vi "高压板校准程序1.2.vi"(8 "波特率":T3(ring)=enum."500Kbps", 9 "CAN路数":u16(ring) items=["0", "1"], 10 "设备索引":u16(ring) items=["0", "1", "2", "3", "4", "5", "6", "7", "8", "9", "10", "11", "12", "13", "14", "15", ""], 11 "CAN卡类型":u32(ring)=21 items=["PCI5121"=1, "PCI9810"=2, "USBCAN1"=3, "USBCAN2"=4, "PCI9820"=5, "PCI5110"=7, "CANLite(mini)"=8, "ISA9620"=9, "ISA5420"=10, "PC104CAN"=11, "DNP9810"=13, "PCI9840B"=14, "PC104C2"=15, "PCI9820I"=16, "pec9920"=18, "USBCAN_E_U"=20, "USBCAN_2E_U"=21]) -> (6 "E-U_baud":u32(ring)=393223 items=["0x060003--1000Kbps"=393219, "0x060004--800Kbps"=393220, "0x060007--500Kbps"=393223, "0x1C0008--250Kbps"=1835016, "0x1C0011--125Kbps"=1835025, "0x160023--100Kbps"=1441827, "0x1C002C--50Kbps"=1835052, "0x1600B3--20Kbps"=1441971, "0x1C00E0--10Kbps"=1835232, "0x1C01C1--5Kbps"=1835457])   [LabVIEW 2013]
uses:
  <vilib>/Instr/_visa.llb/VISA Configure Serial Port (Instr).vi
  <vilib>/Utility/config.llb/Write Key (String).vi
  <vilib>/Utility/file.llb/Read From Spreadsheet File (string).vi
  <vilib>/Utility/file.llb/Write To Spreadsheet File (string).vi
  <vilib>/Utility/config.llb/NI_LVConfig.lvlib
  data/kerneldlls/usbcan.dll
panel:
  in  "输出簇":T1
  out "Life":dbl
  out "分流器":enum32{"选项卡 1"}(tab)
  out "外总压":enum32{"选项卡 1"}(tab)
  out "内总压":enum32{"选项卡 1"}(tab)
  out "电流校正 2":enum32{"选项卡 1"}(tab)
  out "电流校正":enum32{"选项卡 1"}(tab)
  in  "Judge(%)":dbl=1.0
  in  "Judge(%)":dbl=0.5
  in  "记录":bool
  out "结果":i32(listbox)=-1
  in  "一键校正":bool
  in  "刷新":bool
  in  "分流器大小":T2(ring)=enum."300A"
  out "监控状态":bool
  out "电流":dbl format="%#.6f"
  out "外总压":dbl format="%#.6f"
  out "内总压":dbl format="%#.6f"
  in  "平均电压":dbl
  in  "电压增益":dbl
  in  "平均电流":dbl
  in  "电流增益":dbl
  in  "放电能量阀值":dbl=375.0
  in  "充电能量阀值":dbl=375.0
  in  "分流器型号":bool
  out "Current Gain结果 4":bool
  in  "充电能量阀值":bool
  out "Current Offset结果 4":bool
  in  "Set Current Gain 3":bool
  out "Current Gain结果 3":bool
  in  "Set Current Offset 3":bool
  out "Current Offset结果 3":bool
  out "Shunt Volt Gain":string
  out "Shunt Volt Offset":string
  in  "Set Current Gain 2":bool
  out "Current Gain结果 2":bool
  in  "Volt Offset":bool
  out "Current Offset结果 2":bool
  in  "导入配置结果":bool
  in  "读版本结果":bool
  in  "写版本结果":bool
  out "版本号-读":string
  in  "版本号":string
  in  "写配置文件版本":bool
  in  "读配置文件版本":bool
  in  "生成配置":bool
  in  "导入配置":bool
  out "config_data":string="000124FE00264205"
  out "充放电阈值":dbl=75006.0
  in  "连接状态 10":bool
  in  "设置参数":bool
  in  "安时分辨率/AH":u16(ring)=1 items=["0.001", "0.2"]
  in  "是否有外部高压":u16(ring)=1 items=["有", "无"]
  in  "分流器大小/A":u16(ring)=3 items=["50", "100", "200", "300", "400", "500", "600", "700", "800", "900", "1000"]
  in  "传感器类型":u16(ring)=1 items=["霍尔传感器", "分流器"]
  in  "电压分辨率/V":u16(ring)=1 items=["0.01", "0.1"]
  in  "电流分辨率/A":u16(ring)=1 items=["0.01", "0.1"]
  in  "Set":dbl
  in  "Volt2":dbl=300.0
  in  "Volt1":dbl=150.0
  in  "Clear":bool
  out "Clear结果":bool
  out "电流增益":string
  out "电流零点":string
  in  "Read1_in":bool
  out "Read1_in结果":bool
  in  "REAL1":dbl=150.0
  out "AD1":dbl
  in  "REAL2":dbl=300.0
  out "AD2":dbl
  in  "Offset":i32 format="%x"
  in  "Gain":dbl
  in  "REAL1":dbl=150.0
  in  "AD1":dbl
  in  "REAL2":dbl=300.0
  in  "AD2":dbl
  in  "Offset":i32 format="%x"
  in  "Gain":dbl
  in  "Read2_in":bool
  out "Read2_in结果":bool
  in  "Set_in":bool
  out "Set_in结果":bool
  in  "Read1_Out":bool
  out "Read1_Out结果":bool
  in  "Read2_Out":bool
  out "Read2_Out结果":bool
  in  "Set_out":bool
  out "Set_out结果":bool
  in  "Read1":bool
  out "Read1结果":bool
  in  "REAL1":dbl=40.0
  out "AD1":u16
  in  "REAL2":dbl=80.0
  out "AD2":u16
  in  "Gain":dbl
  in  "Read2":bool
  out "Read2结果":bool
  in  "Set":bool
  out "Set结果":bool
  in  "Set Current Gain":bool
  out "Current Gain结果":bool
  in  "Set Current Offset":bool
  out "Current Offset结果":bool
  in  "Clear_out":bool
  out "Clear_out结果":bool
  in  "Clear_in":bool
  out "Clear_in结果":bool
  in  "输出自定义值1":bool
  in  "输出自定义值2":bool
  out "Actual":dbl format="%#.6f"
  out "Set":dbl format="%#.6f"
  out "Actual":dbl
  in  "连接电压源":bool
  out "连接状态 10":bool
  in  "VISA resource name 4":refnum<visa-resource-name>="COM1" caption="设备端口号"
  in  "工作方式":u8(ring) items=["Normal", "Listen Only"]
  in  "滤波方式":u8(ring) items=["Dual Filter", "Single Filter"]
  out "CAN连接状态":bool
  in  "启动CAN连接":bool
  in  "VISA resource name 2":refnum<visa-resource-name>="GPIB0::5::INSTR" caption="设备端口号"
  out "连接状态 10":bool
  in  "连接GPIB":bool
  in  "Curr1":dbl=40.0
  in  "输出自定义值1 2":bool
  in  "输出自定义值2 2":bool
  in  "Curr2":dbl=80.0
  in  "退出":bool
  out "设置中？ 2":bool
  out "CAN状态 3":bool
  in  "设备索引 3":u16(ring) items=["0", "1", "2", "3", "4", "5", "6", "7", "8", "9", "10", "11", "12", "13", "14", "15", ""]
  in  "CAN路数 3":u16(ring) items=["0", "1"]
  in  "设备类型 3":u16(ring)=4 items=["PCI5121"=1, "PCI9810"=2, "USBCAN1"=3, "USBCAN2"=4, "PCI9820"=5, "CAN232"=6, "PCI5110"=7, "CANLite(mini)"=8, "ISA9620"=9, "ISA5420"=10, "PC104CAN"=11, "CANETE"=12, "DNP9810"=13]
  out "CAN 3":bool
  in  "停止 2":bool=TRUE
  out "监控 4":bool
  out "x-y":u32
  in  "退出程序 2":bool
  in  "error in (no error)":errorcluster caption="错误输入（无错误）"
  in  "控制读取  2":bool
  out "VISA资源名称输出":refnum<visa-resource-name>="0"
  in  "退出程序 3":bool
  in  "输出200A":bool
  out "实际值 2":dbl
  out "设定值 2":dbl
  in  "输出100A":bool
  in  "停止 7":bool=TRUE
  in  "分辨率偏移值 4":T4={"主板总电压分辨率"=0.01, "主板总电压偏移量"=0.0, "主板总电流分辨率"=0.01, "主板总电流偏移量"=-300.0, "主板安时分辨率"=0.2, "主板安时偏移量"=0.0, "主板SOC分辨率"=0.4, "主板SOC偏移量"=0.0, "从板总电压分辨率"=0.01, "从板总电压偏移量"=0.0, "从板总电流分辨率"=0.01, "从板总电流偏移量"=0.0, "从板安时分辨率"=0.2, "从板安时偏移量"=0.0, "从板SOC分辨率"=0.4, "从板SOC偏移量"=0.0, "功率分辨率"=0.01, "功率偏移量"=-300.0, "单体电压分辨率 "=0.0001, "单体电压偏移量"=0.0, "温度分辨率"=1.0, "温度偏移量"=-40.0, "高压板总电压分辨率"=0.01, "高压板总电压偏移量"=0.0, "高压板总电流分辨率"=0.01, "高压板总电流偏移量"=-300.0, "高压板安时分辨率"=0.2, "高压板安时偏移量"=0.0, "高压板SOC分辨率"=0.4, "高压板SOC偏移量"=0.0, "高压板功率分辨率"=0.01, "高压板功率偏移量"=-300.0}
  in  "分辨率偏移值 3":T4={"主板总电压分辨率"=0.01, "主板总电压偏移量"=0.0, "主板总电流分辨率"=0.01, "主板总电流偏移量"=-300.0, "主板安时分辨率"=0.2, "主板安时偏移量"=0.0, "主板SOC分辨率"=0.4, "主板SOC偏移量"=0.0, "从板总电压分辨率"=0.01, "从板总电压偏移量"=0.0, "从板总电流分辨率"=0.01, "从板总电流偏移量"=0.0, "从板安时分辨率"=0.2, "从板安时偏移量"=0.0, "从板SOC分辨率"=0.4, "从板SOC偏移量"=0.0, "功率分辨率"=0.01, "功率偏移量"=-300.0, "单体电压分辨率 "=0.0001, "单体电压偏移量"=0.0, "温度分辨率"=1.0, "温度偏移量"=-40.0, "高压板总电压分辨率"=0.01, "高压板总电压偏移量"=0.0, "高压板总电流分辨率"=0.01, "高压板总电流偏移量"=-300.0, "高压板安时分辨率"=0.2, "高压板安时偏移量"=0.0, "高压板SOC分辨率"=0.4, "高压板SOC偏移量"=0.0, "高压板功率分辨率"=0.01, "高压板功率偏移量"=-300.0}
  in  "监控":bool
  out "VCI_CAN_OBJ_R 2":T5={"ID"=0, "TimeStamp"=0, "TimeFlag"=0, "SendType"=1, "RemoteFlag"=0, "ExternFlag"=0, "DataLen"=8, 0, 0, 0, 0, 0, 0, 0, 0, 0, 0, 0}
  in  "分辨率偏移值":T6
  out "允许读取":bool
  out "设置中？":bool
  out "CAN状态 2":bool=TRUE
  in  "设备索引 2":u16(ring) items=["0", "1", "2", "3", "4", "5", "6", "7", "8", "9", "10", "11", "12", "13", "14", "15", ""]
  in  "CAN路数 2":u16(ring) items=["0", "1"]
  in  "设备类型 2":u16(ring)=4 items=["PCI5121"=1, "PCI9810"=2, "USBCAN1"=3, "USBCAN2"=4, "PCI9820"=5, "CAN232"=6, "PCI5110"=7, "CANLite(mini)"=8, "ISA9620"=9, "ISA5420"=10, "PC104CAN"=11, "CANETE"=12, "DNP9810"=13]
  out "CAN 2":bool
  in  "监控 2":bool
  in  "停止 6":bool=TRUE
  out "接收":T5={"ID"=67239966, "TimeStamp"=241409471, "TimeFlag"=1, "SendType"=250, "RemoteFlag"=0, "ExternFlag"=1, "DataLen"=8, 0, 0, 117, 48, 117, 48, 0, 0, 0, 0, 124} {"ID" format="%x"}
  in  "高压板信息":T7={"内部高压/V"=0.0, "Life"=10.0, "外部高压/V"=0.0, "power/KW"=0.0, "current/A"=0.0, "error code"=1, "SOC/%"=0.0, "总充电安时/AH"=0.0, "总放电安时/AH"=0.0, "平均电压"=0.0} {"平均电压" format="%.3f"; "总放电安时/AH" format="%#.3f"; "总充电安时/AH" format="%#.3f"; "SOC/%" format="%.3g"; "error code" format="%x"; "current/A" format="%.3g"; "power/KW" format="%#.3f"; "外部高压/V" format="%.3g"; "内部高压/V" format="%.3g"}
  in  "控制读取  5":bool
  out "VISA资源名称输出 10":refnum<visa-resource-name>
  in  "输出300V":bool
  out "电流/A 4":dbl
  in  "输出150V":bool
  in  "停止 3":bool=TRUE
  out "error out 3":errorcluster caption="error out"
  in  "错误输入（无错误）":errorcluster
  in  "控制读取  2":bool
  out "VISA资源名称输出 9":refnum<visa-resource-name>
  in  "退出程序":bool
  in  "输出80A":bool
  in  "输出40A":bool
  in  "控制读取  4":bool
  out "VISA资源名称输出 8":refnum<visa-resource-name>
  in  "连接状态 7":bool
  out "error out 2":errorcluster caption="error out"
  in  "控制读取  2":bool
  in  "连接状态 6":bool
  in  "控制读取  3":bool
  out "VISA资源名称输出 6":refnum<visa-resource-name>
  out "error out":errorcluster
  in  "控制读取  2":bool
  out "VISA资源名称输出 5":refnum<visa-resource-name>
  in  "电流值":dbl
  in  "自动控制仪器":bool=TRUE
  out "VISA资源名称输出 4":refnum<visa-resource-name>
  out "VISA资源名称输出 3":refnum<visa-resource-name>
  out "实际值 3":dbl format="%#.6f"
  out "设定值":dbl format="%#.6f"
  in  "控制读取  2":bool
  out "电流/A":dbl
  in  "控制读取":bool
  in  "Boar_Type":bool
  out "temp1":bool
  in  "总步骤":dbl=21.0
  in  "NG重测次数":dbl=3.0
  out "一键测试":bool
  out "测试结果":bool=TRUE
  in  "行号":dbl
  out "CAN状态":bool=TRUE
  out "CAN":bool
  in  "监控":bool=TRUE
  out "VCI_CAN_OBJ_R":T5={"ID"=0, "TimeStamp"=0, "TimeFlag"=0, "SendType"=1, "RemoteFlag"=0, "ExternFlag"=0, "DataLen"=8, 0, 0, 0, 0, 0, 0, 0, 0, 0, 0, 0}
  in  "停止":bool=TRUE
  # "重要参数设置"
  # "A"
  # "V"
  # "监控上位机"
  # "内总压"
  # "电流增益"
  # "AD2=AD1*2"
  # "外总压"
  # "BCU实时信息："
  # "BMS_Monitor"
  # "分辩率"
  # "偏移量"
  # "分辩率"
  # "偏移量"
  # "分辩率"
  # "偏移量"
  # "分辩率"
  # "偏移量"
  # "分辩率"
  # "偏移量"
  # "分辩率"
  # "偏移量"
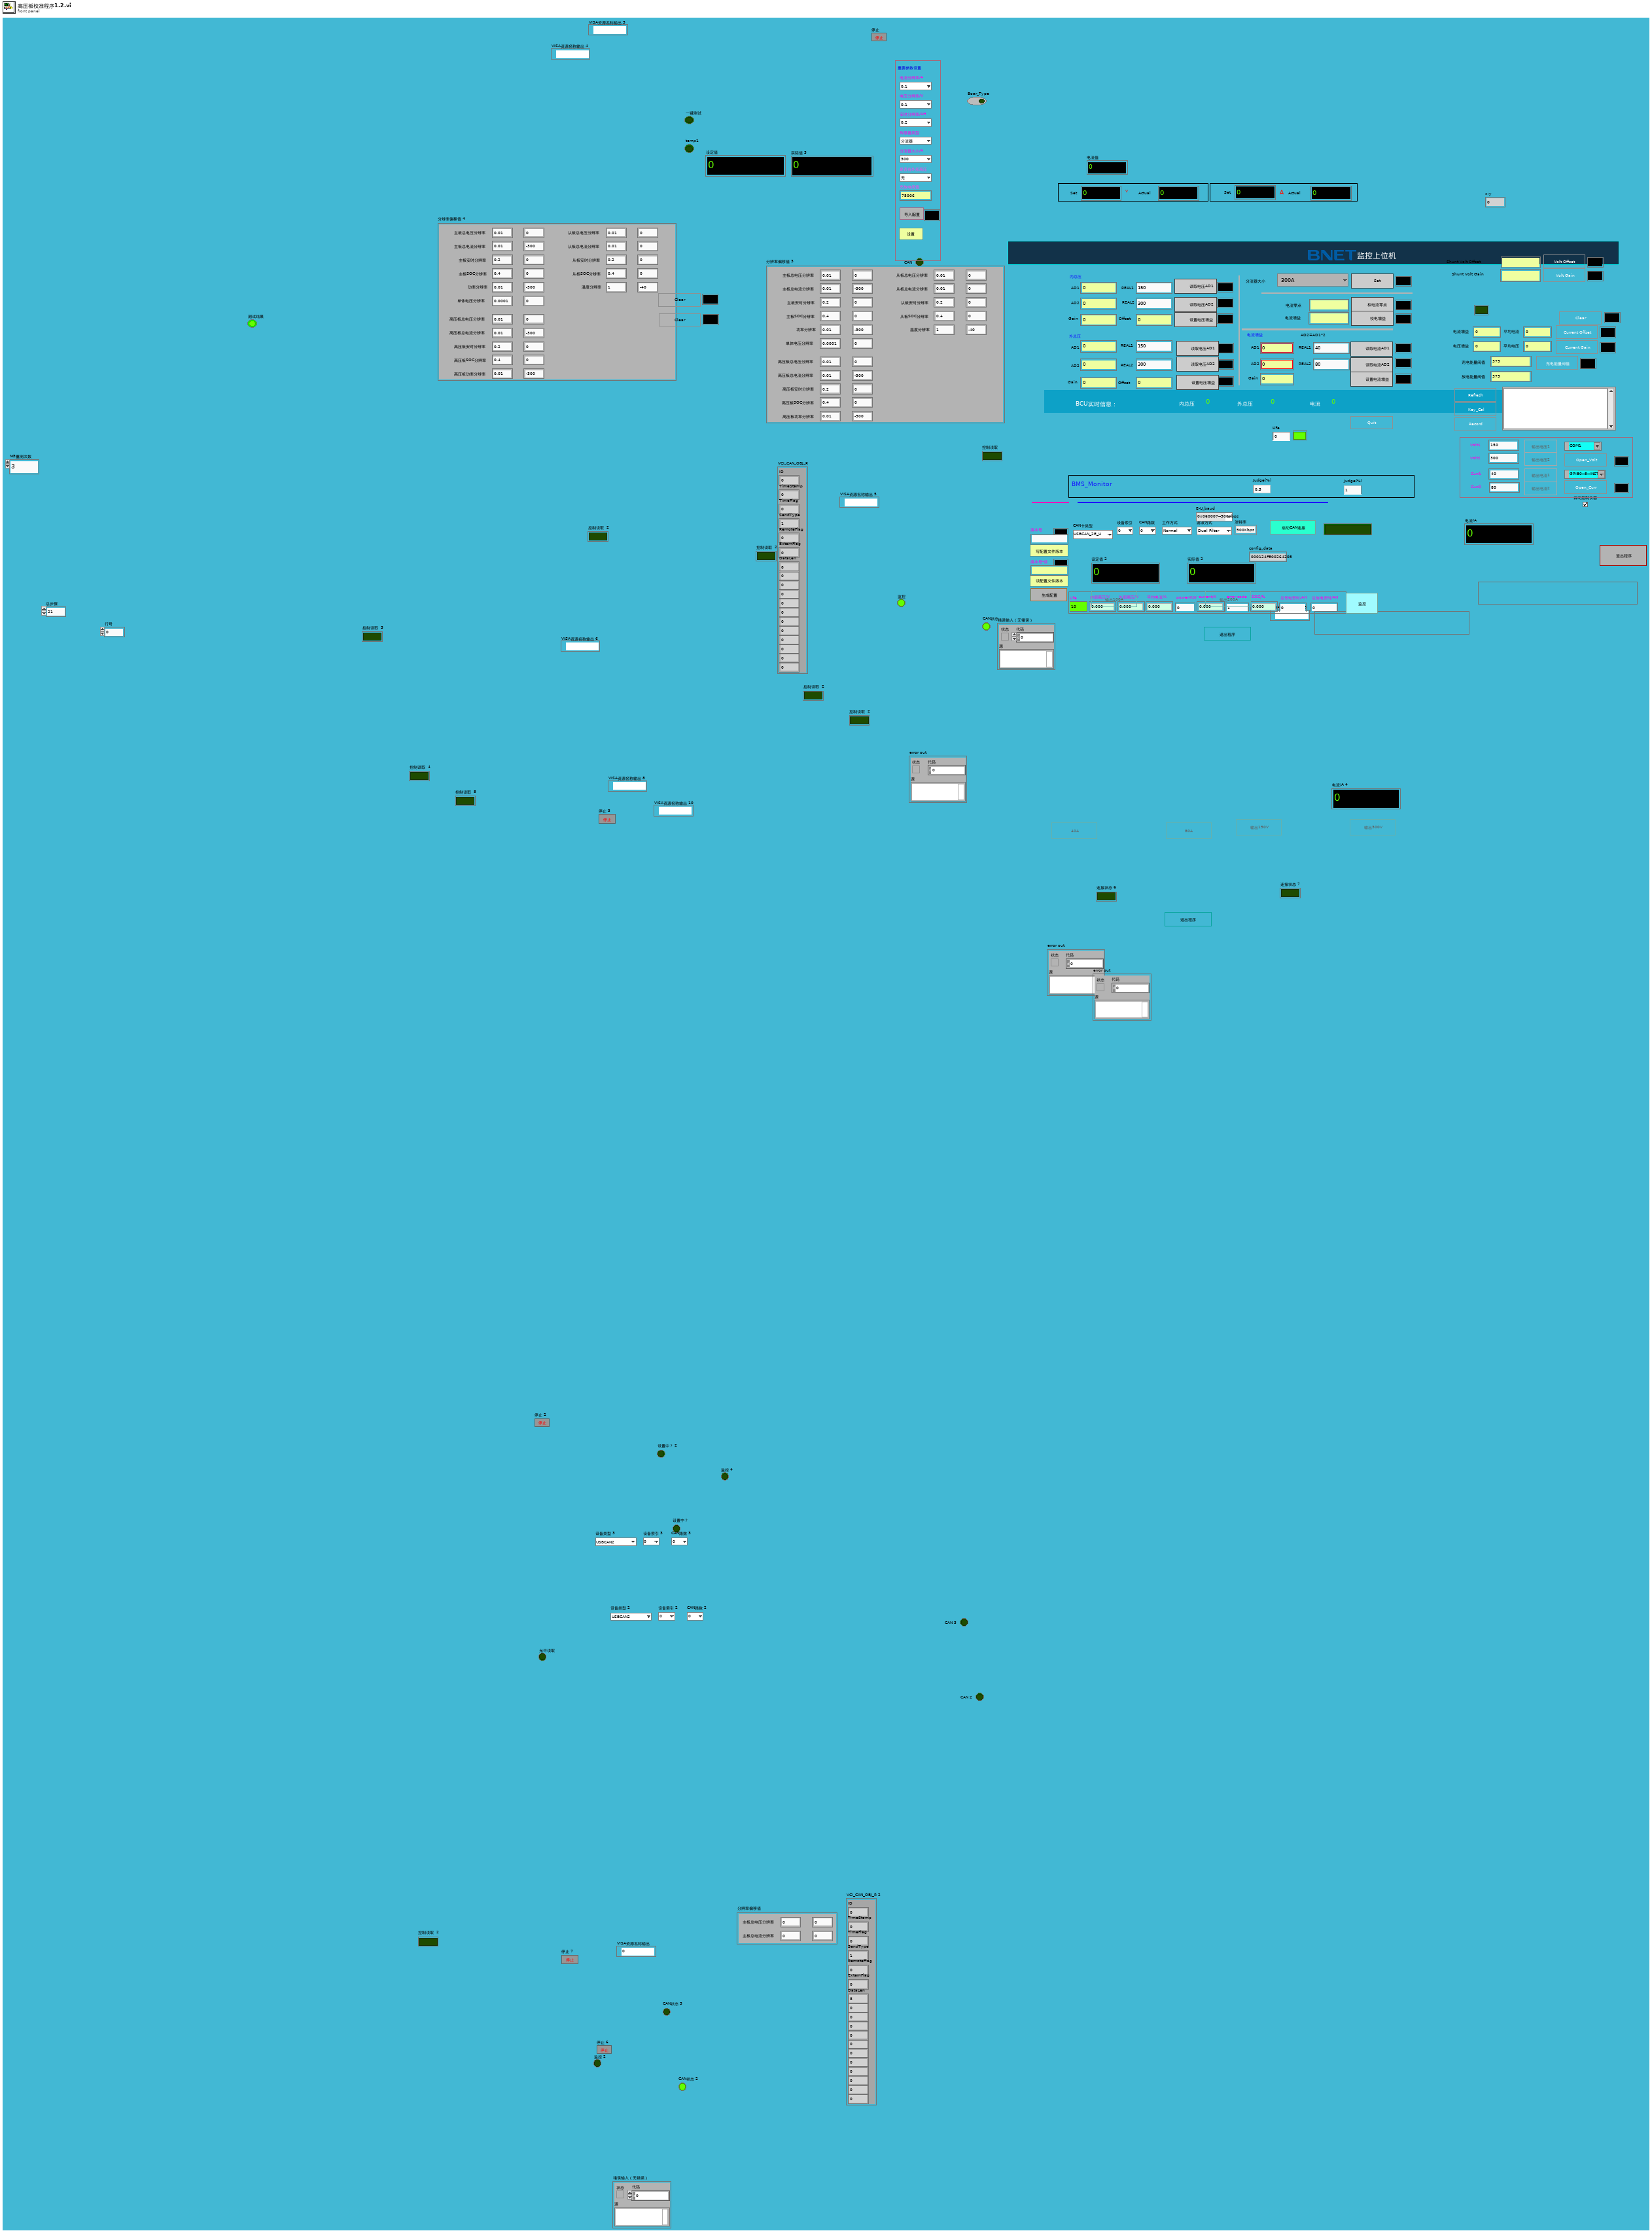
[diagram p1: front panel]
types:
  T1 = cluster{"return type":u32, "pReceive":cluster{"ID":u32, "TimeStamp":u32, "TimeFlag":u8, "SendType":u8, "RemoteFlag":u8, "ExternFlag":u8, "DataLen":u8, u8, u8, u8, u8, u8, u8, u8, u8, u8, u8, u8}[]}
  T2 = enum16{"选择分流器型号", "100A", "200A", "300A", "400A", "500A", "600A", "700A", "800A", "900A", "1000A"}
  T3 = enum16{"5Kbps", "10Kbps", "20Kbps", "40Kbps", "50Kbps", "80Kbps", "100Kbps", "125Kbps", "200Kbps", "250Kbps", "400Kbps", "500Kbps", "666Kbps", "800Kbps", "1000Kbps"}
  T4 = cluster{"主板总电压分辨率":dbl, "主板总电压偏移量":dbl, "主板总电流分辨率":dbl, "主板总电流偏移量":dbl, "主板安时分辨率":dbl, "主板安时偏移量":dbl, "主板SOC分辨率":dbl, "主板SOC偏移量":dbl, "从板总电压分辨率":dbl, "从板总电压偏移量":dbl, "从板总电流分辨率":dbl, "从板总电流偏移量":dbl, "从板安时分辨率":dbl, "从板安时偏移量":dbl, "从板SOC分辨率":dbl, "从板SOC偏移量":dbl, "功率分辨率":dbl, "功率偏移量":dbl, "单体电压分辨率 ":dbl, "单体电压偏移量":dbl, "温度分辨率":dbl, "温度偏移量":dbl, "高压板总电压分辨率":dbl, "高压板总电压偏移量":dbl, "高压板总电流分辨率":dbl, "高压板总电流偏移量":dbl, "高压板安时分辨率":dbl, "高压板安时偏移量":dbl, "高压板SOC分辨率":dbl, "高压板SOC偏移量":dbl, "高压板功率分辨率":dbl, "高压板功率偏移量":dbl}
  T5 = cluster{"ID":u32, "TimeStamp":u32, "TimeFlag":u8, "SendType":u8, "RemoteFlag":u8, "ExternFlag":u8, "DataLen":u8, u8, u8, u8, u8, u8, u8, u8, u8, u8, u8, u8}
  T6 = cluster{"主板总电压分辨率":dbl, "主板总电压偏移量":dbl, "主板总电流分辨率":dbl, "主板总电流偏移量":dbl, "主板安时分辨率":dbl, "主板安时偏移量":dbl, "主板SOC分辨率":dbl, "主板SOC偏移量":dbl, "从板总电压分辨率":dbl, "从板总电压偏移量":dbl, "从板总电流分辨率":dbl, "从板总电流偏移量":dbl, "从板安时分辨率":dbl, "从板安时偏移量":dbl, "从板SOC分辨率":dbl, "从板SOC偏移量":dbl, "功率分辨率":dbl, "功率偏移量":dbl, "单体电压分辨率 ":dbl, "单体电压偏移量":dbl, "温度分辨率":dbl, "温度偏移量":dbl}
  T7 = cluster{"内部高压/V":dbl, "Life":dbl, "外部高压/V":dbl, "power/KW":dbl, "current/A":dbl, "error code":u32, "SOC/%":dbl, "总充电安时/AH":dbl, "总放电安时/AH":dbl, "平均电压":dbl}
  T8 = enum16{"Set Current Offset", "Set Current Gain 4", "Set Current Gain", "Set Volt offset", "Set Volt Gain", "Set Current Offset 3", "Set Current Gain 3", "Set Current Offset 4", "Read", "Set", "Clear", "Read_in", "Set_in", "Clear_in", "Read_out", "Set_out", "Clear_out", "参数设置", "写配置文件版本", "读配置文件版本"}
  T9 = enum16{"Set Current Offset", "Set Current Gain", "Read", "Set", "Clear", "Read_in", "Set_in", "Clear_in", "Read_out", "Set_out", "Clear_out", "参数设置", "写配置文件版本", "读配置文件版本"}
  T10 = enum16{"Set Current Offset", "Set Current Gain", "Read", "Set", "Clear", "Read_in", "Set_in", "Clear_in", "Read_out", "Set_out", "Clear_out"}
  T11 = cluster{"ID":u32, "TimeStamp":u32, "TimeFlag":u8, "SendType":u8, "RemoteFlag":u8, "ExternFlag":u8, "DataLen":u8, u8, u8, u8, u8, u8, u8, u8, u8, u8, u8, u8}[]
  T12 = enum32{"Invalid", "Standard", "Closed", "Hidden", "Minimized", "Maximized"}
  T13 = typedef "NI_LVConfig.lvlib/Config Data RefNum.ctl" = refnum<k1>
  T14 = cluster{"return type":u32, "pReceive":cluster{"ID":u32, "TimeStamp":u32, "TimeFlag":u8, "SendType":u8, "RemoteFlag":u8, "ExternFlag":u8, "DataLen":u8, "1":u8, "2":u8, "3":u8, "4":u8, "5":u8, "6":u8, "7":u8, "8":u8, "9":u8, "10":u8, "11":u8}[]}
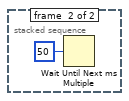
[diagram p4: hidden frame]
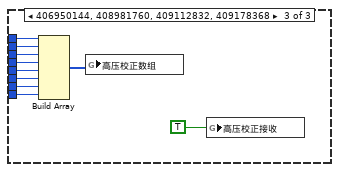
[diagram p6: hidden frame]
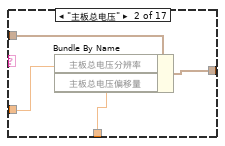
[diagram p9: hidden frame]
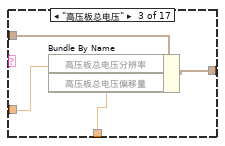
[diagram p10: hidden frame]
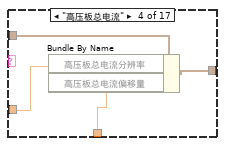
[diagram p11: hidden frame]
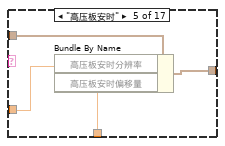
[diagram p12: hidden frame]
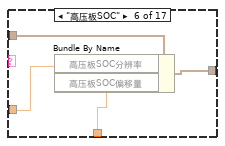
[diagram p13: hidden frame]
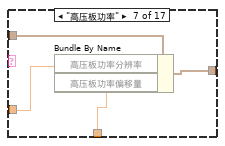
[diagram p14: hidden frame]
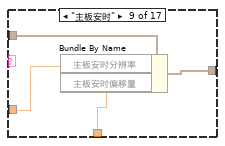
[diagram p15: hidden frame]
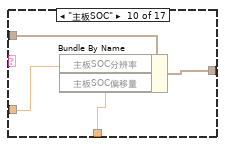
[diagram p16: hidden frame]
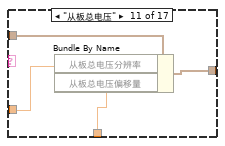
[diagram p17: hidden frame]
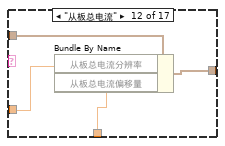
[diagram p18: hidden frame]
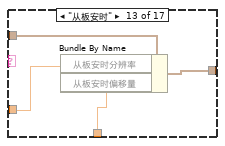
[diagram p19: hidden frame]
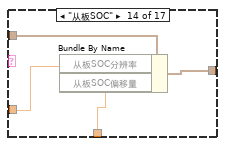
[diagram p20: hidden frame]
diagram:
  w18 = u32 0
  w35 = FALSE ("停止")
  w39 = u16 1 items=["霍尔传感器", "分流器"] ("传感器类型")
  w37 = cluster{u32, u32}[] [{0, 0}] ("颜色[4]")
  w36 = "" ("布尔文本.文本")
  w50 = u8 2 ("禁用")
  w46 = 0.0 ("电流/A")
  (unwired) "SET:GRO 1,10,1,1,0,0,0" ("写入缓冲区")
  w61 = u8 2 ("禁用")
  w45 = u8 2 ("禁用")
  (unwired) "SET:GRO 1,10,1,1,0,0,0" ("写入缓冲区")
  w68 = u8 0 ("禁用")
  w24 = cluster{u32, u32}[] [{0, 0}] ("颜色[4]")
  w23 = "" ("布尔文本.文本")
  (unwired) u8 2 ("禁用")
  (unwired) 20
  (unwired) u8 2 ("禁用")
  w69 = "Cmd" ("名称（未命名）")
  n1 = disable-structure shown="禁用" {
    frame Disabled {
      n2 = call "getpath.vi"() -> ("stripped path"=w77:path)  [unwired: 11 out]
      n3 = local read "分辨率偏移值 3"() -> (w74:T4)
      n4 = Build Path(base path=w77, name or relative path="Settings\\300以下分辨率偏移值.xls" ("名称或相对路径")) -> (appended path=w81:path)
      n5 = call-poly <vilib>:"Read From Spreadsheet File.vi"("file path (dialog if empty)"=w81) -> ("all rows"=w78:string[][])  [unwired: 3 in, 7 out]
      n6 = Delete From Array(array=w78, length=1 ("长度"), index (row)=0 ("索引")) -> (array with subset deleted=w75:string[][])  [unwired: 1 in, 1 out]
      n7 = for {
        tunnel: w75 -> [w90] mode=indexing
        shift-right: [w82] -> w73
        shift-left: w74 -> [w87]
        n8 = Index Array(array=w90, index #1=0 ("索引")) -> (element #1=w88:string, element #2=w86:string, element #3=w84:string)  [unwired: 2 in]
        n9 = Fract/Exp String To Number(string=w86) -> (number=w85:dbl)  [unwired: 4 out]
        n10 = Fract/Exp String To Number(string=w84) -> (number=w83:dbl)  [unwired: 4 out]
        n11 = case shown="\"主板总电流\"" w88 {
          tunnel: w87 -> [w91 w95 w99 w103 w107 w111 w115 w119 w123 w127 w131 w135 w139 w143 w147 w151 w155]
          tunnel: [w91 w94 w98 w102 w106 w110 w114 w118 w122 w126 w130 w134 w138 w142 w146 w150 w154] -> w82
          tunnel: w85 -> [_ w93 w97 w101 w105 w109 w113 w117 w121 w125 w129 w133 w137 w141 w145 w149 w153]
          tunnel: w83 -> [_ w92 w96 w100 w104 w108 w112 w116 w120 w124 w128 w132 w136 w140 w144 w148 w152]
          frame "假", Default {
          }
          frame "主板总电压" {
            n12 = Bundle By Name(cluster=w95, "主板总电压分辨率"=w93, "主板总电压偏移量"=w92) -> (w94:T4)
          }
          frame "高压板总电压" {
            n13 = Bundle By Name(cluster=w99, "高压板总电压分辨率"=w97, "高压板总电压偏移量"=w96) -> (w98:T4)
          }
          frame "高压板总电流" {
            n14 = Bundle By Name(cluster=w103, "高压板总电流分辨率"=w101, "高压板总电流偏移量"=w100) -> (w102:T4)
          }
          frame "高压板安时" {
            n15 = Bundle By Name(cluster=w107, "高压板安时分辨率"=w105, "高压板安时偏移量"=w104) -> (w106:T4)
          }
          frame "高压板SOC" {
            n16 = Bundle By Name(cluster=w111, "高压板SOC分辨率"=w109, "高压板SOC偏移量"=w108) -> (w110:T4)
          }
          frame "高压板功率" {
            n17 = Bundle By Name(cluster=w115, "高压板功率分辨率"=w113, "高压板功率偏移量"=w112) -> (w114:T4)
          }
          frame "主板总电流" {
            n18 = Bundle By Name(cluster=w119, "主板总电流分辨率"=w117, "主板总电流偏移量"=w116) -> (w118:T4)
          }
          frame "主板安时" {
            n19 = Bundle By Name(cluster=w123, "主板安时分辨率"=w121, "主板安时偏移量"=w120) -> (w122:T4)
          }
          frame "主板SOC" {
            n20 = Bundle By Name(cluster=w127, "主板SOC分辨率"=w125, "主板SOC偏移量"=w124) -> (w126:T4)
          }
          frame "从板总电压" {
            n21 = Bundle By Name(cluster=w131, "从板总电压分辨率"=w129, "从板总电压偏移量"=w128) -> (w130:T4)
          }
          frame "从板总电流" {
            n22 = Bundle By Name(cluster=w135, "从板总电流分辨率"=w133, "从板总电流偏移量"=w132) -> (w134:T4)
          }
          frame "从板安时" {
            n23 = Bundle By Name(cluster=w139, "从板安时分辨率"=w137, "从板安时偏移量"=w136) -> (w138:T4)
          }
          frame "从板SOC" {
            n24 = Bundle By Name(cluster=w143, "从板SOC分辨率"=w141, "从板SOC偏移量"=w140) -> (w142:T4)
          }
          frame "温度" {
            n25 = Bundle By Name(cluster=w147, "温度分辨率"=w145, "温度偏移量"=w144) -> (w146:T4)
          }
          frame "功率" {
            n26 = Bundle By Name(cluster=w151, "功率分辨率"=w149, "功率偏移量"=w148) -> (w150:T4)
          }
          frame "单体电压" {
            n27 = Bundle By Name(cluster=w155, "单体电压分辨率"=w153, "单体电压偏移量"=w152) -> (w154:T4)
          }
        }
      }
      n28 = local write "分辨率偏移值 3"(w73) -> ()
    }
    frame Enabled {
    }
  }
  n29 = stacked-sequence {
    tunnel: [w157 _] -> w19
    frame #0 {
      n30 = global read "EV05全局变量1.vi" "设备索引号"() -> (w159:u16)
      n31 = global read "EV05全局变量1.vi" "CAN卡类型"() -> (w160:u32)
      n32 = global read "EV05全局变量1.vi" "CAN端口"() -> (w158:u16)
      n33 = Build Array(1) -> (w161:i32[])
      n34 = call "transmit-8.6.vi"("can卡类型"=w160, "设备索引号"=w159, "CAN端口"=w158, "ID"=418398080, "SendType"=u8 0, "Data"=w161) -> ("错误输出"=w157:errorcluster)  [unwired: 3 in, 10 out]
    }
    frame #1 {
      n35 = Wait Until Next ms Multiple(millisecond multiple=u32 50 ("毫秒倍数")) -> ()  [unwired: 1 out]
    }
  }
  n36 = disable-structure shown="禁用" {
    frame Disabled {
      w171 = "MOSHI" ("section")
      n37 = call "getpath.vi"() -> ("stripped path"=w175:path)  [unwired: 11 out]
      n38 = Build Path(base path=w175, name or relative path="Settings\\EV03.ini" ("名称或相对路径")) -> (appended path=w173:path)
      n39 = call "Read&Write ini.vi"("功能"=enum16{"读取配置", "写入配置"}."读取配置", "configuration file path"=w173, "section"=w171, "key"=w171) -> ("key 4"=w170:string)  [unwired: 1 in, 10 out]
      n40 = Equal?(x=w170, y="1") -> (x = y?=w168:bool)
      n41 = Select(t=u8 0 ("禁用"), s=w168, f=u8 1 ("禁用")) -> (s? t:f=w165:u8)
      n42 = property on="电流分辨率/A" class="Ring (严格)"("Disabled"=w165) -> ()  [unwired: 2 in, 2 out]
      n43 = property on="电压分辨率/V" class="Ring (严格)"("Disabled"=w165) -> ()  [unwired: 2 in, 2 out]
      n44 = property on="是否有外部高压" class="Ring (严格)"("Disabled"=w165) -> ()  [unwired: 2 in, 2 out]
      n45 = property on="充放电阈值" class="DigNum (严格)"("Disabled"=w165) -> ()  [unwired: 2 in, 2 out]
      n46 = property on="传感器类型" class="Ring (严格)"("Disabled"=w165) -> ()  [unwired: 2 in, 2 out]
      n47 = property on="分流器大小/A" class="Ring (严格)"("Disabled"=w165) -> ()  [unwired: 2 in, 2 out]
      n48 = property on="安时分辨率/AH" class="Ring (严格)"("Disabled"=w165) -> ()  [unwired: 2 in, 2 out]
      n49 = property on="版本号" class="Str"("Disabled"=w165) -> ()  [unwired: 2 in, 2 out]
    }
    frame Enabled {
    }
  }
  n50 = local write "连接状态 10"(FALSE ("连接状态")) -> ()
  n51 = property on="输出150V" class="Bool"("Disabled"=w61) -> ()  [unwired: 2 in, 2 out]
  n52 = property on="输出300V" class="Bool"("Disabled"=w61) -> ()  [unwired: 2 in, 2 out]
  n53 = property on="输出自定义值2" class="Bool"("Disabled"=w61) -> ()  [unwired: 2 in, 2 out]
  n54 = property on="输出自定义值1" class="Bool"("Disabled"=w61) -> ()  [unwired: 2 in, 2 out]
  n55 = local write "VISA resource name 2"("GPIB0::5::INSTR" ("写入缓冲区")) -> ()
  n56 = local write "VISA资源名称输出 9"("" ("写入缓冲区")) -> ()
  n57 = local write "连接状态 10"(FALSE ("连接状态")) -> ()
  n58 = global read "EV05全局变量1.vi" "分流器型号"() -> (w1:T2)
  n59 = local write "连接状态 10"(FALSE ("设置_结果")) -> ()
  n60 = property on="Set_out" class="Bool (严格)"("Disabled"=w68) -> ()  [unwired: 2 in, 2 out]
  n61 = property on="Clear_in" class="Bool (严格)"("Disabled"=w68) -> ()  [unwired: 2 in, 2 out]
  n62 = property on="Set_in" class="Bool (严格)"("Disabled"=w68) -> ()  [unwired: 2 in, 2 out]
  n63 = local write "连接状态 10"(FALSE ("连接状态")) -> ()
  n64 = property on="Read2_Out" class="Bool (严格)"("Disabled"=w68) -> ()  [unwired: 2 in, 2 out]
  n65 = property on="Clear" class="Bool (严格)"("Disabled"=w68) -> ()  [unwired: 2 in, 2 out]
  n66 = local write "退出"(FALSE ("退出")) -> ()
  n67 = property on="输出40A" class="Bool"("Disabled"=w45) -> ()  [unwired: 2 in, 2 out]
  n68 = property on="输出80A" class="Bool"("Disabled"=w45) -> ()  [unwired: 2 in, 2 out]
  n69 = local write "NG重测次数"(3.0 ("NG重测次数")) -> ()
  n70 = property on="Read1_Out" class="Bool (严格)"("Disabled"=w68) -> ()  [unwired: 2 in, 2 out]
  n71 = property on="输出100A" class="Bool"("Disabled"=w50) -> ()  [unwired: 2 in, 2 out]
  n72 = property on="输出200A" class="Bool"("Disabled"=w50) -> ()  [unwired: 2 in, 2 out]
  n73 = property on="输出自定义值2 2" class="Bool"("Disabled"=w50) -> ()  [unwired: 2 in, 2 out]
  n74 = property on="输出自定义值1 2" class="Bool"("Disabled"=w50) -> ()  [unwired: 2 in, 2 out]
  n75 = property on="Set Current Gain" class="Bool (严格)"("Disabled"=w68) -> ()  [unwired: 2 in, 2 out]
  n76 = property on="Set Current Offset" class="Bool (严格)"("Disabled"=w68) -> ()  [unwired: 2 in, 2 out]
  n77 = property on="Read1_in" class="Bool (严格)"("Disabled"=w68) -> ()  [unwired: 2 in, 2 out]
  n78 = property on="Clear_out" class="Bool (严格)"("Disabled"=w68) -> ()  [unwired: 2 in, 2 out]
  n79 = local write "分流器大小"(w1) -> ()
  n80 = local write "Actual"(w46) -> ()
  n81 = global read "EV05全局变量1.vi" "设备索引号"() -> (w32:u16)
  n82 = global read "EV05全局变量1.vi" "CAN卡类型"() -> (w33:u32)
  n83 = local write "连接状态 10"(FALSE ("连接状态")) -> ()
  n84 = global read "EV05全局变量1.vi" "CAN端口"() -> (w34:u16)
  n85 = property on="Read2_in" class="Bool (严格)"("Disabled"=w68) -> ()  [unwired: 2 in, 2 out]
  n86 = property on="Set" class="Bool (严格)"("Disabled"=w68) -> ()  [unwired: 2 in, 2 out]
  n87 = property on="Read2" class="Bool (严格)"("Disabled"=w68) -> ()  [unwired: 2 in, 2 out]
  n88 = local write "Set"(w46) -> ()
  n89 = property on="Read1" class="Bool (严格)"("Disabled"=w68) -> ()  [unwired: 2 in, 2 out]
  n90 = local write "Curr1"(40.0 ("电流1（A）")) -> ()
  n91 = local write "Curr2"(80.0 ("电流2（A）")) -> ()
  n92 = local write "Volt1"(150.0 ("电压1 4")) -> ()
  n93 = local write "Volt2"(300.0 ("电压2 5")) -> ()
  n94 = local write "CAN卡类型"(w33) -> ()
  n95 = local write "CAN路数"(w34) -> ()
  n96 = local write "设备索引"(w32) -> ()
  n97 = Obtain Queue(name (unnamed)="CAN" ("名称（未命名）"), element data type="输出簇", error in (no error)="error in (no error)") -> (queue out=w7:refnum<queue>, error out=w41:errorcluster)  [unwired: 2 in, 1 out]
  n98 = local write "VISA资源名称输出"("0" ("写入缓冲区")) -> ()
  n99 = property on="读版本结果" class="Bool (严格)"("Colors [4]"=w37, "BoolText.Text"=w36) -> ()  [unwired: 2 in, 2 out]
  n100 = property on="写版本结果" class="Bool (严格)"("Colors [4]"=w37, "BoolText.Text"=w36) -> ()  [unwired: 2 in, 2 out]
  n101 = property on="导入配置结果" class="Bool (严格)"("Colors [4]"=w37, "BoolText.Text"=w36) -> ()  [unwired: 2 in, 2 out]
  n102 = property on="连接状态 10" class="Bool (严格)"("Colors [4]"=w37, "BoolText.Text"=w36) -> ()  [unwired: 2 in, 2 out]
  n103 = local write "版本号"("" ("版本号")) -> ()
  n104 = invoke on="监控" class="Bool" method="Reinit To Default"() -> ()  [unwired: 3 in, 3 out]
  n105 = local write "监控 2"(FALSE ("监控 2")) -> ()
  n106 = local write "传感器类型"(w39) -> ()
  n107 = Obtain Queue(name (unnamed)=w69, element data type=w69) -> (queue out=w44:refnum<queue>, error out=w43:errorcluster)  [unwired: 3 in, 1 out]
  n108 = while {
    tunnel: [w211] -> _
    tunnel: w19 -> [_]
    stop <- "停止 3" stop-if-true
    n109 = local read "连接状态 10"() -> (w214:bool)
    n110 = local read "控制读取  5"() -> (w215:bool)
    n111 = local read "Judge(%)"() -> (w210:dbl)
    n112 = local read "内总压"() -> (w205:dbl)
    n113 = local read "外总压"() -> (w203:dbl)
    n114 = local read "Actual"() -> (w198:dbl)
    n115 = And(x=w214, y=w215) -> (x .and. y?=w213:bool)
    n116 = case shown="真" w213 {
      tunnel: [_ w218] -> w212
      frame False {
      }
      frame True {
        n117 = local read "VISA资源名称输出 10"() -> (w235:refnum<visa-resource-name>)
        n118 = Concatenate Strings("MEA:ALL?" ("写入缓冲区"), "\n") -> (w232:string)
        n119 = VISA Write(VISA resource name=w235, write buffer=w232) -> (VISA resource name out=w234:refnum<visa-resource-name>, error out=w230:errorcluster)  [unwired: 1 in, 1 out]
        n120 = flat-sequence {
          tunnel: w234 -> [w238]
          tunnel: [w238] -> w229
          tunnel: [w236] -> w228
          tunnel: w230 -> [w236]
          tunnel: [w243] -> w227
          tunnel: [w242] -> w226
          tunnel: w229 -> [w241]
          tunnel: w228 -> [w240]
          tunnel: [w239] -> w225
          frame #0 {
            n121 = Wait (ms)(milliseconds to wait=u32 50 ("等待时间（毫秒）")) -> ()  [unwired: 1 out]
          }
          frame #1 {
            n122 = property class="Instr"(reference=w241, error in=w240) -> (reference out=w243:refnum<visa-resource-name>, error out=w239:errorcluster, "Serial Settings:Number of Bytes at Serial Port"=w242:u32)
          }
        }
        n123 = VISA Read(VISA resource name=w227, byte count=w226, error in (no error)=w225) -> (read buffer=w224:string, error out=w218:errorcluster)  [unwired: 2 out]
        n124 = Match Pattern(string=w224, regular expression="," ("正则表达式")) -> (before substring=w221:string, after substring=w222:string)  [unwired: 3 out]
        n125 = Fract/Exp String To Number(string=w221) -> (number=w220:dbl)  [unwired: 4 out]
        n126 = Fract/Exp String To Number(string=w222) -> (number=w219:dbl)  [unwired: 4 out]
        n127 = local write "电流/A 4"(w219) -> ()
        n128 = local write "Actual"(w220) -> ()
      }
    }
    n129 = Divide(x=w210, y=100.0) -> (x/y=w206:dbl)
    n130 = Add(x=1.0, y=w206) -> (x+y=w202:dbl)
    n131 = Subtract(x=1.0, y=w206) -> (x-y=w204:dbl)
    n132 = Multiply(x=w202, y=w198) -> (x*y=w192:dbl)
    n133 = Multiply(x=w204, y=w198) -> (x*y=w191:dbl)
    n134 = In Range and Coerce(upper limit=w192, x=w205, lower limit=w191) -> (In Range?=w201:bool)  [unwired: 1 out]
    n135 = In Range and Coerce(upper limit=w192, x=w203, lower limit=w191) -> (In Range?=w194:bool)  [unwired: 1 out]
    n136 = Select(t=u32 0, s=w201, f=u32 16711680) -> (s? t:f=w197:u32)
    n137 = Select(t=u32 0, s=w194, f=u32 16711680) -> (s? t:f=w193:u32)
    n138 = property on="内总压" class="DigNum (严格)"("NumText.BGColor"=w197) -> ()  [unwired: 2 in, 2 out]
    n139 = property on="外总压" class="DigNum (严格)"("NumText.BGColor"=w193) -> ()  [unwired: 2 in, 2 out]
    n140 = local read "Judge(%)"() -> (w185:dbl)
    n141 = local read "Actual"() -> (w186:dbl)
    n142 = Divide(x=w185, y=100.0) -> (x/y=w176:dbl)
    n143 = local read "电流"() -> (w180:dbl)
    n144 = Subtract(x=1.0, y=w176) -> (x-y=w188:dbl)
    n145 = Add(x=1.0, y=w176) -> (x+y=w190:dbl)
    n146 = Multiply(x=w188, y=w186) -> (x*y=w178:dbl)
    n147 = Multiply(x=w190, y=w186) -> (x*y=w179:dbl)
    n148 = In Range and Coerce(upper limit=w179, x=w180, lower limit=w178) -> (In Range?=w183:bool)  [unwired: 1 out]
    n149 = Wait (ms)(milliseconds to wait=u32 50 ("等待时间（毫秒）")) -> ()  [unwired: 1 out]
    n150 = Select(t=u32 0, s=w183, f=u32 16711680) -> (s? t:f=w177:u32)
    n151 = property on="电流" class="DigNum (严格)"("NumText.BGColor"=w177) -> ()  [unwired: 2 in, 2 out]
    n152 = call <vilib>:"Clear Errors.vi"("error in (no error)"=w212) -> ("error out"=w211:errorcluster)  [unwired: 6 out]
  }
  n153 = while {
    tunnel: w44 -> [w246]
    tunnel: w43 -> [w245]
    tunnel: w19 -> [_]
    stop <- w244 stop-if-true
    n154 = Dequeue Element(queue=w246, error in (no error)=w245) -> (queue out=w247:refnum<queue>, element=w248:string, error out=w244:errorcluster)  [unwired: 2 out]
    n155 = case shown="无错误" w244 {
      tunnel: w248 -> [w251 _]
      tunnel: w247 -> [w250 _]
      tunnel: w244 -> [w249 _]
      frame No Error {
        n156 = while {
          tunnel: w251 -> [w277]
          tunnel: w249 -> [_]
          tunnel: w250 -> [_]
          i -> [w275]
          stop <- w273 stop-if-true
          n157 = case shown="\"Set Current Gain 4\"" w277 {
            selector: w277 -> [w917 w921 w925 w929 w933 w939 w943 w947 w951 w955 w959 w963 w969 w975 w978 w982 w988 w994 w998 w1002 w1006 w1010 w1020 w1030]
            tunnel: ["" ("转换结果") "00" ("产品编号") "00" ("产品编号") "00" ("产品编号") "00" ("产品编号") w935 "00" ("产品编号") "00" ("产品编号") "00" ("产品编号") "00" ("产品编号") "00" ("产品编号") "00" ("产品编号") w965 w971 "2710" ("产品编号") w980 w985 w990 "000100000000" ("产品编号") "000100000000" ("产品编号") "00" ("产品编号") "00" ("产品编号") w1012 w1024] -> w271
            tunnel: [w917 w921 w925 w929 w933 w939 w943 w947 w951 w955 w959 w963 w969 w975 w978 w982 w988 w994 w998 w1002 w1006 w1010 w1020 w1030] -> w278
            tunnel: [enum16{"ASCII字符", "16进制字符"}."ASCII字符" ("传入类型") enum16{"ASCII字符", "16进制字符"}."16进制字符" ("传入类型") enum16{"ASCII字符", "16进制字符"}."16进制字符" ("传入类型") enum16{"ASCII字符", "16进制字符"}."16进制字符" ("传入类型") enum16{"ASCII字符", "16进制字符"}."16进制字符" ("传入类型") enum16{"ASCII字符", "16进制字符"}."16进制字符" ("传入类型") enum16{"ASCII字符", "16进制字符"}."16进制字符" ("传入类型") enum16{"ASCII字符", "16进制字符"}."16进制字符" ("传入类型") enum16{"ASCII字符", "16进制字符"}."16进制字符" ("传入类型") enum16{"ASCII字符", "16进制字符"}."16进制字符" ("传入类型") enum16{"ASCII字符", "16进制字符"}."16进制字符" ("传入类型") enum16{"ASCII字符", "16进制字符"}."16进制字符" ("传入类型") enum16{"ASCII字符", "16进制字符"}."16进制字符" ("传入类型") enum16{"ASCII字符", "16进制字符"}."16进制字符" ("传入类型") enum16{"ASCII字符", "16进制字符"}."16进制字符" ("传入类型") enum16{"ASCII字符", "16进制字符"}."16进制字符" ("传入类型") enum16{"ASCII字符", "16进制字符"}."ASCII字符" ("传入类型") enum16{"ASCII字符", "16进制字符"}."ASCII字符" ("传入类型") enum16{"ASCII字符", "16进制字符"}."16进制字符" ("传入类型") enum16{"ASCII字符", "16进制字符"}."16进制字符" ("传入类型") enum16{"ASCII字符", "16进制字符"}."16进制字符" ("传入类型") enum16{"ASCII字符", "16进制字符"}."16进制字符" ("传入类型") enum16{"ASCII字符", "16进制字符"}."16进制字符" ("传入类型") enum16{"ASCII字符", "16进制字符"}."16进制字符" ("传入类型")] -> w262
            tunnel: [_ T8."Read" ("校准命令") T8."Read_out" ("校准命令") T8."Read_out" ("校准命令") T8."Read" ("校准命令") T8."Set" ("校准命令") T8."Set Current Offset" ("校准命令") T8."Set Current Gain" ("校准命令") T8."Set Volt offset" ("校准命令") T8."Set Volt Gain" ("校准命令") T8."Set Current Offset 3" ("校准命令") T8."Set Current Gain 3" ("校准命令") T8."Set Current Offset 4" ("校准命令") T8."Set Current Gain 4" ("校准命令") _ T8."参数设置" ("校准命令") T8."写配置文件版本" ("校准命令") T9."读配置文件版本" ("校准命令") T10."Clear_in" ("校准命令") T10."Clear_out" ("校准命令") T8."Read_in" ("校准命令") T8."Read_in" ("校准命令") T8."Set_in" ("校准命令") T8."Set_out" ("校准命令")] -> w260
            frame "NULL", Default {
            }
            frame "Read1" {
            }
            frame "Read1_out" {
            }
            frame "Read2_out" {
            }
            frame "Read2" {
            }
            frame "Set" {
              n158 = local read "Gain"() -> (w937:dbl)
              n159 = Number To Hexadecimal String(1:i16 4 ("宽度(-)"), 2:w937) -> (0:w935:string)
            }
            frame "Set Current Offset" {
            }
            frame "Set Current Gain" {
            }
            frame "Set Volt offset" {
            }
            frame "Set Volt Gain" {
            }
            frame "Set Current Offset 3" {
            }
            frame "Set Current Gain 3" {
            }
            frame "Set Current Offset 4" {
              n160 = local read "充电能量阀值"() -> (w964:dbl)
              n161 = Number To Hexadecimal String(1:i16 8 ("宽度(-)"), 2:w964) -> (0:w965:string)
            }
            frame "Set Current Gain 4" {
              n162 = local read "分流器大小"() -> (w970:T2)
              n163 = Number To Hexadecimal String(1:i16 2 ("宽度(-)"), 2:w970) -> (0:w971:string)
            }
            frame "Clear" {
              (unwired) T8."Clear" ("校准命令")
            }
            frame "设置参数" {
              n164 = local read "config_data"() -> (w980:string)
            }
            frame "写配置文件版本" {
              n165 = local read "版本号"() -> (w984:string)
              n166 = String Subset(string=w984, length (rest)=8 ("长度（剩余）")) -> (substring=w985:string)  [unwired: 1 out]
            }
            frame "读配置文件版本" {
              n167 = local read "版本号"() -> (w989:string)
              n168 = String Subset(string=w989, length (rest)=8 ("长度（剩余）")) -> (substring=w990:string)  [unwired: 1 out]
            }
            frame "Clear_in" {
            }
            frame "Clear_out" {
            }
            frame "Read1_in" {
            }
            frame "Read2_in" {
            }
            frame "Set_in" {
              n169 = local read "Offset"() -> (w1017:i32)
              n170 = local read "Gain"() -> (w1018:dbl)
              n171 = Number To Hexadecimal String(1:i16 4 ("宽度(-)"), 2:w1018) -> (0:w1014:string)
              n172 = Number To Hexadecimal String(1:i16 8 ("宽度(-)"), 2:w1017) -> (0:w1013:string)
              n173 = Concatenate Strings(w1014, w1013) -> (w1012:string)
            }
            frame "Set_out" {
              n174 = local read "Offset"() -> (w1023:i32)
              n175 = local read "Gain"() -> (w1022:dbl)
              n176 = Number To Hexadecimal String(1:i16 4 ("宽度(-)"), 2:w1022) -> (0:w1026:string)
              n177 = Number To Hexadecimal String(1:i16 8 ("宽度(-)"), 2:w1023) -> (0:w1025:string)
              n178 = Concatenate Strings(w1026, w1025) -> (w1024:string)
            }
          }
          n179 = local read "CAN卡类型"() -> (w267:u32)
          n180 = disable-structure shown="禁用" {
            disable-tunnel: [w279 0.0 ("NG重测次数")] -> w276
            frame Disabled {
              n181 = local read "NG重测次数"() -> (w279:dbl)
            }
            frame Enabled {
            }
          }
          n182 = local read "滤波方式"() -> (w266:u8)
          n183 = local read "设备索引"() -> (w268:u16)
          n184 = local read "CAN路数"() -> (w269:u16)
          n185 = local read "工作方式"() -> (w265:u8)
          n186 = local read "波特率"() -> (w270:T3)
          n187 = call "高压板校正命令.vi"("CAN卡类型"=w267, "设备索引"=w268, "波特率"=w270, "CAN路数"=w269, "Data Input"=w271, "滤波方式"=w266, "传入类型"=w262, "工作方式"=w265, "校准命令"=w260) -> ("结果"=w264:bool, "添加的数组"=w259:u8[], "错误输出"=w253:errorcluster)  [unwired: 3 in, 5 out]
          n188 = Equal?(x=w276, y=w275) -> (x = y?=w274:bool)
          n189 = call <vilib>:"Clear Errors.vi"("error in (no error)"=w253) -> ()  [unwired: 7 out]
          n190 = Index Array(array=w259) -> (element #1=w254:u8, element #2=w258:u8, element #3=w257:u8, element #4=w256:u8, element #5=w255:u8)  [unwired: 5 in]
          n191 = case shown="\"Read1_in\"" w278 {
            tunnel: "" ("转换结果") -> [_ _ _ _ _ _ _ _ _ _ _ _ _ _ _ _ _ _ _ _ _ _ _ _]
            tunnel: ["跳过..." ("布尔文本.文本") w294 w327 w353 w379 w405 w432 w455 w477 w512 _ w574 w609 w644 w680 w713 w744 w767 w785 w803 w820 w841 w862 w876] -> _
            tunnel: [TRUE w283 w316 w342 w368 w394 w422 w445 w466 w502 w526 w562 w597 w632 w667 w700 w734 w757 w778 w796 w813 w831 w852 w872] -> w263
            tunnel: FALSE -> [_ w290 w323 w349 w375 w401 w428 w451 w473 w508 w535 w570 w605 w640 w676 w709 w740 w763 w781 w799 w816 w837 w858 w874]
            tunnel: w274 -> [_ w291 w324 w350 w376 w402 w429 w452 w474 w509 w536 w571 w606 w641 w677 w710 w741 w764 w782 w800 w817 w838 w859 w875]
            tunnel: w264 -> [_ w283 w316 w342 w368 w394 w422 w445 w466 w502 w526 w562 w597 w632 w667 w700 w734 w757 w778 w796 w813 w832 w853 w873]
            tunnel: w258 -> [_ w286 w319 w345 w371 w397 w425 w448 w469 w505 w531 w566 w601 w636 w671 w704 w737 w760 _ _ _ w830 w851 _]
            tunnel: w257 -> [_ w285 w318 w344 w370 w396 _ _ w468 _ w530 w565 w600 w635 w670 w703 _ _ _ _ _ _ _ _]
            tunnel: w256 -> [_ _ _ _ _ _ _ _ _ _ w529 w564 w599 w634 w669 w702 _ _ _ _ _ _ _ _]
            tunnel: w255 -> [_ _ _ _ _ _ _ _ _ _ w528 w563 w598 w633 w668 w701 _ _ _ _ _ _ _ _]
            tunnel: w254 -> [_ _ _ _ _ _ _ _ _ _ _ _ _ _ _ _ _ _ _ _ _ _ _ _]
            frame "NULL", Default {
              n192 = call <vilib>:"Unset Busy.vi"() -> ()  [unwired: 2 in, 10 out]
            }
            frame "Read1" {
              n193 = case shown="真" w283 {
                tunnel: [_ w300] -> w287
                tunnel: w286 -> [_ w299]
                tunnel: w285 -> [_ w298]
                frame False {
                }
                frame True {
                  n194 = Join Numbers(hi=w299, lo=w298) -> ((hi.lo)=w300:u16)
                }
              }
              n195 = disable-structure shown="禁用" {
                disable-tunnel: w287 -> [w301 _]
                frame Disabled {
                  w304 = 500.0 ("x")
                  n196 = local read "REAL1"() -> (w307:dbl)
                  n197 = Multiply(x=w307, y=100.0) -> (x*y=w305:dbl)
                  n198 = Add(x=w304, y=w305) -> (x+y=w303:dbl)
                  n199 = Subtract(x=w305, y=w304) -> (x-y=w302:dbl)
                  n200 = In Range and Coerce(upper limit=w303, x=w301, lower limit=w302) -> ()  [unwired: 2 out]
                }
                frame Enabled {
                }
              }
              n201 = global write "EV05全局变量1.vi" "CAN接收"(TRUE ("CAN接收")) -> ()
              n202 = case shown="假" w283 {
                tunnel: cluster{u32, u32}[] [{6618880, 6618880}] ("颜色[4]") -> [w312 _]
                tunnel: cluster{u32, u32}[] [{15663131, 6618880}] ("颜色[4]") -> [_ w315]
                tunnel: [w312 w315] -> w295
                tunnel: ["OK" ("布尔文本.文本") "NG" ("布尔文本.文本")] -> w294
                frame True {
                  n203 = call <vilib>:"Unset Busy.vi"() -> ()  [unwired: 2 in, 10 out]
                }
                frame False {
                  n204 = call <vilib>:"Unset Busy.vi"() -> ()  [unwired: 2 in, 10 out]
                }
              }
              n205 = Not(x=w290) -> (.not. x?=w293:bool)
              n206 = And(x=w283, y=w293) -> (x .and. y?=w292:bool)
              n207 = And(x=w293, y=w291) -> (x .and. y?=w289:bool)
              n208 = Or(x=w292, y=w289) -> (x .or. y?=w288:bool)
              n209 = case shown="真" w288 {
                tunnel: w295 -> [_ w311]
                tunnel: w294 -> [_ w310]
                tunnel: w287 -> [_ w309]
                frame False {
                }
                frame True {
                  n210 = local write "AD1"(w309) -> ()
                  n211 = property on="Read1结果" class="Bool (严格)"("Colors [4]"=w311, "BoolText.Text"=w310) -> (error out=w308:errorcluster)  [unwired: 2 in, 1 out]
                  n212 = call <vilib>:"Clear Errors.vi"("error in (no error)"=w308) -> ()  [unwired: 7 out]
                }
              }
            }
            frame "Read1_out" {
              n213 = case shown="真" w316 {
                tunnel: [_ w333] -> w320
                tunnel: w319 -> [_ w332]
                tunnel: w318 -> [_ w331]
                frame False {
                }
                frame True {
                  n214 = Join Numbers(hi=w332, lo=w331) -> ((hi.lo)=w333:u16)
                }
              }
              n215 = global write "EV05全局变量1.vi" "CAN接收"(TRUE ("CAN接收")) -> ()
              n216 = case shown="假" w316 {
                tunnel: cluster{u32, u32}[] [{6618880, 6618880}] ("颜色[4]") -> [w338 _]
                tunnel: cluster{u32, u32}[] [{15663131, 6618880}] ("颜色[4]") -> [_ w341]
                tunnel: [w338 w341] -> w328
                tunnel: ["OK" ("布尔文本.文本") "NG" ("布尔文本.文本")] -> w327
                frame True {
                  n217 = call <vilib>:"Unset Busy.vi"() -> ()  [unwired: 2 in, 10 out]
                }
                frame False {
                  n218 = call <vilib>:"Unset Busy.vi"() -> ()  [unwired: 2 in, 10 out]
                }
              }
              n219 = Not(x=w323) -> (.not. x?=w326:bool)
              n220 = And(x=w316, y=w326) -> (x .and. y?=w325:bool)
              n221 = And(x=w326, y=w324) -> (x .and. y?=w322:bool)
              n222 = Or(x=w325, y=w322) -> (x .or. y?=w321:bool)
              n223 = case shown="真" w321 {
                tunnel: w328 -> [_ w337]
                tunnel: w327 -> [_ w336]
                tunnel: w320 -> [_ w335]
                frame False {
                }
                frame True {
                  n224 = local write "AD1"(w335) -> ()
                  n225 = property on="Read1_Out结果" class="Bool (严格)"("Colors [4]"=w337, "BoolText.Text"=w336) -> (error out=w334:errorcluster)  [unwired: 2 in, 1 out]
                  n226 = call <vilib>:"Clear Errors.vi"("error in (no error)"=w334) -> ()  [unwired: 7 out]
                }
              }
            }
            frame "Read2_out" {
              n227 = case shown="真" w342 {
                tunnel: [_ w359] -> w346
                tunnel: w345 -> [_ w358]
                tunnel: w344 -> [_ w357]
                frame False {
                }
                frame True {
                  n228 = Join Numbers(hi=w358, lo=w357) -> ((hi.lo)=w359:u16)
                }
              }
              n229 = global write "EV05全局变量1.vi" "CAN接收"(TRUE ("CAN接收")) -> ()
              n230 = case shown="假" w342 {
                tunnel: cluster{u32, u32}[] [{6618880, 6618880}] ("颜色[4]") -> [w364 _]
                tunnel: cluster{u32, u32}[] [{15663131, 6618880}] ("颜色[4]") -> [_ w367]
                tunnel: [w364 w367] -> w354
                tunnel: ["OK" ("布尔文本.文本") "NG" ("布尔文本.文本")] -> w353
                frame True {
                  n231 = call <vilib>:"Unset Busy.vi"() -> ()  [unwired: 2 in, 10 out]
                }
                frame False {
                  n232 = call <vilib>:"Unset Busy.vi"() -> ()  [unwired: 2 in, 10 out]
                }
              }
              n233 = Not(x=w349) -> (.not. x?=w352:bool)
              n234 = And(x=w342, y=w352) -> (x .and. y?=w351:bool)
              n235 = And(x=w352, y=w350) -> (x .and. y?=w348:bool)
              n236 = Or(x=w351, y=w348) -> (x .or. y?=w347:bool)
              n237 = case shown="真" w347 {
                tunnel: w354 -> [_ w363]
                tunnel: w353 -> [_ w362]
                tunnel: w346 -> [_ w361]
                frame False {
                }
                frame True {
                  n238 = local write "AD2"(w361) -> ()
                  n239 = property on="Read2_Out结果" class="Bool (严格)"("Colors [4]"=w363, "BoolText.Text"=w362) -> (error out=w360:errorcluster)  [unwired: 2 in, 1 out]
                  n240 = call <vilib>:"Clear Errors.vi"("error in (no error)"=w360) -> ()  [unwired: 7 out]
                }
              }
            }
            frame "Read1_in" {
              n241 = case shown="真" w368 {
                tunnel: [_ w385] -> w372
                tunnel: w371 -> [_ w384]
                tunnel: w370 -> [_ w383]
                frame False {
                }
                frame True {
                  n242 = Join Numbers(hi=w384, lo=w383) -> ((hi.lo)=w385:u16)
                }
              }
              n243 = global write "EV05全局变量1.vi" "CAN接收"(TRUE ("CAN接收")) -> ()
              n244 = case shown="假" w368 {
                tunnel: cluster{u32, u32}[] [{6618880, 6618880}] ("颜色[4]") -> [w390 _]
                tunnel: cluster{u32, u32}[] [{15663131, 6618880}] ("颜色[4]") -> [_ w393]
                tunnel: [w390 w393] -> w380
                tunnel: ["OK" ("布尔文本.文本") "NG" ("布尔文本.文本")] -> w379
                frame True {
                  n245 = call <vilib>:"Unset Busy.vi"() -> ()  [unwired: 2 in, 10 out]
                }
                frame False {
                  n246 = call <vilib>:"Unset Busy.vi"() -> ()  [unwired: 2 in, 10 out]
                }
              }
              n247 = Not(x=w375) -> (.not. x?=w378:bool)
              n248 = And(x=w368, y=w378) -> (x .and. y?=w377:bool)
              n249 = And(x=w378, y=w376) -> (x .and. y?=w374:bool)
              n250 = Or(x=w377, y=w374) -> (x .or. y?=w373:bool)
              n251 = case shown="真" w373 {
                tunnel: w380 -> [_ w389]
                tunnel: w379 -> [_ w388]
                tunnel: w372 -> [_ w387]
                frame False {
                }
                frame True {
                  n252 = property on="Read1_in结果" class="Bool (严格)"("Colors [4]"=w389, "BoolText.Text"=w388) -> (error out=w386:errorcluster)  [unwired: 2 in, 1 out]
                  n253 = local write "AD1"(w387) -> ()
                  n254 = call <vilib>:"Clear Errors.vi"("error in (no error)"=w386) -> ()  [unwired: 7 out]
                }
              }
            }
            frame "Read2_in" {
              n255 = case shown="真" w394 {
                tunnel: [_ w411] -> w398
                tunnel: w397 -> [_ w410]
                tunnel: w396 -> [_ w409]
                frame False {
                }
                frame True {
                  n256 = Join Numbers(hi=w410, lo=w409) -> ((hi.lo)=w411:u16)
                }
              }
              n257 = global write "EV05全局变量1.vi" "CAN接收"(TRUE ("CAN接收")) -> ()
              n258 = case shown="假" w394 {
                tunnel: cluster{u32, u32}[] [{6618880, 6618880}] ("颜色[4]") -> [w416 _]
                tunnel: cluster{u32, u32}[] [{15663131, 6618880}] ("颜色[4]") -> [_ w419]
                tunnel: [w416 w419] -> w406
                tunnel: ["OK" ("布尔文本.文本") "NG" ("布尔文本.文本")] -> w405
                frame True {
                  n259 = call <vilib>:"Unset Busy.vi"() -> ()  [unwired: 2 in, 10 out]
                }
                frame False {
                  n260 = call <vilib>:"Unset Busy.vi"() -> ()  [unwired: 2 in, 10 out]
                }
              }
              n261 = Not(x=w401) -> (.not. x?=w404:bool)
              n262 = And(x=w394, y=w404) -> (x .and. y?=w403:bool)
              n263 = And(x=w404, y=w402) -> (x .and. y?=w400:bool)
              n264 = Or(x=w403, y=w400) -> (x .or. y?=w399:bool)
              n265 = case shown="真" w399 {
                tunnel: w406 -> [_ w415]
                tunnel: w405 -> [_ w414]
                tunnel: w398 -> [_ w413]
                frame False {
                }
                frame True {
                  n266 = local write "AD2"(w413) -> ()
                  n267 = property on="Read2_in结果" class="Bool (严格)"("Colors [4]"=w415, "BoolText.Text"=w414) -> (error out=w412:errorcluster)  [unwired: 2 in, 1 out]
                  n268 = call <vilib>:"Clear Errors.vi"("error in (no error)"=w412) -> ()  [unwired: 7 out]
                }
              }
            }
            frame "Set_in" {
              n269 = Equal?(x=w425, y=u8 1 ("x")) -> (x = y?=w423:bool)
              n270 = global write "EV05全局变量1.vi" "CAN接收"(TRUE ("CAN接收")) -> ()
              n271 = And(x=w423, y=w422) -> (x .and. y?=w421:bool)
              n272 = case shown="假" w421 {
                tunnel: cluster{u32, u32}[] [{6618880, 6618880}] ("颜色[4]") -> [w439 _]
                tunnel: cluster{u32, u32}[] [{15663131, 6618880}] ("颜色[4]") -> [_ w442]
                tunnel: [w439 w442] -> w433
                tunnel: ["OK" ("布尔文本.文本") "NG" ("布尔文本.文本")] -> w432
                frame True {
                  n273 = call <vilib>:"Unset Busy.vi"() -> ()  [unwired: 2 in, 10 out]
                }
                frame False {
                  n274 = call <vilib>:"Unset Busy.vi"() -> ()  [unwired: 2 in, 10 out]
                }
              }
              n275 = Not(x=w428) -> (.not. x?=w431:bool)
              n276 = And(x=w422, y=w431) -> (x .and. y?=w430:bool)
              n277 = And(x=w431, y=w429) -> (x .and. y?=w427:bool)
              n278 = Or(x=w430, y=w427) -> (x .or. y?=w426:bool)
              n279 = case shown="真" w426 {
                tunnel: w433 -> [_ w438]
                tunnel: w432 -> [_ w437]
                frame False {
                }
                frame True {
                  n280 = property on="Set_in结果" class="Bool (严格)"("Colors [4]"=w438, "BoolText.Text"=w437) -> (error out=w436:errorcluster)  [unwired: 2 in, 1 out]
                  n281 = call <vilib>:"Clear Errors.vi"("error in (no error)"=w436) -> ()  [unwired: 7 out]
                }
              }
            }
            frame "Set_out" {
              n282 = Equal?(x=w448, y=u8 1) -> (x = y?=w446:bool)
              n283 = global write "EV05全局变量1.vi" "CAN接收"(TRUE ("CAN接收")) -> ()
              n284 = And(x=w446, y=w445) -> (x .and. y?=w444:bool)
              n285 = case shown="假" w444 {
                tunnel: cluster{u32, u32}[] [{6618880, 6618880}] ("颜色[4]") -> [w462 _]
                tunnel: cluster{u32, u32}[] [{15663131, 6618880}] ("颜色[4]") -> [_ w465]
                tunnel: [w462 w465] -> w456
                tunnel: ["OK" ("布尔文本.文本") "NG" ("布尔文本.文本")] -> w455
                frame True {
                  n286 = call <vilib>:"Unset Busy.vi"() -> ()  [unwired: 2 in, 10 out]
                }
                frame False {
                  n287 = call <vilib>:"Unset Busy.vi"() -> ()  [unwired: 2 in, 10 out]
                }
              }
              n288 = Not(x=w451) -> (.not. x?=w454:bool)
              n289 = And(x=w445, y=w454) -> (x .and. y?=w453:bool)
              n290 = And(x=w454, y=w452) -> (x .and. y?=w450:bool)
              n291 = Or(x=w453, y=w450) -> (x .or. y?=w449:bool)
              n292 = case shown="真" w449 {
                tunnel: w456 -> [_ w461]
                tunnel: w455 -> [_ w460]
                frame False {
                }
                frame True {
                  n293 = property on="Set_out结果" class="Bool (严格)"("Colors [4]"=w461, "BoolText.Text"=w460) -> (error out=w459:errorcluster)  [unwired: 2 in, 1 out]
                  n294 = call <vilib>:"Clear Errors.vi"("error in (no error)"=w459) -> ()  [unwired: 7 out]
                }
              }
            }
            frame "Read2" {
              n295 = case shown="真" w466 {
                tunnel: [_ w483] -> w470
                tunnel: w469 -> [_ w482]
                tunnel: w468 -> [_ w481]
                frame False {
                }
                frame True {
                  n296 = Join Numbers(hi=w482, lo=w481) -> ((hi.lo)=w483:u16)
                }
              }
              n297 = disable-structure shown="禁用" {
                disable-tunnel: w470 -> [w485 _]
                frame Disabled {
                  w488 = 500.0 ("x")
                  n298 = local read "REAL2"() -> (w484:dbl)
                  n299 = Multiply(x=w484, y=100.0) -> (x*y=w489:dbl)
                  n300 = Add(x=w488, y=w489) -> (x+y=w487:dbl)
                  n301 = Subtract(x=w489, y=w488) -> (x-y=w486:dbl)
                  n302 = In Range and Coerce(upper limit=w487, x=w485, lower limit=w486) -> ()  [unwired: 2 out]
                }
                frame Enabled {
                }
              }
              n303 = global write "EV05全局变量1.vi" "CAN接收"(TRUE ("CAN接收")) -> ()
              n304 = case shown="假" w466 {
                tunnel: cluster{u32, u32}[] [{6618880, 6618880}] ("颜色[4]") -> [w495 _]
                tunnel: cluster{u32, u32}[] [{15663131, 6618880}] ("颜色[4]") -> [_ w498]
                tunnel: [w495 w498] -> w478
                tunnel: ["OK" ("布尔文本.文本") "NG" ("布尔文本.文本")] -> w477
                frame True {
                  n305 = call <vilib>:"Unset Busy.vi"() -> ()  [unwired: 2 in, 10 out]
                }
                frame False {
                  n306 = call <vilib>:"Unset Busy.vi"() -> ()  [unwired: 2 in, 10 out]
                }
              }
              n307 = Not(x=w473) -> (.not. x?=w476:bool)
              n308 = And(x=w466, y=w476) -> (x .and. y?=w475:bool)
              n309 = And(x=w476, y=w474) -> (x .and. y?=w472:bool)
              n310 = Or(x=w475, y=w472) -> (x .or. y?=w471:bool)
              n311 = case shown="真" w471 {
                tunnel: w478 -> [_ w494]
                tunnel: w477 -> [_ w493]
                tunnel: w470 -> [_ w492]
                frame False {
                }
                frame True {
                  n312 = local write "AD2"(w492) -> ()
                  n313 = property on="Read2结果" class="Bool (严格)"("Colors [4]"=w494, "BoolText.Text"=w493) -> (error out=w491:errorcluster)  [unwired: 2 in, 1 out]
                  n314 = call <vilib>:"Clear Errors.vi"("error in (no error)"=w491) -> ()  [unwired: 7 out]
                }
              }
            }
            frame "Set" {
              n315 = Equal?(x=w505, y=u8 1) -> (x = y?=w503:bool)
              n316 = disable-structure shown="禁用" {
                frame Disabled {
                  n317 = local read "Gain"() -> (w517:dbl)
                  n318 = In Range and Coerce(upper limit=100.0 ("上限"), x=w517, lower limit=94.0 ("上限")) -> (In Range?=w515:bool)  [unwired: 1 out]
                  n319 = And(x=w515, y=w515) -> ()  [unwired: 1 out]
                }
                frame Enabled {
                }
              }
              n320 = global write "EV05全局变量1.vi" "CAN接收"(TRUE ("CAN接收")) -> ()
              n321 = And(x=w503, y=w502) -> (x .and. y?=w501:bool)
              n322 = case shown="假" w501 {
                tunnel: cluster{u32, u32}[] [{6618880, 6618880}] ("颜色[4]") -> [w522 _]
                tunnel: cluster{u32, u32}[] [{15663131, 6618880}] ("颜色[4]") -> [_ w525]
                tunnel: [w522 w525] -> w513
                tunnel: ["OK" ("布尔文本.文本") "NG" ("布尔文本.文本")] -> w512
                frame True {
                  n323 = call <vilib>:"Unset Busy.vi"() -> ()  [unwired: 2 in, 10 out]
                }
                frame False {
                  n324 = call <vilib>:"Unset Busy.vi"() -> ()  [unwired: 2 in, 10 out]
                }
              }
              n325 = Not(x=w508) -> (.not. x?=w511:bool)
              n326 = And(x=w502, y=w511) -> (x .and. y?=w510:bool)
              n327 = And(x=w511, y=w509) -> (x .and. y?=w507:bool)
              n328 = Or(x=w510, y=w507) -> (x .or. y?=w506:bool)
              n329 = case shown="真" w506 {
                tunnel: w513 -> [_ w521]
                tunnel: w512 -> [_ w520]
                frame False {
                }
                frame True {
                  n330 = property on="Set结果" class="Bool (严格)"("Colors [4]"=w521, "BoolText.Text"=w520) -> (error out=w519:errorcluster)  [unwired: 2 in, 1 out]
                  n331 = call <vilib>:"Clear Errors.vi"("error in (no error)"=w519) -> ()  [unwired: 7 out]
                }
              }
            }
            frame "Set Current Offset" {
              n332 = case shown="假" w526 {
                tunnel: [_ w549] -> w532
                tunnel: w531 -> [_ w546]
                tunnel: w530 -> [_ w545]
                tunnel: w529 -> [_ w544]
                tunnel: w528 -> [_ w543]
                frame False {
                }
                frame True {
                  w548 = i16 2 ("宽度(-)")
                  n333 = Number To Hexadecimal String(1:w548, 2:w545) -> (0:w551:string)
                  n334 = Number To Hexadecimal String(1:w548, 2:w544) -> (0:w550:string)
                  n335 = Number To Hexadecimal String(1:w548, 2:w546) -> (0:w552:string)
                  n336 = Number To Hexadecimal String(1:w548, 2:w543) -> (0:w547:string)
                  n337 = Concatenate Strings(w552, w551, w550, w547) -> (w549:string)
                }
              }
              n338 = global write "EV05全局变量1.vi" "CAN接收"(TRUE ("CAN接收")) -> ()
              n339 = case shown="真" w526 {
                tunnel: cluster{u32, u32}[] [{6618880, 6618880}] ("颜色[4]") -> [w557 _]
                tunnel: cluster{u32, u32}[] [{15663131, 6618880}] ("颜色[4]") -> [_ w560]
                tunnel: [w557 w560] -> w540
                tunnel: ["OK" ("布尔文本.文本") "NG" ("布尔文本.文本")] -> w539
                frame True {
                  n340 = call <vilib>:"Unset Busy.vi"() -> ()  [unwired: 2 in, 10 out]
                }
                frame False {
                  n341 = call <vilib>:"Unset Busy.vi"() -> ()  [unwired: 2 in, 10 out]
                }
              }
              n342 = Not(x=w535) -> (.not. x?=w538:bool)
              n343 = And(x=w526, y=w538) -> (x .and. y?=w537:bool)
              n344 = And(x=w538, y=w536) -> (x .and. y?=w534:bool)
              n345 = Or(x=w537, y=w534) -> (x .or. y?=w533:bool)
              n346 = case shown="真" w533 {
                tunnel: w540 -> [_ w556]
                tunnel: w539 -> [_ w555]
                tunnel: w532 -> [_ w554]
                frame False {
                }
                frame True {
                  n347 = property on="Current Offset结果" class="Bool (严格)"("Colors [4]"=w556, "BoolText.Text"=w555) -> (error out=w553:errorcluster)  [unwired: 2 in, 1 out]
                  n348 = local write "电流零点"(w554) -> ()
                  n349 = call <vilib>:"Clear Errors.vi"("error in (no error)"=w553) -> ()  [unwired: 7 out]
                }
              }
            }
            frame "Set Current Gain" {
              n350 = case shown="真" w562 {
                tunnel: [_ w584] -> w567
                tunnel: w566 -> [_ w581]
                tunnel: w565 -> [_ w580]
                tunnel: w564 -> [_ w579]
                tunnel: w563 -> [_ w578]
                frame False {
                }
                frame True {
                  w583 = i16 2 ("宽度(-)")
                  n351 = Number To Hexadecimal String(1:w583, 2:w580) -> (0:w586:string)
                  n352 = Number To Hexadecimal String(1:w583, 2:w581) -> (0:w587:string)
                  n353 = Number To Hexadecimal String(1:w583, 2:w578) -> (0:w582:string)
                  n354 = Number To Hexadecimal String(1:w583, 2:w579) -> (0:w585:string)
                  n355 = Concatenate Strings(w587, w586, w585, w582) -> (w584:string)
                }
              }
              n356 = global write "EV05全局变量1.vi" "CAN接收"(TRUE ("CAN接收")) -> ()
              n357 = case shown="真" w562 {
                tunnel: cluster{u32, u32}[] [{6618880, 6618880}] ("颜色[4]") -> [w592 _]
                tunnel: cluster{u32, u32}[] [{15663131, 6618880}] ("颜色[4]") -> [_ w595]
                tunnel: [w592 w595] -> w575
                tunnel: ["OK" ("布尔文本.文本") "NG" ("布尔文本.文本")] -> w574
                frame True {
                  n358 = call <vilib>:"Unset Busy.vi"() -> ()  [unwired: 2 in, 10 out]
                }
                frame False {
                  n359 = call <vilib>:"Unset Busy.vi"() -> ()  [unwired: 2 in, 10 out]
                }
              }
              n360 = Not(x=w570) -> (.not. x?=w573:bool)
              n361 = And(x=w562, y=w573) -> (x .and. y?=w572:bool)
              n362 = And(x=w573, y=w571) -> (x .and. y?=w569:bool)
              n363 = Or(x=w572, y=w569) -> (x .or. y?=w568:bool)
              n364 = case shown="真" w568 {
                tunnel: w575 -> [_ w591]
                tunnel: w574 -> [_ w590]
                tunnel: w567 -> [_ w589]
                frame False {
                }
                frame True {
                  n365 = local write "电流增益"(w589) -> ()
                  n366 = property on="Current Gain结果" class="Bool (严格)"("Colors [4]"=w591, "BoolText.Text"=w590) -> (error out=w588:errorcluster)  [unwired: 2 in, 1 out]
                  n367 = call <vilib>:"Clear Errors.vi"("error in (no error)"=w588) -> ()  [unwired: 7 out]
                }
              }
            }
            frame "Set Volt offset" {
              n368 = case shown="真" w597 {
                tunnel: [_ w619] -> w602
                tunnel: w601 -> [_ w616]
                tunnel: w600 -> [_ w615]
                tunnel: w599 -> [_ w614]
                tunnel: w598 -> [_ w613]
                frame False {
                }
                frame True {
                  w618 = i16 2 ("宽度(-)")
                  n369 = Number To Hexadecimal String(1:w618, 2:w615) -> (0:w621:string)
                  n370 = Number To Hexadecimal String(1:w618, 2:w616) -> (0:w622:string)
                  n371 = Number To Hexadecimal String(1:w618, 2:w614) -> (0:w620:string)
                  n372 = Number To Hexadecimal String(1:w618, 2:w613) -> (0:w617:string)
                  n373 = Concatenate Strings(w622, w621, w620, w617) -> (w619:string)
                }
              }
              n374 = global write "EV05全局变量1.vi" "CAN接收"(TRUE ("CAN接收")) -> ()
              n375 = case shown="假" w597 {
                tunnel: cluster{u32, u32}[] [{6618880, 6618880}] ("颜色[4]") -> [w627 _]
                tunnel: cluster{u32, u32}[] [{15663131, 6618880}] ("颜色[4]") -> [_ w630]
                tunnel: [w627 w630] -> w610
                tunnel: ["OK" ("布尔文本.文本") "NG" ("布尔文本.文本")] -> w609
                frame True {
                  n376 = call <vilib>:"Unset Busy.vi"() -> ()  [unwired: 2 in, 10 out]
                }
                frame False {
                  n377 = call <vilib>:"Unset Busy.vi"() -> ()  [unwired: 2 in, 10 out]
                }
              }
              n378 = Not(x=w605) -> (.not. x?=w608:bool)
              n379 = And(x=w597, y=w608) -> (x .and. y?=w607:bool)
              n380 = And(x=w608, y=w606) -> (x .and. y?=w604:bool)
              n381 = Or(x=w607, y=w604) -> (x .or. y?=w603:bool)
              n382 = case shown="真" w603 {
                tunnel: w610 -> [_ w626]
                tunnel: w609 -> [_ w625]
                tunnel: w602 -> [_ w624]
                frame False {
                }
                frame True {
                  n383 = local write "Shunt Volt Offset"(w624) -> ()
                  n384 = property on="Current Offset结果 2" class="Bool (严格)"("Colors [4]"=w626, "BoolText.Text"=w625) -> (error out=w623:errorcluster)  [unwired: 2 in, 1 out]
                  n385 = call <vilib>:"Clear Errors.vi"("error in (no error)"=w623) -> ()  [unwired: 7 out]
                }
              }
            }
            frame "Set Volt Gain" {
              n386 = case shown="真" w632 {
                tunnel: [_ w654] -> w637
                tunnel: w636 -> [_ w651]
                tunnel: w635 -> [_ w650]
                tunnel: w634 -> [_ w649]
                tunnel: w633 -> [_ w648]
                frame False {
                }
                frame True {
                  w653 = i16 2 ("宽度(-)")
                  n387 = Number To Hexadecimal String(1:w653, 2:w649) -> (0:w655:string)
                  n388 = Number To Hexadecimal String(1:w653, 2:w648) -> (0:w652:string)
                  n389 = Number To Hexadecimal String(1:w653, 2:w650) -> (0:w656:string)
                  n390 = Number To Hexadecimal String(1:w653, 2:w651) -> (0:w657:string)
                  n391 = Concatenate Strings(w657, w656, w655, w652) -> (w654:string)
                }
              }
              n392 = global write "EV05全局变量1.vi" "CAN接收"(TRUE ("CAN接收")) -> ()
              n393 = case shown="假" w632 {
                tunnel: cluster{u32, u32}[] [{6618880, 6618880}] ("颜色[4]") -> [w662 _]
                tunnel: cluster{u32, u32}[] [{15663131, 6618880}] ("颜色[4]") -> [_ w665]
                tunnel: [w662 w665] -> w645
                tunnel: ["OK" ("布尔文本.文本") "NG" ("布尔文本.文本")] -> w644
                frame True {
                  n394 = call <vilib>:"Unset Busy.vi"() -> ()  [unwired: 2 in, 10 out]
                }
                frame False {
                  n395 = call <vilib>:"Unset Busy.vi"() -> ()  [unwired: 2 in, 10 out]
                }
              }
              n396 = Not(x=w640) -> (.not. x?=w643:bool)
              n397 = And(x=w632, y=w643) -> (x .and. y?=w642:bool)
              n398 = And(x=w643, y=w641) -> (x .and. y?=w639:bool)
              n399 = Or(x=w642, y=w639) -> (x .or. y?=w638:bool)
              n400 = case shown="真" w638 {
                tunnel: w645 -> [_ w661]
                tunnel: w644 -> [_ w660]
                tunnel: w637 -> [_ w659]
                frame False {
                }
                frame True {
                  n401 = local write "Shunt Volt Gain"(w659) -> ()
                  n402 = property on="Current Gain结果 2" class="Bool (严格)"("Colors [4]"=w661, "BoolText.Text"=w660) -> (error out=w658:errorcluster)  [unwired: 2 in, 1 out]
                  n403 = call <vilib>:"Clear Errors.vi"("error in (no error)"=w658) -> ()  [unwired: 7 out]
                }
              }
            }
            frame "Set Current Offset 3" {
              n404 = case shown="真" w667 {
                tunnel: [_ w689] -> w673
                tunnel: [_ w688] -> w672
                tunnel: w671 -> [_ w687]
                tunnel: w670 -> [_ w686]
                tunnel: w669 -> [_ w685]
                tunnel: w668 -> [_ w684]
                frame False {
                }
                frame True {
                  n405 = Join Numbers(hi=w687, lo=w686) -> ((hi.lo)=w689:u16)
                  n406 = Join Numbers(hi=w685, lo=w684) -> ((hi.lo)=w688:u16)
                }
              }
              n407 = global write "EV05全局变量1.vi" "CAN接收"(TRUE ("CAN接收")) -> ()
              n408 = case shown="假" w667 {
                tunnel: cluster{u32, u32}[] [{6618880, 6618880}] ("颜色[4]") -> [w695 _]
                tunnel: cluster{u32, u32}[] [{15663131, 6618880}] ("颜色[4]") -> [_ w698]
                tunnel: [w695 w698] -> w681
                tunnel: ["OK" ("布尔文本.文本") "NG" ("布尔文本.文本")] -> w680
                frame True {
                  n409 = call <vilib>:"Unset Busy.vi"() -> ()  [unwired: 2 in, 10 out]
                }
                frame False {
                  n410 = call <vilib>:"Unset Busy.vi"() -> ()  [unwired: 2 in, 10 out]
                }
              }
              n411 = Not(x=w676) -> (.not. x?=w679:bool)
              n412 = And(x=w667, y=w679) -> (x .and. y?=w678:bool)
              n413 = And(x=w679, y=w677) -> (x .and. y?=w675:bool)
              n414 = Or(x=w678, y=w675) -> (x .or. y?=w674:bool)
              n415 = case shown="真" w674 {
                tunnel: w681 -> [_ w694]
                tunnel: w680 -> [_ w693]
                tunnel: w673 -> [_ w692]
                tunnel: w672 -> [_ w691]
                frame False {
                }
                frame True {
                  n416 = property on="Current Offset结果 3" class="Bool (严格)"("Colors [4]"=w694, "BoolText.Text"=w693) -> (error out=w690:errorcluster)  [unwired: 2 in, 1 out]
                  n417 = local write "平均电流"(w691) -> ()
                  n418 = local write "电流增益"(w692) -> ()
                  n419 = call <vilib>:"Clear Errors.vi"("error in (no error)"=w690) -> ()  [unwired: 7 out]
                }
              }
            }
            frame "Set Current Gain 3" {
              n420 = case shown="真" w700 {
                tunnel: [_ w722] -> w706
                tunnel: [_ w721] -> w705
                tunnel: w704 -> [_ w720]
                tunnel: w703 -> [_ w719]
                tunnel: w702 -> [_ w718]
                tunnel: w701 -> [_ w717]
                frame False {
                }
                frame True {
                  n421 = Join Numbers(hi=w720, lo=w719) -> ((hi.lo)=w722:u16)
                  n422 = Join Numbers(hi=w718, lo=w717) -> ((hi.lo)=w721:u16)
                }
              }
              n423 = global write "EV05全局变量1.vi" "CAN接收"(TRUE ("CAN接收")) -> ()
              n424 = case shown="假" w700 {
                tunnel: cluster{u32, u32}[] [{6618880, 6618880}] ("颜色[4]") -> [w728 _]
                tunnel: cluster{u32, u32}[] [{15663131, 6618880}] ("颜色[4]") -> [_ w731]
                tunnel: [w728 w731] -> w714
                tunnel: ["OK" ("布尔文本.文本") "NG" ("布尔文本.文本")] -> w713
                frame True {
                  n425 = call <vilib>:"Unset Busy.vi"() -> ()  [unwired: 2 in, 10 out]
                }
                frame False {
                  n426 = call <vilib>:"Unset Busy.vi"() -> ()  [unwired: 2 in, 10 out]
                }
              }
              n427 = Not(x=w709) -> (.not. x?=w712:bool)
              n428 = And(x=w700, y=w712) -> (x .and. y?=w711:bool)
              n429 = And(x=w712, y=w710) -> (x .and. y?=w708:bool)
              n430 = Or(x=w711, y=w708) -> (x .or. y?=w707:bool)
              n431 = case shown="真" w707 {
                tunnel: w714 -> [_ w727]
                tunnel: w713 -> [_ w726]
                tunnel: w706 -> [_ w725]
                tunnel: w705 -> [_ w724]
                frame False {
                }
                frame True {
                  n432 = property on="Current Gain结果 3" class="Bool (严格)"("Colors [4]"=w727, "BoolText.Text"=w726) -> (error out=w723:errorcluster)  [unwired: 2 in, 1 out]
                  n433 = local write "电压增益"(w725) -> ()
                  n434 = local write "平均电压"(w724) -> ()
                  n435 = call <vilib>:"Clear Errors.vi"("error in (no error)"=w723) -> ()  [unwired: 7 out]
                }
              }
            }
            frame "Set Current Offset 4" {
              n436 = Equal?(x=w737, y=u8 1) -> (x = y?=w735:bool)
              n437 = global write "EV05全局变量1.vi" "CAN接收"(TRUE ("CAN接收")) -> ()
              n438 = And(x=w735, y=w734) -> (x .and. y?=w733:bool)
              n439 = case shown="假" w733 {
                tunnel: cluster{u32, u32}[] [{6618880, 6618880}] ("颜色[4]") -> [w751 _]
                tunnel: cluster{u32, u32}[] [{15663131, 6618880}] ("颜色[4]") -> [_ w754]
                tunnel: [w751 w754] -> w745
                tunnel: ["OK" ("布尔文本.文本") "NG" ("布尔文本.文本")] -> w744
                frame True {
                  n440 = call <vilib>:"Unset Busy.vi"() -> ()  [unwired: 2 in, 10 out]
                }
                frame False {
                  n441 = call <vilib>:"Unset Busy.vi"() -> ()  [unwired: 2 in, 10 out]
                }
              }
              n442 = Not(x=w740) -> (.not. x?=w743:bool)
              n443 = And(x=w734, y=w743) -> (x .and. y?=w742:bool)
              n444 = And(x=w743, y=w741) -> (x .and. y?=w739:bool)
              n445 = Or(x=w742, y=w739) -> (x .or. y?=w738:bool)
              n446 = case shown="真" w738 {
                tunnel: w745 -> [_ w750]
                tunnel: w744 -> [_ w749]
                frame False {
                }
                frame True {
                  n447 = property on="Current Offset结果 4" class="Bool (严格)"("Colors [4]"=w750, "BoolText.Text"=w749) -> (error out=w748:errorcluster)  [unwired: 2 in, 1 out]
                  n448 = call <vilib>:"Clear Errors.vi"("error in (no error)"=w748) -> ()  [unwired: 7 out]
                }
              }
            }
            frame "Set Current Gain 4" {
              n449 = Equal?(x=w760, y=u8 1) -> (x = y?=w758:bool)
              n450 = And(x=w758, y=w757) -> (x .and. y?=w756:bool)
              n451 = global write "EV05全局变量1.vi" "CAN接收"(TRUE ("CAN接收")) -> ()
              n452 = case shown="假" w756 {
                tunnel: cluster{u32, u32}[] [{6618880, 6618880}] ("颜色[4]") -> [w774 _]
                tunnel: cluster{u32, u32}[] [{15663131, 6618880}] ("颜色[4]") -> [_ w777]
                tunnel: [w774 w777] -> w768
                tunnel: ["OK" ("布尔文本.文本") "NG" ("布尔文本.文本")] -> w767
                frame True {
                  n453 = call <vilib>:"Unset Busy.vi"() -> ()  [unwired: 2 in, 10 out]
                }
                frame False {
                  n454 = call <vilib>:"Unset Busy.vi"() -> ()  [unwired: 2 in, 10 out]
                }
              }
              n455 = Not(x=w763) -> (.not. x?=w766:bool)
              n456 = And(x=w757, y=w766) -> (x .and. y?=w765:bool)
              n457 = And(x=w766, y=w764) -> (x .and. y?=w762:bool)
              n458 = Or(x=w765, y=w762) -> (x .or. y?=w761:bool)
              n459 = case shown="真" w761 {
                tunnel: w768 -> [_ w773]
                tunnel: w767 -> [_ w772]
                frame False {
                }
                frame True {
                  n460 = property on="Current Gain结果 4" class="Bool (严格)"("Colors [4]"=w773, "BoolText.Text"=w772) -> (error out=w771:errorcluster)  [unwired: 2 in, 1 out]
                  n461 = call <vilib>:"Clear Errors.vi"("error in (no error)"=w771) -> ()  [unwired: 7 out]
                }
              }
            }
            frame "Clear_in" {
              n462 = case shown="真" w778 {
                tunnel: cluster{u32, u32}[] [{6618880, 6618880}] ("颜色[4]") -> [w792 _]
                tunnel: cluster{u32, u32}[] [{15663131, 6618880}] ("颜色[4]") -> [_ w795]
                tunnel: [w792 w795] -> w786
                tunnel: ["OK" ("布尔文本.文本") "NG" ("布尔文本.文本")] -> w785
                frame True {
                }
                frame False {
                }
              }
              n463 = Not(x=w781) -> (.not. x?=w784:bool)
              n464 = And(x=w778, y=w784) -> (x .and. y?=w783:bool)
              n465 = And(x=w784, y=w782) -> (x .and. y?=w780:bool)
              n466 = Or(x=w783, y=w780) -> (x .or. y?=w779:bool)
              n467 = case shown="真" w779 {
                tunnel: w786 -> [_ w791]
                tunnel: w785 -> [_ w790]
                frame False {
                }
                frame True {
                  n468 = property on="Clear_in结果" class="Bool (严格)"("Colors [4]"=w791, "BoolText.Text"=w790) -> (error out=w789:errorcluster)  [unwired: 2 in, 1 out]
                  n469 = call <vilib>:"Clear Errors.vi"("error in (no error)"=w789) -> ()  [unwired: 7 out]
                }
              }
            }
            frame "Clear_out" {
              n470 = case shown="真" w796 {
                tunnel: cluster{u32, u32}[] [{6618880, 6618880}] ("颜色[4]") -> [w809 _]
                tunnel: cluster{u32, u32}[] [{15663131, 6618880}] ("颜色[4]") -> [_ w812]
                tunnel: [w809 w812] -> w804
                tunnel: ["OK" ("布尔文本.文本") "NG" ("布尔文本.文本")] -> w803
                frame True {
                }
                frame False {
                }
              }
              n471 = Not(x=w799) -> (.not. x?=w802:bool)
              n472 = And(x=w796, y=w802) -> (x .and. y?=w801:bool)
              n473 = And(x=w802, y=w800) -> (x .and. y?=w798:bool)
              n474 = Or(x=w801, y=w798) -> (x .or. y?=w797:bool)
              n475 = case shown="真" w797 {
                tunnel: w804 -> [_ w808]
                tunnel: w803 -> [_ w807]
                frame False {
                }
                frame True {
                  n476 = property on="Clear_out结果" class="Bool (严格)"("Colors [4]"=w808, "BoolText.Text"=w807) -> ()  [unwired: 2 in, 2 out]
                }
              }
            }
            frame "Clear" {
              n477 = case shown="真" w813 {
                tunnel: cluster{u32, u32}[] [{6618880, 6618880}] ("颜色[4]") -> [w826 _]
                tunnel: cluster{u32, u32}[] [{15663131, 6618880}] ("颜色[4]") -> [_ w829]
                tunnel: [w826 w829] -> w821
                tunnel: ["OK" ("布尔文本.文本") "NG" ("布尔文本.文本")] -> w820
                frame True {
                }
                frame False {
                }
              }
              n478 = Not(x=w816) -> (.not. x?=w819:bool)
              n479 = And(x=w813, y=w819) -> (x .and. y?=w818:bool)
              n480 = And(x=w819, y=w817) -> (x .and. y?=w815:bool)
              n481 = Or(x=w818, y=w815) -> (x .or. y?=w814:bool)
              n482 = case shown="真" w814 {
                tunnel: w821 -> [_ w825]
                tunnel: w820 -> [_ w824]
                frame False {
                }
                frame True {
                  n483 = property on="Clear结果" class="Bool (严格)"("Colors [4]"=w825, "BoolText.Text"=w824) -> ()  [unwired: 2 in, 2 out]
                }
              }
            }
            frame "设置参数" {
              n484 = Equal?(x=w830, y=u8 1) -> (x = y?=w833:bool)
              n485 = And(x=w833, y=w832) -> (x .and. y?=w831:bool)
              n486 = case shown="真" w831 {
                tunnel: cluster{u32, u32}[] [{6618880, 6618880}] ("颜色[4]") -> [w847 _]
                tunnel: cluster{u32, u32}[] [{15663131, 6618880}] ("颜色[4]") -> [_ w850]
                tunnel: [w847 w850] -> w842
                tunnel: ["OK" ("布尔文本.文本") "NG" ("布尔文本.文本")] -> w841
                frame True {
                }
                frame False {
                }
              }
              n487 = Not(x=w837) -> (.not. x?=w840:bool)
              n488 = And(x=w831, y=w840) -> (x .and. y?=w839:bool)
              n489 = And(x=w840, y=w838) -> (x .and. y?=w836:bool)
              n490 = Or(x=w839, y=w836) -> (x .or. y?=w835:bool)
              n491 = case shown="真" w835 {
                tunnel: w842 -> [_ w846]
                tunnel: w841 -> [_ w845]
                frame False {
                }
                frame True {
                  n492 = property on="连接状态 10" class="Bool (严格)"("Colors [4]"=w846, "BoolText.Text"=w845) -> ()  [unwired: 2 in, 2 out]
                }
              }
            }
            frame "写配置文件版本" {
              n493 = Equal?(x=w851, y=u8 1) -> (x = y?=w854:bool)
              n494 = And(x=w854, y=w853) -> (x .and. y?=w852:bool)
              n495 = case shown="真" w852 {
                tunnel: cluster{u32, u32}[] [{6618880, 6618880}] ("颜色[4]") -> [w868 _]
                tunnel: cluster{u32, u32}[] [{15663131, 6618880}] ("颜色[4]") -> [_ w871]
                tunnel: [w868 w871] -> w863
                tunnel: ["OK" ("布尔文本.文本") "NG" ("布尔文本.文本")] -> w862
                frame True {
                }
                frame False {
                }
              }
              n496 = Not(x=w858) -> (.not. x?=w861:bool)
              n497 = And(x=w852, y=w861) -> (x .and. y?=w860:bool)
              n498 = And(x=w861, y=w859) -> (x .and. y?=w857:bool)
              n499 = Or(x=w860, y=w857) -> (x .or. y?=w856:bool)
              n500 = case shown="真" w856 {
                tunnel: w863 -> [_ w867]
                tunnel: w862 -> [_ w866]
                frame False {
                }
                frame True {
                  n501 = property on="写版本结果" class="Bool (严格)"("Colors [4]"=w867, "BoolText.Text"=w866) -> ()  [unwired: 2 in, 2 out]
                }
              }
            }
            frame "读配置文件版本" {
              n502 = disable-structure shown="禁用" {
                disable-tunnel: [w886 _] -> w876
                disable-tunnel: w875 -> [w883 _]
                disable-tunnel: w874 -> [w882 _]
                disable-tunnel: w873 -> [w879 _]
                disable-tunnel: [w878 _] -> w872
                frame Disabled {
                  n503 = And(x=TRUE, y=w879) -> (x .and. y?=w878:bool)
                  n504 = case shown="真" w878 {
                    tunnel: cluster{u32, u32}[] [{6618880, 6618880}] ("颜色[4]") -> [w890 _]
                    tunnel: cluster{u32, u32}[] [{15663131, 6618880}] ("颜色[4]") -> [_ w893]
                    tunnel: [w890 w893] -> w887
                    tunnel: ["OK" ("布尔文本.文本") "NG" ("布尔文本.文本")] -> w886
                    frame True {
                    }
                    frame False {
                    }
                  }
                  n505 = Not(x=w882) -> (.not. x?=w885:bool)
                  n506 = And(x=w878, y=w885) -> (x .and. y?=w884:bool)
                  n507 = And(x=w885, y=w883) -> (x .and. y?=w881:bool)
                  n508 = Or(x=w884, y=w881) -> (x .or. y?=w880:bool)
                  n509 = case shown="真" w880 {
                    tunnel: w887 -> [_ w913]
                    tunnel: w886 -> [_ w912]
                    tunnel: _ -> [_ w914]
                    frame False {
                    }
                    frame True {
                      w911 = "" ("转换结果")
                      n510 = property on="读版本结果" class="Bool (严格)"("Colors [4]"=w913, "BoolText.Text"=w912) -> ()  [unwired: 2 in, 2 out]
                      n511 = Unbundle(w914) -> (w896, w897, w898, w899, w900, w901, w902, w903)  [unwired: 10 out]
                      n512 = Type Cast(type=w911, x=w902) -> (*(type *) &x=w909:string)
                      n513 = Type Cast(type=w911, x=w899) -> (*(type *) &x=w895:string)
                      n514 = Type Cast(type=w911, x=w896) -> (*(type *) &x=w904:string)
                      n515 = Type Cast(type=w911, x=w900) -> (*(type *) &x=w907:string)
                      n516 = Type Cast(type=w911, x=w901) -> (*(type *) &x=w908:string)
                      n517 = Type Cast(type=w911, x=w897) -> (*(type *) &x=w905:string)
                      n518 = Type Cast(type=w911, x=w898) -> (*(type *) &x=w906:string)
                      n519 = Type Cast(type=w911, x=w903) -> (*(type *) &x=w910:string)
                      n520 = Concatenate Strings(w904, w905, w906, w895, w907, w908, w909, w910) -> (w894:string)
                      n521 = local write "版本号-读"(w894) -> ()
                    }
                  }
                }
                frame Enabled {
                }
              }
            }
          }
          n522 = Or(x=w263, y=TRUE) -> (x .or. y?=w273:bool)
        }
      }
      frame Error {
      }
    }
  }
  n523 = while {
    tunnel: w19 -> [_]
    tunnel: w7 -> [w1033]
    stop <- "停止 2" stop-if-true
    n524 = Dequeue Element(queue=w1033) -> (element=w1031:T1, error out=w1032:errorcluster)  [unwired: 1 in, 3 out]
    n525 = case shown="无错误" w1032 {
      tunnel: w1031 -> [w1037 _]
      frame No Error {
        n526 = Unbundle(w1037) -> ("return type"=w1036:u32, "pReceive"=w1035:T11)
        n527 = for {
          N: w1036 -> [_]
          tunnel: w1035 -> [w1049] mode=indexing
          n528 = Unbundle(w1049) -> ("ID"=w1048:u32, w1047:u8, w1046:u8, w1045:u8, w1044:u8, w1043:u8, w1042:u8, w1039:u8, w1038:u8)  [unwired: 9 out]
          n529 = case shown="4019100" w1048 {
            tunnel: w1047 -> [_ w1059 w1075]
            tunnel: w1046 -> [_ w1058 w1074]
            tunnel: w1045 -> [_ w1057 w1073]
            tunnel: w1044 -> [_ w1056 w1072]
            tunnel: w1043 -> [_ w1055 w1071]
            tunnel: w1042 -> [_ w1054 w1070]
            tunnel: w1039 -> [_ _ w1069]
            tunnel: w1038 -> [_ w1050 w1068]
            frame 0, Default {
            }
            frame 67211520 {
              n530 = Join Numbers(hi=w1059, lo=w1058) -> ((hi.lo)=w1063:u16)
              n531 = Join Numbers(hi=w1057, lo=w1056) -> ((hi.lo)=w1062:u16)
              n532 = Join Numbers(hi=w1055, lo=w1054) -> ((hi.lo)=w1061:u16)
              n533 = call "输出分辨率计算.vi"("偏移量"=sgl -3000.0, "分辨率"=0.1, "数值 2"=w1062) -> ("输出2"=→"电流":dbl)  [unwired: 3 in, 5 out]
              n534 = call "输出分辨率计算.vi"("分辨率"=0.1, "数值 3"=w1061, "数值 2"=w1063) -> ("输出3"=→"外总压":dbl, "输出2"=→"内总压":dbl)  [unwired: 3 in, 4 out]
              "Life" <- w1050
            }
            frame 406950144, 408981760, 409112832, 409178368 {
              n535 = Build Array(w1075, w1074, w1073, w1072, w1071, w1070, w1069, w1068) -> (w1067:u8[])
              n536 = global write "EV05全局变量1.vi" "高压校正数组"(w1067) -> ()
              n537 = global write "EV05全局变量1.vi" "高压校正接收"(TRUE ("高压校正接收")) -> ()
            }
          }
          n538 = property on="监控状态" class="Bool (严格)"("Colors [4]"=cluster{u32, u32}[] [{6618880, 6618880}] ("颜色[4]")) -> (error out=w1040:errorcluster)  [unwired: 2 in, 1 out]
          n539 = call <vilib>:"Clear Errors.vi"("error in (no error)"=w1040) -> ()  [unwired: 7 out]
          "接收" <- w1049
        }
      }
      frame Error {
      }
    }
  }
  n540 = while {
    tunnel: w44 -> [w1081]
    tunnel: w43 -> [w1084]
    tunnel: [w1083] -> w31
    tunnel: [w1082] -> w30
    tunnel: w19 -> [_]
    stop <- w1076 stop-if-true
    n541 = local read "版本号"() -> (w1080:string)
    n542 = String Subset(string=w1080, length (rest)=8 ("长度（剩余）")) -> (substring=w1078:string)  [unwired: 1 out]
    n543 = local write "版本号"(w1078) -> ()
    n544 = event shown="[25] \"分流器型号\": 值改变" {
      selector: _ -> [_ _ _ _ _ _ _ _ _ _ _ _ _ _ _ _ _ _ _ _ _ _ _ _ _ _ _ _ _ _ _ _ _ _ _ _ _ _ _ _ _ _]
      dyn-events: _ -> [_ _ _ _ _ _ _ _ _ _ _ _ _ _ _ _ _ _ _ _ _ _ _ _ _ _ _ _ _ _ _ _ _ _ _ _ _ _ _ _ _ _]
      timeout: 100 -> [_ _ _ _ _ _ _ _ _ _ _ _ _ _ _ _ _ _ _ _ _ _ _ _ _ _ _ _ _ _ _ _ _ _ _ _ _ _ _ _ _ _]
      tunnel: w1081 -> [w1086 w1116 w1186 _ w1261 _ _ _ _ _ _ w3184 w3223 w3260 w3296 w3318 w3340 w3363 _ _ _ _ w3623 w3640 w3664 w3688 w3721 w3745 w3770 w3795 w3820 w3842 w3864 w3901 w3938 w3977 w4011 _ _ _ _ w4315]
      tunnel: w1084 -> [w1085 w1119 w1191 _ w1263 _ w2771 w2848 _ _ _ w3183 w3222 w3259 w3295 w3317 w3339 w3362 w3454 w3514 _ _ w3622 w3639 w3663 w3687 w3720 w3744 w3769 w3794 w3819 w3841 w3863 w3900 w3937 w3976 w4010 w4039 w4088 w4176 w4264 w4314]
      tunnel: [_ w1115 w1185 _ w1262 _ w2770 w2847 _ _ _ w3182 w3221 w3258 w3294 w3316 w3338 w3361 _ _ _ _ w3621 w3638 w3662 w3686 w3719 w3743 w3768 w3793 w3818 w3840 w3862 w3899 w3936 w3975 w4009 w4038 w4087 w4175 w4265 w4313] -> w1083
      tunnel: [_ w1116 w1186 _ w1260 _ _ _ _ _ _ w3181 w3220 w3257 w3293 w3315 w3337 w3360 _ _ _ _ w3620 w3637 w3661 w3685 w3718 w3742 w3767 w3792 w3817 w3839 w3861 w3898 w3935 w3974 w4008 _ _ _ _ w4312] -> w1082
      tunnel: [_ w1114 w1188 _ _ _ _ _ _ _ _ _ _ _ _ _ _ _ _ _ _ _ _ _ _ _ _ _ _ _ _ _ _ _ _ _ _ _ _ _ _ _] -> w1076
      event "启动CAN连接": Value Change {
        n545 = event-data() -> ("NewVal"=w1087:bool)  [unwired: 6 out]
        n546 = local write "监控"(w1087) -> ()
        n547 = local read "设备索引"() -> (w1092:u16)
        n548 = local read "CAN路数"() -> (w1090:u16)
        n549 = local read "CAN卡类型"() -> (w1093:u32)
        n550 = local read "波特率"() -> (w1091:T3)
        n551 = local read "滤波方式"() -> (w1089:u8)
        n552 = local read "工作方式"() -> (w1088:u8)
        n553 = case shown="假" w1087 {
          tunnel: w1093 -> [w1104 w1113]
          tunnel: w1092 -> [w1103 w1112]
          tunnel: w1091 -> [w1102 w1111]
          tunnel: w1090 -> [w1101 w1110]
          tunnel: w1089 -> [w1099 w1108]
          tunnel: w1088 -> [w1098 w1107]
          tunnel: w1086 -> [w1095 _]
          tunnel: w1085 -> [w1094 _]
          frame True {
            w1096 = u8 0 ("禁用")
            n554 = Flush Queue(queue=w1095, error in (no error)=w1094) -> ()  [unwired: 3 out]
            n555 = call "CAN_Init.vi"("设备类型"=w1104, "设备索引"=w1103, "波特率"=w1102, "CAN路数"=w1101, "操作类型"=enum16{"初始化CAN", "关闭CAN"}."初始化CAN", "滤波方式"=w1099, "工作方式"=w1098) -> ("CAN 操作结果"=w1097:bool)  [unwired: 3 in, 9 out]
            n556 = local write "CAN连接状态"(w1097) -> ()
            n557 = local write "CAN状态"(w1097) -> ()
            n558 = property on="Set_out" class="Bool (严格)"("Disabled"=w1096) -> ()  [unwired: 2 in, 2 out]
            n559 = property on="Clear_in" class="Bool (严格)"("Disabled"=w1096) -> ()  [unwired: 2 in, 2 out]
            n560 = property on="Set_in" class="Bool (严格)"("Disabled"=w1096) -> ()  [unwired: 2 in, 2 out]
            n561 = property on="Read2_Out" class="Bool (严格)"("Disabled"=w1096) -> ()  [unwired: 2 in, 2 out]
            n562 = property on="Clear" class="Bool (严格)"("Disabled"=w1096) -> ()  [unwired: 2 in, 2 out]
            n563 = property on="Read1_Out" class="Bool (严格)"("Disabled"=w1096) -> ()  [unwired: 2 in, 2 out]
            n564 = property on="Set Current Gain" class="Bool (严格)"("Disabled"=w1096) -> ()  [unwired: 2 in, 2 out]
            n565 = property on="Set Current Offset" class="Bool (严格)"("Disabled"=w1096) -> ()  [unwired: 2 in, 2 out]
            n566 = property on="Read1_in" class="Bool (严格)"("Disabled"=w1096) -> ()  [unwired: 2 in, 2 out]
            n567 = property on="Clear_out" class="Bool (严格)"("Disabled"=w1096) -> ()  [unwired: 2 in, 2 out]
            n568 = property on="Read2_in" class="Bool (严格)"("Disabled"=w1096) -> ()  [unwired: 2 in, 2 out]
            n569 = property on="Set" class="Bool (严格)"("Disabled"=w1096) -> ()  [unwired: 2 in, 2 out]
            n570 = property on="Read2" class="Bool (严格)"("Disabled"=w1096) -> ()  [unwired: 2 in, 2 out]
            n571 = property on="Read1" class="Bool (严格)"("Disabled"=w1096) -> ()  [unwired: 2 in, 2 out]
          }
          frame False {
            w1105 = u8 0 ("禁用")
            w1106 = FALSE ("CAN状态")
            n572 = call "CAN_Init.vi"("设备类型"=w1113, "设备索引"=w1112, "波特率"=w1111, "CAN路数"=w1110, "操作类型"=enum16{"初始化CAN", "关闭CAN"}."关闭CAN", "滤波方式"=w1108, "工作方式"=w1107) -> ()  [unwired: 3 in, 10 out]
            n573 = invoke on="监控" class="Bool" method="Reinit To Default"() -> ()  [unwired: 3 in, 3 out]
            n574 = local write "CAN连接状态"(w1106) -> ()
            n575 = local write "CAN状态"(w1106) -> ()
            n576 = property on="Set_out" class="Bool (严格)"("Disabled"=w1105) -> ()  [unwired: 2 in, 2 out]
            n577 = property on="Clear_in" class="Bool (严格)"("Disabled"=w1105) -> ()  [unwired: 2 in, 2 out]
            n578 = property on="Set_in" class="Bool (严格)"("Disabled"=w1105) -> ()  [unwired: 2 in, 2 out]
            n579 = property on="Read2_Out" class="Bool (严格)"("Disabled"=w1105) -> ()  [unwired: 2 in, 2 out]
            n580 = property on="Clear" class="Bool (严格)"("Disabled"=w1105) -> ()  [unwired: 2 in, 2 out]
            n581 = property on="Read1_Out" class="Bool (严格)"("Disabled"=w1105) -> ()  [unwired: 2 in, 2 out]
            n582 = property on="Set Current Gain" class="Bool (严格)"("Disabled"=w1105) -> ()  [unwired: 2 in, 2 out]
            n583 = property on="Set Current Offset" class="Bool (严格)"("Disabled"=w1105) -> ()  [unwired: 2 in, 2 out]
            n584 = property on="Read1_in" class="Bool (严格)"("Disabled"=w1105) -> ()  [unwired: 2 in, 2 out]
            n585 = property on="Clear_out" class="Bool (严格)"("Disabled"=w1105) -> ()  [unwired: 2 in, 2 out]
            n586 = property on="Read2_in" class="Bool (严格)"("Disabled"=w1105) -> ()  [unwired: 2 in, 2 out]
            n587 = property on="Set" class="Bool (严格)"("Disabled"=w1105) -> ()  [unwired: 2 in, 2 out]
            n588 = property on="Read2" class="Bool (严格)"("Disabled"=w1105) -> ()  [unwired: 2 in, 2 out]
            n589 = property on="Read1" class="Bool (严格)"("Disabled"=w1105) -> ()  [unwired: 2 in, 2 out]
          }
        }
      }
      event "退出": Value Change {
        n590 = event-data() -> ()  [unwired: 7 out]
        n591 = flat-sequence {
          tunnel: w1119 -> [w1122]
          tunnel: [w1125] -> w1118
          tunnel: [w1124] -> w1117
          tunnel: [w1123] -> w1114
          tunnel: w1118 -> [_]
          tunnel: w1117 -> [w1184]
          tunnel: [w1184] -> w1115
          frame #0 {
            w1123 = TRUE ("停止")
            n592 = disable-structure shown="禁用" {
              frame Disabled {
                n593 = local read "CAN卡类型"() -> (w1142:u32)
                n594 = local read "设备索引"() -> (w1141:u16)
                n595 = call "CAN_Init.vi"("设备类型"=w1142, "设备索引"=w1141, "操作类型"=enum16{"初始化CAN", "关闭CAN"}."关闭CAN") -> ()  [unwired: 7 in, 10 out]
              }
              frame Enabled {
              }
            }
            n596 = local write "停止"(w1123) -> ()
            n597 = local write "停止 3"(w1123) -> ()
            n598 = local write "停止 2"(w1123) -> ()
            n599 = local write "停止 6"(w1123) -> ()
            n600 = local write "停止 7"(w1123) -> ()
            n601 = local read "VISA资源名称输出 10"() -> (w1128:refnum<visa-resource-name>)
            n602 = local read "VISA资源名称输出"() -> (w1133:refnum<visa-resource-name>)
            n603 = flat-sequence {
              tunnel: w1128 -> [w1147]
              tunnel: [w1147] -> w1132
              tunnel: w1122 -> [w1145]
              tunnel: [w1144] -> w1120
              tunnel: w1132 -> [w1150]
              tunnel: [w1150] -> w1131
              tunnel: [w1148] -> w1121
              tunnel: w1120 -> [w1148]
              tunnel: w1131 -> [w1154]
              tunnel: [w1153] -> w1130
              tunnel: [w1152] -> w1129
              tunnel: w1121 -> [w1151]
              tunnel: [w1157] -> w1126
              tunnel: [w1158] -> w1127
              tunnel: w1130 -> [w1158]
              tunnel: w1129 -> [w1157]
              frame #0 {
                n604 = VISA Write(VISA resource name=w1147, write buffer="OUT:OFF" ("写入缓冲区"), error in (no error)=w1145) -> (error out=w1144:errorcluster)  [unwired: 2 out]
              }
              frame #1 {
                n605 = Wait (ms)(milliseconds to wait=u32 50 ("等待时间（毫秒）")) -> ()  [unwired: 1 out]
              }
              frame #2 {
                n606 = VISA Write(VISA resource name=w1154, write buffer="OUT:OFF" ("写入缓冲区"), error in (no error)=w1151) -> (VISA resource name out=w1153:refnum<visa-resource-name>, error out=w1152:errorcluster)  [unwired: 1 out]
              }
              frame #3 {
                n607 = Wait (ms)(milliseconds to wait=u32 50 ("等待时间（毫秒）")) -> ()  [unwired: 1 out]
              }
            }
            n608 = flat-sequence {
              tunnel: w1133 -> [w1159]
              tunnel: [w1159] -> w1140
              tunnel: w1140 -> [w1161]
              tunnel: [w1161] -> w1139
              tunnel: w1139 -> [w1166]
              tunnel: [w1165] -> w1138
              tunnel: [w1164] -> w1137
              tunnel: [w1163] -> w1136
              tunnel: w1122 -> [w1162]
              tunnel: [w1169] -> w1135
              tunnel: [w1168] -> w1134
              tunnel: w1138 -> [w1171]
              tunnel: w1137 -> [w1170]
              tunnel: w1136 -> [w1167]
              frame #0 {
              }
              frame #1 {
                n609 = Wait (ms)(milliseconds to wait=u32 50 ("等待时间（毫秒）")) -> ()  [unwired: 1 out]
              }
              frame #2 {
                w1163 = "outp off" ("写入缓冲区")
                n610 = VISA Write(VISA resource name=w1166, write buffer=w1163, error in (no error)=w1162) -> (VISA resource name out=w1165:refnum<visa-resource-name>, error out=w1164:errorcluster)  [unwired: 1 out]
              }
              frame #3 {
                n611 = VISA Write(VISA resource name=w1171, write buffer=w1167, error in (no error)=w1170) -> (VISA resource name out=w1168:refnum<visa-resource-name>, error out=w1169:errorcluster)  [unwired: 1 out]
                n612 = Wait (ms)(milliseconds to wait=u32 50 ("等待时间（毫秒）")) -> ()  [unwired: 1 out]
              }
            }
            n613 = VISA Close(VISA resource name=w1134, error in (no error)=w1135) -> (error out=w1125:errorcluster)
            n614 = VISA Close(VISA resource name=w1127, error in (no error)=w1126) -> (error out=w1124:errorcluster)
          }
          frame #1 {
            n615 = global read "EV05全局变量1.vi" "设备索引号"() -> (w1179:u16)
            n616 = global read "EV05全局变量1.vi" "CAN卡类型"() -> (w1180:u32)
            n617 = global read "EV05全局变量1.vi" "CAN端口"() -> (w1178:u16)
            n618 = property class="VI"("FP.State"=T12."Hidden" ("前面板窗口:状态")) -> (reference out=w1176:refnum<vi>, error out=w1177:errorcluster)  [unwired: 2 in]
            n619 = Build Array(7) -> (w1181:i32[])
            n620 = call "transmit-8.6.vi"("can卡类型"=w1180, "设备索引号"=w1179, "CAN端口"=w1178, "ID"=418398080, "SendType"=u8 0, "Data"=w1181) -> ()  [unwired: 3 in, 11 out]
            n621 = property class="VI"(reference=w1176, error in=w1177, "Front Panel.Open"=FALSE ("前面板窗口:打开")) -> ()  [unwired: 2 out]
          }
        }
      }
      event Panel Close? {
        n622 = event-data() -> ()  [unwired: 5 out]
        n623 = flat-sequence {
          tunnel: w1191 -> [w1194]
          tunnel: [w1193] -> w1190
          tunnel: [w1192] -> w1189
          tunnel: w1190 -> [_]
          tunnel: w1189 -> [w1247]
          tunnel: [w1247] -> w1185
          tunnel: [w1246] -> w1188
          frame #0 {
            n624 = local read "VISA资源名称输出 10"() -> (w1197:refnum<visa-resource-name>)
            n625 = local read "VISA资源名称输出"() -> (w1202:refnum<visa-resource-name>)
            n626 = flat-sequence {
              tunnel: w1197 -> [w1210]
              tunnel: [w1210] -> w1201
              tunnel: w1201 -> [w1212]
              tunnel: [w1212] -> w1200
              tunnel: w1200 -> [w1216]
              tunnel: [w1215] -> w1199
              tunnel: [w1214] -> w1198
              tunnel: w1194 -> [w1213]
              tunnel: [w1219] -> w1195
              tunnel: [w1220] -> w1196
              tunnel: w1199 -> [w1220]
              tunnel: w1198 -> [w1219]
              frame #0 {
              }
              frame #1 {
                n627 = Wait (ms)(milliseconds to wait=u32 120 ("等待时间（毫秒）")) -> ()  [unwired: 1 out]
              }
              frame #2 {
                n628 = VISA Write(VISA resource name=w1216, write buffer="OUT:OFF" ("写入缓冲区"), error in (no error)=w1213) -> (VISA resource name out=w1215:refnum<visa-resource-name>, error out=w1214:errorcluster)  [unwired: 1 out]
              }
              frame #3 {
                n629 = Wait (ms)(milliseconds to wait=u32 50 ("等待时间（毫秒）")) -> ()  [unwired: 1 out]
              }
            }
            n630 = flat-sequence {
              tunnel: w1202 -> [w1221]
              tunnel: [w1221] -> w1209
              tunnel: w1209 -> [w1223]
              tunnel: [w1223] -> w1208
              tunnel: w1208 -> [w1228]
              tunnel: [w1227] -> w1207
              tunnel: [w1226] -> w1206
              tunnel: [w1225] -> w1205
              tunnel: w1194 -> [w1224]
              tunnel: [w1231] -> w1204
              tunnel: [w1230] -> w1203
              tunnel: w1207 -> [w1233]
              tunnel: w1206 -> [w1232]
              tunnel: w1205 -> [w1229]
              frame #0 {
              }
              frame #1 {
                n631 = Wait (ms)(milliseconds to wait=u32 120 ("等待时间（毫秒）")) -> ()  [unwired: 1 out]
              }
              frame #2 {
                w1225 = "outp off" ("写入缓冲区")
                n632 = VISA Write(VISA resource name=w1228, write buffer=w1225, error in (no error)=w1224) -> (VISA resource name out=w1227:refnum<visa-resource-name>, error out=w1226:errorcluster)  [unwired: 1 out]
              }
              frame #3 {
                n633 = VISA Write(VISA resource name=w1233, write buffer=w1229, error in (no error)=w1232) -> (VISA resource name out=w1230:refnum<visa-resource-name>, error out=w1231:errorcluster)  [unwired: 1 out]
                n634 = Wait (ms)(milliseconds to wait=u32 50 ("等待时间（毫秒）")) -> ()  [unwired: 1 out]
              }
            }
            n635 = VISA Close(VISA resource name=w1203, error in (no error)=w1204) -> (error out=w1193:errorcluster)
            n636 = VISA Close(VISA resource name=w1196, error in (no error)=w1195) -> (error out=w1192:errorcluster)
          }
          frame #1 {
            w1246 = TRUE ("停止")
            n637 = global read "EV05全局变量1.vi" "设备索引号"() -> (w1241:u16)
            n638 = global read "EV05全局变量1.vi" "CAN卡类型"() -> (w1242:u32)
            n639 = global read "EV05全局变量1.vi" "CAN端口"() -> (w1240:u16)
            n640 = property class="VI"("FP.State"=T12."Hidden" ("前面板窗口:状态")) -> (reference out=w1238:refnum<vi>, error out=w1239:errorcluster)  [unwired: 2 in]
            n641 = Build Array(7) -> (w1243:i32[])
            n642 = local write "停止"(w1246) -> ()
            n643 = call "transmit-8.6.vi"("can卡类型"=w1242, "设备索引号"=w1241, "CAN端口"=w1240, "ID"=418398080, "SendType"=u8 0, "Data"=w1243) -> ()  [unwired: 3 in, 11 out]
            n644 = local write "停止 3"(w1246) -> ()
            n645 = local write "停止 2"(w1246) -> ()
            n646 = local write "停止 6"(w1246) -> ()
            n647 = local write "停止 7"(w1246) -> ()
            n648 = property class="VI"(reference=w1238, error in=w1239, "Front Panel.Open"=FALSE ("前面板窗口:打开")) -> ()  [unwired: 2 out]
          }
        }
        n649 = event-data("Discard?"=FALSE ("放弃？")) -> ()  [unwired: 1 in, 1 out]
      }
      event "刷新": Value Change {
        n650 = event-data() -> ("NewVal"=w1248:bool)  [unwired: 6 out]
        n651 = case shown="真" w1248 {
          frame False {
          }
          frame True {
            w1254 = cluster{u32, u32}[] [{0, 0}] ("颜色[4]")
            w1253 = "" ("布尔文本.文本")
            n652 = property on="Set结果" class="Bool (严格)"("Colors [4]"=w1254, "BoolText.Text"=w1253) -> ()  [unwired: 2 in, 2 out]
            n653 = property on="Read1结果" class="Bool (严格)"("Colors [4]"=w1254, "BoolText.Text"=w1253) -> ()  [unwired: 2 in, 2 out]
            n654 = property on="Clear_in结果" class="Bool (严格)"("Colors [4]"=w1254, "BoolText.Text"=w1253) -> ()  [unwired: 2 in, 2 out]
            n655 = property on="Current Offset结果 2" class="Bool (严格)"("Colors [4]"=w1254, "BoolText.Text"=w1253) -> ()  [unwired: 2 in, 2 out]
            n656 = property on="Current Offset结果 4" class="Bool (严格)"("Colors [4]"=w1254, "BoolText.Text"=w1253) -> ()  [unwired: 2 in, 2 out]
            n657 = property on="Current Gain结果 4" class="Bool (严格)"("Colors [4]"=w1254, "BoolText.Text"=w1253) -> ()  [unwired: 2 in, 2 out]
            n658 = property on="Set_out结果" class="Bool (严格)"("Colors [4]"=w1254, "BoolText.Text"=w1253) -> ()  [unwired: 2 in, 2 out]
            n659 = property on="Read2_Out结果" class="Bool (严格)"("Colors [4]"=w1254, "BoolText.Text"=w1253) -> ()  [unwired: 2 in, 2 out]
            n660 = property on="Read1_Out结果" class="Bool (严格)"("Colors [4]"=w1254, "BoolText.Text"=w1253) -> ()  [unwired: 2 in, 2 out]
            n661 = property on="Current Offset结果" class="Bool (严格)"("Colors [4]"=w1254, "BoolText.Text"=w1253) -> ()  [unwired: 2 in, 2 out]
            n662 = property on="Current Offset结果 3" class="Bool (严格)"("Colors [4]"=w1254, "BoolText.Text"=w1253) -> ()  [unwired: 2 in, 2 out]
            n663 = property on="Current Gain结果 3" class="Bool (严格)"("Colors [4]"=w1254, "BoolText.Text"=w1253) -> ()  [unwired: 2 in, 2 out]
            n664 = property on="Read2结果" class="Bool (严格)"("Colors [4]"=w1254, "BoolText.Text"=w1253) -> ()  [unwired: 2 in, 2 out]
            n665 = property on="Current Offset结果" class="Bool (严格)"("Colors [4]"=w1254, "BoolText.Text"=w1253) -> ()  [unwired: 2 in, 2 out]
            n666 = property on="Current Gain结果" class="Bool (严格)"("Colors [4]"=w1254, "BoolText.Text"=w1253) -> ()  [unwired: 2 in, 2 out]
            n667 = property on="Clear结果" class="Bool (严格)"("Colors [4]"=w1254, "BoolText.Text"=w1253) -> ()  [unwired: 2 in, 2 out]
            n668 = property on="Read1_in结果" class="Bool (严格)"("Colors [4]"=w1254, "BoolText.Text"=w1253) -> ()  [unwired: 2 in, 2 out]
            n669 = property on="Clear_out结果" class="Bool (严格)"("Colors [4]"=w1254, "BoolText.Text"=w1253) -> ()  [unwired: 2 in, 2 out]
            n670 = property on="Read2_in结果" class="Bool (严格)"("Colors [4]"=w1254, "BoolText.Text"=w1253) -> ()  [unwired: 2 in, 2 out]
            n671 = property on="Set_in结果" class="Bool (严格)"("Colors [4]"=w1254, "BoolText.Text"=w1253) -> ()  [unwired: 2 in, 2 out]
            n672 = property on="Current Gain结果 2" class="Bool (严格)"("Colors [4]"=w1254, "BoolText.Text"=w1253) -> ()  [unwired: 2 in, 2 out]
            n673 = control-ref of="结果"() -> (w1251:refnum<vi>)
            n674 = for {
              N: 40 -> [_]
              tunnel: w1251 -> [w1259]
              i -> [w1257]
              n675 = Bundle(w1257, 0) -> (w1255:cluster{i32, i32})  [unwired: 1 out]
              n676 = property class="MCListbox (严格)"(reference=w1259, "ActiveCell"=w1255, "CellBG"=u32 16448250) -> ()  [unwired: 1 in, 2 out]
            }
            n677 = property class="MCListbox (严格)"(reference=w1251, "ItemNames"=string[][] [] ("项名")) -> ()  [unwired: 1 in, 2 out]
            n678 = local write "分流器大小"(T2."选择分流器型号" ("Shunt Type")) -> ()
          }
        }
      }
      event "一键校正": Value Change {
        n679 = event-data() -> ("NewVal"=w1264:bool)  [unwired: 6 out]
        n680 = case shown="真" w1264 {
          tunnel: w1263 -> [w1266 w1270]
          tunnel: [w1266 w1269] -> w1262
          tunnel: w1261 -> [w1265 w1268]
          tunnel: [w1265 w1267] -> w1260
          frame False {
          }
          frame True {
            n681 = while {
              tunnel: w1270 -> [w1279]
              tunnel: [w1276] -> w1269
              tunnel: w1268 -> [w1278]
              tunnel: [w1277] -> w1267
              i -> [w1280]
              stop <- w1275 continue-if-true
              n682 = case shown="0, 默认" w1280 {
                tunnel: w1279 -> [w1293 w1320 w1356 w1428 w1464 w1537 w1577 w1617 w1659 w1730 w1772 w1835 w1925 w1964 w1988 w2073 w2119 w2162 w2247 w2293 w2337 w2382 w2440 w2587 w2619]
                tunnel: [w1285 w1313 w1354 w1421 w1462 w1530 w1570 w1612 w1656 w1725 w1765 w1833 TRUE ("status") w1961 w1984 w2068 w2114 w2159 w2242 w2288 w2332 w2377 w2437 w2583 w2616] -> w1275
                tunnel: w1278 -> [w1290 w1321 w1353 w1429 w1461 w1538 w1578 w1618 w1658 w1731 w1773 w1832 w1924 w1960 w1987 w2074 w2120 w2161 w2248 w2294 w2338 w2383 w2439 w2585 w2620]
                tunnel: [w1290 w1319 w1353 w1427 w1461 w1536 w1576 w1620 w1658 w1733 w1771 w1832 w1924 w1960 w1987 w2072 w2118 w2161 w2246 w2292 w2336 w2381 w2439 w2585 w2618] -> w1277
                tunnel: [w1292 w1318 w1355 w1426 w1463 w1535 w1575 w1619 w1657 w1732 w1770 w1834 w1923 w1963 w1986 w2071 w2117 w2160 w2245 w2291 w2335 w2380 w2438 w2586 w2617] -> w1276
                frame 0, Default {
                  # "打开电流源"
                  n683 = local read "VISA resource name 2"() -> (w1300:refnum<visa-resource-name>)
                  n684 = VISA Open(error in (no error)=w1293, VISA resource name=w1300) -> (VISA resource name=w1295:refnum<visa-resource-name>, error out=w1298:errorcluster)  [unwired: 3 out]
                  n685 = property class="Instr"(reference=w1295, "Timeout"=u32 100 ("General Settings:Timeout Value")) -> (reference out=w1294:refnum<visa-resource-name>)  [unwired: 1 in, 1 out]
                  n686 = VISA Write(VISA resource name=w1294, write buffer="*rst" ("写入缓冲区"), error in (no error)=w1298) -> (VISA resource name out=w1297:refnum<visa-resource-name>, error out=w1292:errorcluster)  [unwired: 1 out]
                  n687 = Unbundle(w1292) -> ("status"=w1291:bool)  [unwired: 2 out]
                  n688 = case shown="假" w1291 {
                    tunnel: w1297 -> [w1306 w1311]
                    tunnel: ["电流源连接成功" "电流源连接NG"] -> w1287
                    tunnel: [u32 6618880 u32 16711680] -> w1288
                    frame False {
                      w1304 = u8 0 ("禁用")
                      n689 = local write "VISA资源名称输出"(w1306) -> ()
                      n690 = local write "连接状态 10"(TRUE ("连接状态")) -> ()
                      n691 = property on="连接状态 10" class="Bool (严格)"("Colors [4]"=cluster{u32, u32}[] [{6618880, 6618880}] ("颜色[4]")) -> ()  [unwired: 2 in, 2 out]
                      n692 = property on="输出100A" class="Bool"("Disabled"=w1304) -> ()  [unwired: 2 in, 2 out]
                      n693 = property on="输出200A" class="Bool"("Disabled"=w1304) -> ()  [unwired: 2 in, 2 out]
                      n694 = property on="输出自定义值2 2" class="Bool"("Disabled"=w1304) -> ()  [unwired: 2 in, 2 out]
                      n695 = property on="输出自定义值1 2" class="Bool"("Disabled"=w1304) -> ()  [unwired: 2 in, 2 out]
                    }
                    frame True {
                      w1310 = u8 2 ("禁用")
                      n696 = local write "VISA资源名称输出"(w1311) -> ()
                      n697 = local write "连接状态 10"(FALSE ("连接状态")) -> ()
                      n698 = property on="连接状态 10" class="Bool (严格)"("Colors [4]"=cluster{u32, u32}[] [{15663131, 6618880}] ("颜色[4]")) -> ()  [unwired: 2 in, 2 out]
                      n699 = property on="输出100A" class="Bool"("Disabled"=w1310) -> ()  [unwired: 2 in, 2 out]
                      n700 = property on="输出200A" class="Bool"("Disabled"=w1310) -> ()  [unwired: 2 in, 2 out]
                      n701 = property on="输出自定义值2 2" class="Bool"("Disabled"=w1310) -> ()  [unwired: 2 in, 2 out]
                      n702 = property on="输出自定义值1 2" class="Bool"("Disabled"=w1310) -> ()  [unwired: 2 in, 2 out]
                    }
                  }
                  n703 = control-ref of="结果"() -> (w1289:refnum<vi>)
                  n704 = Build Array(w1287) -> (w1286:string[])
                  n705 = call "表格编辑.vi"("新元素/子数组"=w1286, "活动单元格:单元格背景色"=w1288, "MCListbox引用句柄"=w1289) -> ()  [unwired: 9 out]
                  n706 = Not(x=w1291) -> (.not. x?=w1285:bool)
                }
                frame 1 {
                  # "5460电流零点"
                  n707 = flat-sequence {
                    tunnel: w1320 -> [w1327]
                    tunnel: w1321 -> [w1328]
                    tunnel: [w1328] -> w1317
                    tunnel: [w1327] -> w1316
                    tunnel: w1317 -> [w1332]
                    tunnel: w1316 -> [w1331]
                    tunnel: [w1330] -> w1315
                    tunnel: [w1329] -> w1314
                    tunnel: [w1339] -> w1318
                    tunnel: [w1340] -> w1319
                    tunnel: w1315 -> [w1340]
                    tunnel: w1314 -> [w1339]
                    tunnel: [w1334] -> w1313
                    frame #0 {
                      n708 = local write "电流零点"("" ("5460Current Offset")) -> ()
                      n709 = global write "EV05全局变量1.vi" "高压校正接收"(FALSE ("高压校正接收")) -> ()
                      n710 = global write "EV05全局变量1.vi" "CAN接收"(FALSE ("CAN接收")) -> ()
                      n711 = call <vilib>:"Set Busy.vi"() -> ()  [unwired: 4 in, 8 out]
                      n712 = property on="Current Offset结果" class="Bool (严格)"("Colors [4]"=cluster{u32, u32}[] [{0, 0}] ("颜色[4]"), "BoolText.Text"="" ("布尔文本.文本")) -> ()  [unwired: 2 in, 2 out]
                    }
                    frame #1 {
                      n713 = Enqueue Element(queue=w1332, element="Set Current Offset" ("元素"), error in (no error)=w1331) -> (queue out=w1330:refnum<queue>, error out=w1329:errorcluster)  [unwired: 2 out]
                    }
                    frame #2 {
                      n714 = while {
                        tunnel: [w1346] -> w1334
                        i -> [w1351]
                        stop <- w1347 stop-if-true
                        n715 = property on="Current Offset结果" class="Bool (严格)"() -> ("BoolText.Text"=w1345:string)  [unwired: 2 in, 2 out]
                        n716 = Greater Or Equal?(x=w1351, y=30) -> (x >= y?=w1348:bool)
                        n717 = Not Equal?(x=w1345, y="NG" ("布尔文本.文本")) -> (x != y?=w1346:bool)
                        n718 = Wait Until Next ms Multiple(millisecond multiple=u32 110 ("毫秒倍数")) -> ()  [unwired: 1 out]
                        n719 = Or(x=w1346, y=w1348) -> (x .or. y?=w1347:bool)
                      }
                      n720 = case shown="真" w1334 {
                        tunnel: ["5460电流零点校正NG" "5460电流零点校正成功"] -> w1335
                        tunnel: [u32 16711680 u32 6618880] -> w1336
                        frame False {
                        }
                        frame True {
                        }
                      }
                      n721 = control-ref of="结果"() -> (w1337:refnum<vi>)
                      n722 = Build Array(w1335) -> (w1338:string[])
                      n723 = call "表格编辑.vi"("新元素/子数组"=w1338, "活动单元格:单元格背景色"=w1336, "MCListbox引用句柄"=w1337) -> ()  [unwired: 9 out]
                    }
                  }
                }
                frame 2 {
                  # "300A"
                  n724 = flat-sequence {
                    tunnel: FALSE ("控制读取") -> [w1369]
                    tunnel: [w1379] -> w1368
                    tunnel: [w1378] -> w1367
                    tunnel: [w1373] -> w1366
                    tunnel: w1356 -> [w1372]
                    tunnel: w1368 -> [w1383]
                    tunnel: [w1383] -> w1365
                    tunnel: w1367 -> [w1382]
                    tunnel: [w1382] -> w1364
                    tunnel: [w1380] -> w1363
                    tunnel: w1366 -> [w1380]
                    tunnel: w1365 -> [w1388]
                    tunnel: w1364 -> [w1387]
                    tunnel: [w1386] -> w1362
                    tunnel: [w1385] -> w1361
                    tunnel: w1363 -> [w1384]
                    tunnel: w1362 -> [w1391]
                    tunnel: [w1391] -> w1360
                    tunnel: w1361 -> [w1390]
                    tunnel: [w1390] -> w1359
                    tunnel: w1360 -> [w1395]
                    tunnel: w1359 -> [w1394]
                    tunnel: [w1392] -> w1358
                    tunnel: w1358 -> [w1403]
                    tunnel: [w1403] -> w1355
                    tunnel: [w1402] -> w1354
                    frame #0 {
                      n725 = local write "控制读取  2"(w1369) -> ()
                    }
                    frame #1 {
                      n726 = Wait (ms)(milliseconds to wait=u32 50 ("等待时间（毫秒）")) -> ()  [unwired: 1 out]
                    }
                    frame #2 {
                      n727 = local read "VISA资源名称输出"() -> (w1377:refnum<visa-resource-name>)
                      n728 = Number To Fractional String(number=300.0 ("数字"), precision (6)=i16 3 ("精度(6)")) -> (F-format string=w1374:string)  [unwired: 2 out]
                      n729 = Concatenate Strings("volt 1;curr " ("写入缓冲区"), w1374) -> (w1373:string)
                      n730 = VISA Write(VISA resource name=w1377, write buffer=w1373, error in (no error)=w1372) -> (VISA resource name out=w1379:refnum<visa-resource-name>, error out=w1378:errorcluster)  [unwired: 1 out]
                    }
                    frame #3 {
                      n731 = Wait (ms)(milliseconds to wait=u32 50 ("等待时间（毫秒）")) -> ()  [unwired: 1 out]
                    }
                    frame #4 {
                      n732 = VISA Write(VISA resource name=w1388, write buffer=w1384, error in (no error)=w1387) -> (VISA resource name out=w1386:refnum<visa-resource-name>, error out=w1385:errorcluster)  [unwired: 1 out]
                    }
                    frame #5 {
                      n733 = Wait (ms)(milliseconds to wait=u32 200 ("等待时间（毫秒）")) -> ()  [unwired: 1 out]
                    }
                    frame #6 {
                      n734 = Wait (ms)(milliseconds to wait=u32 50 ("等待时间（毫秒）")) -> ()  [unwired: 1 out]
                      n735 = VISA Write(VISA resource name=w1395, write buffer="outp on" ("写入缓冲区"), error in (no error)=w1394) -> (VISA resource name out=w1397:refnum<visa-resource-name>, error out=w1392:errorcluster)  [unwired: 1 out]
                      n736 = local write "VISA资源名称输出"(w1397) -> ()
                    }
                    frame #7 {
                      n737 = while {
                        tunnel: [w1406] -> w1402
                        i -> [w1409]
                        stop <- w1405 stop-if-true
                        w1411 = 300.0 ("x")
                        n738 = local read "Actual"() -> (w1415:dbl)
                        n739 = Greater Or Equal?(x=w1409, y=20) -> (x >= y?=w1407:bool)
                        n740 = Multiply(x=w1411, y=0.02) -> (x*y=w1412:dbl)
                        n741 = Add(x=w1411, y=w1412) -> (x+y=w1414:dbl)
                        n742 = Subtract(x=w1411, y=w1412) -> (x-y=w1413:dbl)
                        n743 = Wait Until Next ms Multiple(millisecond multiple=u32 200 ("毫秒倍数")) -> ()  [unwired: 1 out]
                        n744 = In Range and Coerce(upper limit=w1414, x=w1415, lower limit=w1413) -> (In Range?=w1406:bool)  [unwired: 1 out]
                        n745 = Or(x=w1406, y=w1407) -> (x .or. y?=w1405:bool)
                      }
                      n746 = local write "控制读取  2"(TRUE ("控制读取")) -> ()
                      n747 = case shown="假" w1402 {
                        tunnel: ["300A电流开启NG" "300A电流开启成功"] -> w1398
                        tunnel: [u32 16711680 u32 6618880] -> w1399
                        frame False {
                        }
                        frame True {
                        }
                      }
                      n748 = control-ref of="结果"() -> (w1400:refnum<vi>)
                      n749 = Build Array(w1398) -> (w1401:string[])
                      n750 = call "表格编辑.vi"("新元素/子数组"=w1401, "活动单元格:单元格背景色"=w1399, "MCListbox引用句柄"=w1400) -> ()  [unwired: 9 out]
                    }
                  }
                }
                frame 3 {
                  # "5460电流增益"
                  n751 = flat-sequence {
                    tunnel: w1428 -> [w1435]
                    tunnel: w1429 -> [w1436]
                    tunnel: [w1436] -> w1425
                    tunnel: [w1435] -> w1424
                    tunnel: w1425 -> [w1440]
                    tunnel: w1424 -> [w1439]
                    tunnel: [w1438] -> w1423
                    tunnel: [w1437] -> w1422
                    tunnel: [w1447] -> w1426
                    tunnel: [w1448] -> w1427
                    tunnel: w1423 -> [w1448]
                    tunnel: w1422 -> [w1447]
                    tunnel: [w1442] -> w1421
                    frame #0 {
                      n752 = global write "EV05全局变量1.vi" "高压校正接收"(FALSE ("高压校正接收")) -> ()
                      n753 = local write "电流增益"("" ("5460Current Offset")) -> ()
                      n754 = global write "EV05全局变量1.vi" "CAN接收"(FALSE ("CAN接收")) -> ()
                      n755 = call <vilib>:"Set Busy.vi"() -> ()  [unwired: 4 in, 8 out]
                      n756 = property on="Current Gain结果" class="Bool (严格)"("Colors [4]"=cluster{u32, u32}[] [{0, 0}] ("颜色[4]"), "BoolText.Text"="" ("布尔文本.文本")) -> ()  [unwired: 2 in, 2 out]
                    }
                    frame #1 {
                      n757 = Enqueue Element(queue=w1440, element="Set Current Gain" ("元素"), error in (no error)=w1439) -> (queue out=w1438:refnum<queue>, error out=w1437:errorcluster)  [unwired: 2 out]
                    }
                    frame #2 {
                      n758 = while {
                        tunnel: [w1454] -> w1442
                        i -> [w1459]
                        stop <- w1455 stop-if-true
                        n759 = property on="Current Gain结果" class="Bool (严格)"() -> ("BoolText.Text"=w1453:string)  [unwired: 2 in, 2 out]
                        n760 = Greater Or Equal?(x=w1459, y=30) -> (x >= y?=w1456:bool)
                        n761 = Not Equal?(x=w1453, y="NG" ("布尔文本.文本")) -> (x != y?=w1454:bool)
                        n762 = Wait Until Next ms Multiple(millisecond multiple=u32 110 ("毫秒倍数")) -> ()  [unwired: 1 out]
                        n763 = Or(x=w1454, y=w1456) -> (x .or. y?=w1455:bool)
                      }
                      n764 = case shown="假" w1442 {
                        tunnel: ["5460电流增益校正NG" "5460电流增益校正成功"] -> w1443
                        tunnel: [u32 16711680 u32 6618880] -> w1444
                        frame False {
                        }
                        frame True {
                        }
                      }
                      n765 = control-ref of="结果"() -> (w1445:refnum<vi>)
                      n766 = Build Array(w1443) -> (w1446:string[])
                      n767 = call "表格编辑.vi"("新元素/子数组"=w1446, "活动单元格:单元格背景色"=w1444, "MCListbox引用句柄"=w1445) -> ()  [unwired: 9 out]
                    }
                  }
                }
                frame 4 {
                  # "40A"
                  n768 = flat-sequence {
                    tunnel: FALSE ("控制读取") -> [w1478]
                    tunnel: [w1488] -> w1477
                    tunnel: [w1487] -> w1476
                    tunnel: [w1481] -> w1475
                    tunnel: w1464 -> [w1480]
                    tunnel: w1477 -> [w1492]
                    tunnel: [w1492] -> w1474
                    tunnel: w1476 -> [w1491]
                    tunnel: [w1491] -> w1473
                    tunnel: [w1489] -> w1472
                    tunnel: w1475 -> [w1489]
                    tunnel: w1474 -> [w1497]
                    tunnel: w1473 -> [w1496]
                    tunnel: [w1495] -> w1471
                    tunnel: [w1494] -> w1470
                    tunnel: w1472 -> [w1493]
                    tunnel: w1471 -> [w1500]
                    tunnel: [w1500] -> w1469
                    tunnel: w1470 -> [w1499]
                    tunnel: [w1499] -> w1468
                    tunnel: w1469 -> [w1504]
                    tunnel: w1468 -> [w1503]
                    tunnel: [w1501] -> w1467
                    tunnel: w1467 -> [w1512]
                    tunnel: [w1512] -> w1463
                    tunnel: [w1511] -> w1462
                    frame #0 {
                      n769 = local write "控制读取  2"(w1478) -> ()
                    }
                    frame #1 {
                      n770 = Wait (ms)(milliseconds to wait=u32 50 ("等待时间（毫秒）")) -> ()  [unwired: 1 out]
                    }
                    frame #2 {
                      n771 = local read "VISA资源名称输出"() -> (w1486:refnum<visa-resource-name>)
                      n772 = local read "Curr1"() -> (w1484:dbl)
                      n773 = Number To Fractional String(number=w1484, precision (6)=i16 3 ("精度(6)")) -> (F-format string=w1482:string)  [unwired: 2 out]
                      n774 = Concatenate Strings("volt 1;curr " ("写入缓冲区"), w1482) -> (w1481:string)
                      n775 = VISA Write(VISA resource name=w1486, write buffer=w1481, error in (no error)=w1480) -> (VISA resource name out=w1488:refnum<visa-resource-name>, error out=w1487:errorcluster)  [unwired: 1 out]
                    }
                    frame #3 {
                      n776 = Wait (ms)(milliseconds to wait=u32 50 ("等待时间（毫秒）")) -> ()  [unwired: 1 out]
                    }
                    frame #4 {
                      n777 = VISA Write(VISA resource name=w1497, write buffer=w1493, error in (no error)=w1496) -> (VISA resource name out=w1495:refnum<visa-resource-name>, error out=w1494:errorcluster)  [unwired: 1 out]
                    }
                    frame #5 {
                      n778 = Wait (ms)(milliseconds to wait=u32 200 ("等待时间（毫秒）")) -> ()  [unwired: 1 out]
                    }
                    frame #6 {
                      n779 = Wait (ms)(milliseconds to wait=u32 50 ("等待时间（毫秒）")) -> ()  [unwired: 1 out]
                      n780 = VISA Write(VISA resource name=w1504, write buffer="outp on" ("写入缓冲区"), error in (no error)=w1503) -> (VISA resource name out=w1506:refnum<visa-resource-name>, error out=w1501:errorcluster)  [unwired: 1 out]
                      n781 = local write "VISA资源名称输出"(w1506) -> ()
                    }
                    frame #7 {
                      n782 = while {
                        tunnel: [w1516] -> w1511
                        i -> [w1517]
                        stop <- w1515 stop-if-true
                        n783 = local read "Actual"() -> (w1524:dbl)
                        n784 = local read "Curr1"() -> (w1521:dbl)
                        n785 = Greater Or Equal?(x=w1517, y=20) -> (x >= y?=w1518:bool)
                        n786 = Multiply(x=w1521, y=0.02) -> (x*y=w1520:dbl)
                        n787 = Add(x=w1521, y=w1520) -> (x+y=w1523:dbl)
                        n788 = Subtract(x=w1521, y=w1520) -> (x-y=w1522:dbl)
                        n789 = Wait Until Next ms Multiple(millisecond multiple=u32 200 ("毫秒倍数")) -> ()  [unwired: 1 out]
                        n790 = In Range and Coerce(upper limit=w1523, x=w1524, lower limit=w1522) -> (In Range?=w1516:bool)  [unwired: 1 out]
                        n791 = Or(x=w1516, y=w1518) -> (x .or. y?=w1515:bool)
                      }
                      n792 = local write "控制读取  2"(TRUE ("控制读取")) -> ()
                      n793 = case shown="真" w1511 {
                        tunnel: ["40A电流开启NG" "40A电流开启成功"] -> w1507
                        tunnel: [u32 16711680 u32 6618880] -> w1508
                        frame False {
                        }
                        frame True {
                        }
                      }
                      n794 = control-ref of="结果"() -> (w1509:refnum<vi>)
                      n795 = Build Array(w1507) -> (w1510:string[])
                      n796 = call "表格编辑.vi"("新元素/子数组"=w1510, "活动单元格:单元格背景色"=w1508, "MCListbox引用句柄"=w1509) -> ()  [unwired: 9 out]
                    }
                  }
                  n797 = local read "Curr1"() -> (w1465:dbl)
                  n798 = local write "REAL1"(w1465) -> ()
                  n799 = local write "Set"(w1465) -> ()
                }
                frame 5 {
                  # "5460电压零点"
                  n800 = flat-sequence {
                    tunnel: w1537 -> [w1544]
                    tunnel: w1538 -> [w1545]
                    tunnel: [w1545] -> w1534
                    tunnel: [w1544] -> w1533
                    tunnel: w1534 -> [w1549]
                    tunnel: w1533 -> [w1548]
                    tunnel: [w1547] -> w1532
                    tunnel: [w1546] -> w1531
                    tunnel: [w1556] -> w1535
                    tunnel: [w1557] -> w1536
                    tunnel: w1532 -> [w1557]
                    tunnel: w1531 -> [w1556]
                    tunnel: [w1551] -> w1530
                    frame #0 {
                      n801 = local write "Shunt Volt Offset"("" ("5460Current Offset")) -> ()
                      n802 = global write "EV05全局变量1.vi" "高压校正接收"(FALSE ("高压校正接收")) -> ()
                      n803 = global write "EV05全局变量1.vi" "CAN接收"(FALSE ("CAN接收")) -> ()
                      n804 = call <vilib>:"Set Busy.vi"() -> ()  [unwired: 4 in, 8 out]
                      n805 = property on="Current Offset结果 2" class="Bool (严格)"("Colors [4]"=cluster{u32, u32}[] [{0, 0}] ("颜色[4]"), "BoolText.Text"="" ("布尔文本.文本")) -> ()  [unwired: 2 in, 2 out]
                    }
                    frame #1 {
                      n806 = Enqueue Element(queue=w1549, element="Set Volt offset" ("元素"), error in (no error)=w1548) -> (queue out=w1547:refnum<queue>, error out=w1546:errorcluster)  [unwired: 2 out]
                    }
                    frame #2 {
                      n807 = while {
                        tunnel: [w1563] -> w1551
                        i -> [w1568]
                        stop <- w1564 stop-if-true
                        n808 = property on="Current Offset结果 2" class="Bool (严格)"() -> ("BoolText.Text"=w1562:string)  [unwired: 2 in, 2 out]
                        n809 = Greater Or Equal?(x=w1568, y=30) -> (x >= y?=w1565:bool)
                        n810 = Not Equal?(x=w1562, y="NG" ("布尔文本.文本")) -> (x != y?=w1563:bool)
                        n811 = Wait Until Next ms Multiple(millisecond multiple=u32 110 ("毫秒倍数")) -> ()  [unwired: 1 out]
                        n812 = Or(x=w1563, y=w1565) -> (x .or. y?=w1564:bool)
                      }
                      n813 = case shown="真" w1551 {
                        tunnel: ["5460电压零点校正NG" "5460电压零点校正成功"] -> w1552
                        tunnel: [u32 16711680 u32 6618880] -> w1553
                        frame False {
                        }
                        frame True {
                        }
                      }
                      n814 = control-ref of="结果"() -> (w1554:refnum<vi>)
                      n815 = Build Array(w1552) -> (w1555:string[])
                      n816 = call "表格编辑.vi"("新元素/子数组"=w1555, "活动单元格:单元格背景色"=w1553, "MCListbox引用句柄"=w1554) -> ()  [unwired: 9 out]
                    }
                  }
                }
                frame 6 {
                  # "5460电压增益"
                  n817 = flat-sequence {
                    tunnel: w1577 -> [w1584]
                    tunnel: w1578 -> [w1585]
                    tunnel: [w1585] -> w1574
                    tunnel: [w1584] -> w1573
                    tunnel: w1574 -> [w1589]
                    tunnel: w1573 -> [w1588]
                    tunnel: [w1587] -> w1572
                    tunnel: [w1586] -> w1571
                    tunnel: [w1596] -> w1575
                    tunnel: [w1597] -> w1576
                    tunnel: w1572 -> [w1597]
                    tunnel: w1571 -> [w1596]
                    tunnel: [w1591] -> w1570
                    frame #0 {
                      n818 = local write "Shunt Volt Gain"("" ("5460Current Offset")) -> ()
                      n819 = global write "EV05全局变量1.vi" "高压校正接收"(FALSE ("高压校正接收")) -> ()
                      n820 = global write "EV05全局变量1.vi" "CAN接收"(FALSE ("CAN接收")) -> ()
                      n821 = call <vilib>:"Set Busy.vi"() -> ()  [unwired: 4 in, 8 out]
                      n822 = property on="Current Gain结果 2" class="Bool (严格)"("Colors [4]"=cluster{u32, u32}[] [{0, 0}] ("颜色[4]"), "BoolText.Text"="" ("布尔文本.文本")) -> ()  [unwired: 2 in, 2 out]
                    }
                    frame #1 {
                      n823 = Enqueue Element(queue=w1589, element="Set Volt Gain" ("元素"), error in (no error)=w1588) -> (queue out=w1587:refnum<queue>, error out=w1586:errorcluster)  [unwired: 2 out]
                    }
                    frame #2 {
                      n824 = while {
                        tunnel: [w1603] -> w1591
                        i -> [w1608]
                        stop <- w1604 stop-if-true
                        n825 = property on="Current Gain结果 2" class="Bool (严格)"() -> ("BoolText.Text"=w1602:string)  [unwired: 2 in, 2 out]
                        n826 = Greater Or Equal?(x=w1608, y=30) -> (x >= y?=w1605:bool)
                        n827 = Not Equal?(x=w1602, y="NG" ("布尔文本.文本")) -> (x != y?=w1603:bool)
                        n828 = Wait Until Next ms Multiple(millisecond multiple=u32 110 ("毫秒倍数")) -> ()  [unwired: 1 out]
                        n829 = Or(x=w1603, y=w1605) -> (x .or. y?=w1604:bool)
                      }
                      n830 = case shown="假" w1591 {
                        tunnel: ["5460电压增益校正NG" "5460电压增益校正成功"] -> w1592
                        tunnel: [u32 16711680 u32 6618880] -> w1593
                        frame False {
                        }
                        frame True {
                        }
                      }
                      n831 = control-ref of="结果"() -> (w1594:refnum<vi>)
                      n832 = Build Array(w1592) -> (w1595:string[])
                      n833 = call "表格编辑.vi"("新元素/子数组"=w1595, "活动单元格:单元格背景色"=w1593, "MCListbox引用句柄"=w1594) -> ()  [unwired: 9 out]
                    }
                  }
                }
                frame 7 {
                  # "AD1"
                  n834 = flat-sequence {
                    tunnel: w1617 -> [w1623]
                    tunnel: w1618 -> [w1624]
                    tunnel: [w1624] -> w1611
                    tunnel: [w1623] -> w1610
                    tunnel: [w1631] -> w1616
                    tunnel: [w1630] -> w1615
                    tunnel: w1611 -> [w1631]
                    tunnel: w1610 -> [w1630]
                    tunnel: w1616 -> [w1634]
                    tunnel: w1615 -> [w1633]
                    tunnel: [w1636] -> w1614
                    tunnel: [w1635] -> w1613
                    tunnel: [w1642] -> w1619
                    tunnel: [w1643] -> w1620
                    tunnel: w1614 -> [w1643]
                    tunnel: w1613 -> [w1642]
                    tunnel: [w1641] -> w1612
                    frame #0 {
                      n835 = One Button Dialog(message="请重启主板电源" ("消息"), button name ("OK")="确定" ("T按钮名称（“确定”）")) -> ()  [unwired: 1 out]
                    }
                    frame #1 {
                      n836 = global write "EV05全局变量1.vi" "CAN接收"(FALSE ("CAN接收")) -> ()
                      n837 = global write "EV05全局变量1.vi" "高压校正接收"(FALSE ("高压校正接收")) -> ()
                      n838 = local write "AD1"(u16 0 ("AD1")) -> ()
                      n839 = property on="Read1结果" class="Bool (严格)"("Colors [4]"=cluster{u32, u32}[] [{0, 0}] ("颜色[4]"), "BoolText.Text"="" ("布尔文本.文本")) -> ()  [unwired: 2 in, 2 out]
                    }
                    frame #2 {
                      n840 = Enqueue Element(queue=w1634, element="Read1" ("元素"), error in (no error)=w1633) -> (queue out=w1636:refnum<queue>, error out=w1635:errorcluster)  [unwired: 2 out]
                    }
                    frame #3 {
                      n841 = while {
                        tunnel: [w1648] -> w1641
                        i -> [w1653]
                        stop <- w1649 stop-if-true
                        n842 = property on="Read1结果" class="Bool (严格)"() -> ("BoolText.Text"=w1655:string)  [unwired: 2 in, 2 out]
                        n843 = Greater Or Equal?(x=w1653, y=30) -> (x >= y?=w1650:bool)
                        n844 = Not Equal?(x=w1655, y="NG" ("布尔文本.文本")) -> (x != y?=w1648:bool)
                        n845 = Wait Until Next ms Multiple(millisecond multiple=u32 110 ("毫秒倍数")) -> ()  [unwired: 1 out]
                        n846 = Or(x=w1648, y=w1650) -> (x .or. y?=w1649:bool)
                      }
                      n847 = case shown="真" w1641 {
                        tunnel: ["40A AD1值读取NG" "40A AD1值读取成功"] -> w1637
                        tunnel: [u32 16711680 u32 6618880] -> w1638
                        frame False {
                        }
                        frame True {
                        }
                      }
                      n848 = control-ref of="结果"() -> (w1639:refnum<vi>)
                      n849 = Build Array(w1637) -> (w1640:string[])
                      n850 = call "表格编辑.vi"("新元素/子数组"=w1640, "活动单元格:单元格背景色"=w1638, "MCListbox引用句柄"=w1639) -> ()  [unwired: 9 out]
                    }
                  }
                }
                frame 8 {
                  # "80A"
                  n851 = local read "Curr2"() -> (w1660:dbl)
                  n852 = flat-sequence {
                    tunnel: FALSE ("控制读取") -> [w1673]
                    tunnel: [w1683] -> w1672
                    tunnel: [w1682] -> w1671
                    tunnel: [w1677] -> w1670
                    tunnel: w1659 -> [w1675]
                    tunnel: w1672 -> [w1687]
                    tunnel: [w1687] -> w1669
                    tunnel: w1671 -> [w1686]
                    tunnel: [w1686] -> w1668
                    tunnel: [w1684] -> w1667
                    tunnel: w1670 -> [w1684]
                    tunnel: w1669 -> [w1692]
                    tunnel: w1668 -> [w1691]
                    tunnel: [w1690] -> w1666
                    tunnel: [w1689] -> w1665
                    tunnel: w1667 -> [w1688]
                    tunnel: w1666 -> [w1695]
                    tunnel: [w1695] -> w1664
                    tunnel: w1665 -> [w1694]
                    tunnel: [w1694] -> w1663
                    tunnel: w1664 -> [w1699]
                    tunnel: w1663 -> [w1698]
                    tunnel: [w1696] -> w1662
                    tunnel: w1662 -> [w1707]
                    tunnel: [w1707] -> w1657
                    tunnel: [w1706] -> w1656
                    frame #0 {
                      n853 = local write "控制读取  2"(w1673) -> ()
                    }
                    frame #1 {
                      n854 = Wait (ms)(milliseconds to wait=u32 50 ("等待时间（毫秒）")) -> ()  [unwired: 1 out]
                    }
                    frame #2 {
                      n855 = local read "VISA资源名称输出"() -> (w1681:refnum<visa-resource-name>)
                      n856 = local read "Curr2"() -> (w1676:dbl)
                      n857 = Number To Fractional String(number=w1676, precision (6)=i16 3 ("精度(6)")) -> (F-format string=w1678:string)  [unwired: 2 out]
                      n858 = Concatenate Strings("volt 1;curr " ("写入缓冲区"), w1678) -> (w1677:string)
                      n859 = VISA Write(VISA resource name=w1681, write buffer=w1677, error in (no error)=w1675) -> (VISA resource name out=w1683:refnum<visa-resource-name>, error out=w1682:errorcluster)  [unwired: 1 out]
                    }
                    frame #3 {
                      n860 = Wait (ms)(milliseconds to wait=u32 50 ("等待时间（毫秒）")) -> ()  [unwired: 1 out]
                    }
                    frame #4 {
                      n861 = VISA Write(VISA resource name=w1692, write buffer=w1688, error in (no error)=w1691) -> (VISA resource name out=w1690:refnum<visa-resource-name>, error out=w1689:errorcluster)  [unwired: 1 out]
                    }
                    frame #5 {
                      n862 = Wait (ms)(milliseconds to wait=u32 200 ("等待时间（毫秒）")) -> ()  [unwired: 1 out]
                    }
                    frame #6 {
                      n863 = Wait (ms)(milliseconds to wait=u32 50 ("等待时间（毫秒）")) -> ()  [unwired: 1 out]
                      n864 = VISA Write(VISA resource name=w1699, write buffer="outp on" ("写入缓冲区"), error in (no error)=w1698) -> (VISA resource name out=w1701:refnum<visa-resource-name>, error out=w1696:errorcluster)  [unwired: 1 out]
                      n865 = local write "VISA资源名称输出"(w1701) -> ()
                    }
                    frame #7 {
                      n866 = while {
                        tunnel: [w1711] -> w1706
                        i -> [w1709]
                        stop <- w1710 stop-if-true
                        n867 = local read "Curr2"() -> (w1715:dbl)
                        n868 = local read "Actual"() -> (w1719:dbl)
                        n869 = Greater Or Equal?(x=w1709, y=20) -> (x >= y?=w1713:bool)
                        n870 = Multiply(x=w1715, y=0.02) -> (x*y=w1716:dbl)
                        n871 = Add(x=w1715, y=w1716) -> (x+y=w1718:dbl)
                        n872 = Subtract(x=w1715, y=w1716) -> (x-y=w1717:dbl)
                        n873 = Wait Until Next ms Multiple(millisecond multiple=u32 200 ("毫秒倍数")) -> ()  [unwired: 1 out]
                        n874 = In Range and Coerce(upper limit=w1718, x=w1719, lower limit=w1717) -> (In Range?=w1711:bool)  [unwired: 1 out]
                        n875 = Or(x=w1711, y=w1713) -> (x .or. y?=w1710:bool)
                      }
                      n876 = local write "控制读取  2"(TRUE ("控制读取")) -> ()
                      n877 = case shown="真" w1706 {
                        tunnel: ["80A电流开启NG" "80A电流开启成功"] -> w1702
                        tunnel: [u32 16711680 u32 6618880] -> w1703
                        frame False {
                        }
                        frame True {
                        }
                      }
                      n878 = control-ref of="结果"() -> (w1704:refnum<vi>)
                      n879 = Build Array(w1702) -> (w1705:string[])
                      n880 = call "表格编辑.vi"("新元素/子数组"=w1705, "活动单元格:单元格背景色"=w1703, "MCListbox引用句柄"=w1704) -> ()  [unwired: 9 out]
                    }
                  }
                  n881 = local write "REAL2"(w1660) -> ()
                  n882 = local write "Set"(w1660) -> ()
                }
                frame 9 {
                  # "AD2"
                  n883 = flat-sequence {
                    tunnel: w1730 -> [w1739]
                    tunnel: w1731 -> [w1740]
                    tunnel: [w1740] -> w1729
                    tunnel: [w1739] -> w1728
                    tunnel: w1729 -> [w1743]
                    tunnel: w1728 -> [w1742]
                    tunnel: [w1745] -> w1727
                    tunnel: [w1744] -> w1726
                    tunnel: [w1751] -> w1732
                    tunnel: [w1752] -> w1733
                    tunnel: w1727 -> [w1752]
                    tunnel: w1726 -> [w1751]
                    tunnel: [w1750] -> w1725
                    frame #0 {
                      n884 = local write "AD2"(u16 0 ("AD2")) -> ()
                      n885 = global write "EV05全局变量1.vi" "CAN接收"(FALSE ("CAN接收")) -> ()
                      n886 = global write "EV05全局变量1.vi" "高压校正接收"(FALSE ("高压校正接收")) -> ()
                      n887 = property on="Read2结果" class="Bool (严格)"("Colors [4]"=cluster{u32, u32}[] [{0, 0}] ("颜色[4]"), "BoolText.Text"="" ("布尔文本.文本")) -> ()  [unwired: 2 in, 2 out]
                    }
                    frame #1 {
                      n888 = Enqueue Element(queue=w1743, element="Read2" ("元素"), error in (no error)=w1742) -> (queue out=w1745:refnum<queue>, error out=w1744:errorcluster)  [unwired: 2 out]
                    }
                    frame #2 {
                      n889 = while {
                        tunnel: [w1758] -> w1750
                        i -> [w1763]
                        stop <- w1759 stop-if-true
                        n890 = property on="Read2结果" class="Bool (严格)"() -> ("BoolText.Text"=w1757:string)  [unwired: 2 in, 2 out]
                        n891 = Greater Or Equal?(x=w1763, y=30) -> (x >= y?=w1760:bool)
                        n892 = Not Equal?(x=w1757, y="NG" ("布尔文本.文本")) -> (x != y?=w1758:bool)
                        n893 = Wait Until Next ms Multiple(millisecond multiple=u32 110 ("毫秒倍数")) -> ()  [unwired: 1 out]
                        n894 = Or(x=w1758, y=w1760) -> (x .or. y?=w1759:bool)
                      }
                      n895 = case shown="假" w1750 {
                        tunnel: ["80A AD2值读取NG" "80A AD2值读取成功"] -> w1746
                        tunnel: [u32 16711680 u32 6618880] -> w1747
                        frame False {
                        }
                        frame True {
                        }
                      }
                      n896 = control-ref of="结果"() -> (w1748:refnum<vi>)
                      n897 = Build Array(w1746) -> (w1749:string[])
                      n898 = call "表格编辑.vi"("新元素/子数组"=w1749, "活动单元格:单元格背景色"=w1747, "MCListbox引用句柄"=w1748) -> ()  [unwired: 9 out]
                    }
                  }
                }
                frame 10 {
                  # "写入电流增益"
                  n899 = flat-sequence {
                    tunnel: w1772 -> [w1788]
                    tunnel: w1773 -> [w1789]
                    tunnel: [w1789] -> w1769
                    tunnel: [w1788] -> w1768
                    tunnel: w1769 -> [w1794]
                    tunnel: w1768 -> [w1793]
                    tunnel: [w1792] -> w1767
                    tunnel: [w1791] -> w1766
                    tunnel: [w1800] -> w1771
                    tunnel: [w1801] -> w1770
                    tunnel: w1767 -> [w1801]
                    tunnel: w1766 -> [w1800]
                    tunnel: [w1799] -> w1765
                    frame #0 {
                      n900 = local read "REAL2"() -> (w1786:dbl)
                      n901 = local read "REAL1"() -> (w1785:dbl)
                      n902 = local read "AD1"() -> (w1781:u16)
                      n903 = local read "AD2"() -> (w1782:u16)
                      n904 = Subtract(x=w1786, y=w1785) -> (x-y=w1784:dbl)
                      n905 = Subtract(x=w1782, y=w1781) -> (x-y=w1780:u16)
                      n906 = Multiply(x=w1784, y=1000000.0) -> (x*y=w1783:dbl)
                      n907 = global write "EV05全局变量1.vi" "CAN接收"(FALSE ("CAN接收")) -> ()
                      n908 = Divide(x=w1783, y=w1780) -> (x/y=w1779:dbl)
                      n909 = Round Toward -Infinity(1:w1779) -> (0:w1778:dbl)
                      n910 = local write "Gain"(w1778) -> ()
                      n911 = global write "EV05全局变量1.vi" "高压校正接收"(FALSE ("高压校正接收")) -> ()
                      n912 = property on="Set结果" class="Bool (严格)"("Colors [4]"=cluster{u32, u32}[] [{0, 0}] ("颜色[4]"), "BoolText.Text"="" ("布尔文本.文本")) -> ()  [unwired: 2 in, 2 out]
                    }
                    frame #1 {
                      n913 = Enqueue Element(queue=w1794, element="Set" ("元素"), error in (no error)=w1793) -> (queue out=w1791:refnum<queue>, error out=w1792:errorcluster)  [unwired: 2 out]
                    }
                    frame #2 {
                      n914 = while {
                        tunnel: [w1807] -> w1799
                        i -> [w1812]
                        stop <- w1808 stop-if-true
                        n915 = property on="Set结果" class="Bool (严格)"() -> ("BoolText.Text"=w1806:string)  [unwired: 2 in, 2 out]
                        n916 = Greater Or Equal?(x=w1812, y=30) -> (x >= y?=w1809:bool)
                        n917 = Not Equal?(x=w1806, y="NG" ("布尔文本.文本")) -> (x != y?=w1807:bool)
                        n918 = Wait Until Next ms Multiple(millisecond multiple=u32 110 ("毫秒倍数")) -> ()  [unwired: 1 out]
                        n919 = Or(x=w1807, y=w1809) -> (x .or. y?=w1808:bool)
                      }
                      n920 = case shown="假" w1799 {
                        tunnel: ["设电流增益NG" "设电流增益成功"] -> w1795
                        tunnel: [u32 16711680 u32 6618880] -> w1796
                        frame False {
                        }
                        frame True {
                        }
                      }
                      n921 = control-ref of="结果"() -> (w1797:refnum<vi>)
                      n922 = Build Array(w1795) -> (w1798:string[])
                      n923 = call "表格编辑.vi"("新元素/子数组"=w1798, "活动单元格:单元格背景色"=w1796, "MCListbox引用句柄"=w1797) -> ()  [unwired: 9 out]
                    }
                  }
                }
                frame 11 {
                  # "检验电流校正状态"
                  n924 = flat-sequence {
                    tunnel: [w1836] -> w1831
                    tunnel: [w1841] -> w1830
                    tunnel: w1831 -> [w1841]
                    tunnel: [w1852] -> w1829
                    tunnel: [w1851] -> w1828
                    tunnel: [w1846] -> w1827
                    tunnel: w1835 -> [w1845]
                    tunnel: [w1843] -> w1826
                    tunnel: w1830 -> [w1843]
                    tunnel: w1829 -> [w1857]
                    tunnel: [w1857] -> w1825
                    tunnel: w1828 -> [w1856]
                    tunnel: [w1856] -> w1824
                    tunnel: [w1854] -> w1823
                    tunnel: w1827 -> [w1854]
                    tunnel: [w1853] -> w1822
                    tunnel: w1826 -> [w1853]
                    tunnel: w1825 -> [w1863]
                    tunnel: w1824 -> [w1862]
                    tunnel: [w1861] -> w1821
                    tunnel: [w1860] -> w1820
                    tunnel: w1823 -> [w1859]
                    tunnel: [w1858] -> w1819
                    tunnel: w1822 -> [w1858]
                    tunnel: w1821 -> [w1867]
                    tunnel: [w1867] -> w1818
                    tunnel: w1820 -> [w1866]
                    tunnel: [w1866] -> w1817
                    tunnel: [w1864] -> w1816
                    tunnel: w1819 -> [w1864]
                    tunnel: w1818 -> [w1872]
                    tunnel: w1817 -> [w1871]
                    tunnel: [w1869] -> w1815
                    tunnel: [w1868] -> w1814
                    tunnel: w1816 -> [w1868]
                    tunnel: w1815 -> [w1877]
                    tunnel: [w1877] -> w1834
                    tunnel: [w1875] -> w1833
                    tunnel: w1814 -> [w1876]
                    frame #0 {
                      n925 = local read "Actual"() -> (w1838:dbl)
                      n926 = local read "电流"() -> (w1840:dbl)
                      n927 = Subtract(x=w1838, y=w1840) -> (x-y=w1839:dbl)
                      n928 = Absolute Value(x=w1839) -> (abs(x)=w1837:dbl)
                      n929 = Divide(x=w1837, y=w1838) -> (x/y=w1836:dbl)
                    }
                    frame #1 {
                      n930 = Wait (ms)(milliseconds to wait=u32 50 ("等待时间（毫秒）")) -> ()  [unwired: 1 out]
                    }
                    frame #2 {
                      n931 = local read "VISA资源名称输出"() -> (w1850:refnum<visa-resource-name>)
                      n932 = Number To Fractional String(number=200.0 ("数字"), precision (6)=i16 3 ("精度(6)")) -> (F-format string=w1847:string)  [unwired: 2 out]
                      n933 = Concatenate Strings("volt 1;curr " ("写入缓冲区"), w1847) -> (w1846:string)
                      n934 = VISA Write(VISA resource name=w1850, write buffer=w1846, error in (no error)=w1845) -> (VISA resource name out=w1852:refnum<visa-resource-name>, error out=w1851:errorcluster)  [unwired: 1 out]
                    }
                    frame #3 {
                      n935 = Wait (ms)(milliseconds to wait=u32 50 ("等待时间（毫秒）")) -> ()  [unwired: 1 out]
                    }
                    frame #4 {
                      n936 = VISA Write(VISA resource name=w1863, write buffer=w1859, error in (no error)=w1862) -> (VISA resource name out=w1861:refnum<visa-resource-name>, error out=w1860:errorcluster)  [unwired: 1 out]
                    }
                    frame #5 {
                      n937 = Wait (ms)(milliseconds to wait=u32 200 ("等待时间（毫秒）")) -> ()  [unwired: 1 out]
                    }
                    frame #6 {
                      n938 = Wait (ms)(milliseconds to wait=u32 50 ("等待时间（毫秒）")) -> ()  [unwired: 1 out]
                      n939 = VISA Write(VISA resource name=w1872, write buffer="outp on" ("写入缓冲区"), error in (no error)=w1871) -> (VISA resource name out=w1874:refnum<visa-resource-name>, error out=w1869:errorcluster)  [unwired: 1 out]
                      n940 = local write "VISA资源名称输出"(w1874) -> ()
                    }
                    frame #7 {
                      n941 = stacked-sequence {
                        seq-local: [w1878 _ _] -> [_ w1891 _]
                        tunnel: w1876 -> [_ _ w1912]
                        tunnel: [_ w1891 _] -> w1875
                        frame #0 {
                          n942 = while {
                            tunnel: [w1882] -> w1878
                            i -> [w1880]
                            stop <- w1881 stop-if-true
                            w1879 = 200.0 ("y")
                            n943 = local read "Actual"() -> (w1889:dbl)
                            n944 = Greater Or Equal?(x=w1880, y=20) -> (x >= y?=w1884:bool)
                            n945 = Multiply(x=w1879, y=0.02) -> (x*y=w1886:dbl)
                            n946 = Add(x=w1879, y=w1886) -> (x+y=w1888:dbl)
                            n947 = Subtract(x=w1879, y=w1886) -> (x-y=w1887:dbl)
                            n948 = Wait Until Next ms Multiple(millisecond multiple=u32 200 ("毫秒倍数")) -> ()  [unwired: 1 out]
                            n949 = In Range and Coerce(upper limit=w1888, x=w1889, lower limit=w1887) -> (In Range?=w1882:bool)  [unwired: 1 out]
                            n950 = Or(x=w1882, y=w1884) -> (x .or. y?=w1881:bool)
                          }
                        }
                        frame #1 {
                          n951 = case shown="假" w1891 {
                            tunnel: ["200A电流开启NG" "200A电流开启成功"] -> w1892
                            tunnel: [u32 16711680 u32 6618880] -> w1893
                            frame False {
                            }
                            frame True {
                            }
                          }
                          n952 = control-ref of="结果"() -> (w1894:refnum<vi>)
                          n953 = Build Array(w1892) -> (w1895:string[])
                          n954 = call "表格编辑.vi"("新元素/子数组"=w1895, "活动单元格:单元格背景色"=w1893, "MCListbox引用句柄"=w1894) -> ()  [unwired: 9 out]
                        }
                        frame #2 {
                          n955 = local read "Actual"() -> (w1917:dbl)
                          n956 = local read "电流"() -> (w1916:dbl)
                          n957 = Multiply(x=w1912, y=100.0) -> (x*y=w1913:dbl)
                          n958 = Subtract(x=w1917, y=w1916) -> (x-y=w1918:dbl)
                          n959 = Format Into String(format string="%.3f%" ("格式字符串"), w1913) -> (resulting string=w1910:string)  [unwired: 2 in, 1 out]
                          n960 = Absolute Value(x=w1918) -> (abs(x)=w1919:dbl)
                          n961 = Divide(x=w1919, y=w1917) -> (x/y=w1907:dbl)
                          n962 = Multiply(x=w1907, y=100.0) -> (x*y=w1908:dbl)
                          n963 = Format Into String(format string="%.3f%" ("格式字符串"), w1908) -> (resulting string=w1905:string)  [unwired: 2 in, 1 out]
                          n964 = Concatenate Strings("80A误差", w1910, "  200A误差", w1905) -> (w1900:string)
                          n965 = control-ref of="结果"() -> (w1902:refnum<vi>)
                          n966 = Build Array(w1900) -> (w1903:string[])
                          n967 = call "表格编辑.vi"("新元素/子数组"=w1903, "活动单元格:单元格背景色"=u32 6618880, "MCListbox引用句柄"=w1902) -> ()  [unwired: 9 out]
                        }
                      }
                    }
                  }
                }
                frame 12 {
                  # "关闭电流源"
                  n968 = local read "VISA资源名称输出"() -> (w1926:refnum<visa-resource-name>)
                  n969 = local write "控制读取  2"(FALSE ("控制读取")) -> ()
                  n970 = flat-sequence {
                    tunnel: [w1935] -> w1933
                    tunnel: w1926 -> [w1935]
                    tunnel: w1933 -> [w1939]
                    tunnel: [w1938] -> w1932
                    tunnel: w1925 -> [w1937]
                    tunnel: [w1936] -> w1931
                    tunnel: w1932 -> [w1943]
                    tunnel: [w1943] -> w1930
                    tunnel: [w1941] -> w1929
                    tunnel: w1931 -> [w1941]
                    tunnel: w1930 -> [w1948]
                    tunnel: w1929 -> [w1945]
                    tunnel: [w1947] -> w1921
                    tunnel: [w1944] -> w1920
                    tunnel: [w1954] -> w1923
                    tunnel: [w1955] -> w1927
                    tunnel: w1921 -> [w1955]
                    tunnel: w1920 -> [w1954]
                    frame #0 {
                      n971 = Wait (ms)(milliseconds to wait=u32 200 ("等待时间（毫秒）")) -> ()  [unwired: 1 out]
                    }
                    frame #1 {
                      n972 = VISA Write(VISA resource name=w1939, write buffer="outp off" ("写入缓冲区"), error in (no error)=w1937) -> (VISA resource name out=w1938:refnum<visa-resource-name>, error out=w1936:errorcluster)  [unwired: 1 out]
                    }
                    frame #2 {
                      n973 = Wait (ms)(milliseconds to wait=u32 50 ("等待时间（毫秒）")) -> ()  [unwired: 1 out]
                    }
                    frame #3 {
                      n974 = local write "控制读取  2"(TRUE ("控制读取")) -> ()
                      n975 = VISA Write(VISA resource name=w1948, write buffer="outp off" ("写入缓冲区"), error in (no error)=w1945) -> (VISA resource name out=w1947:refnum<visa-resource-name>, error out=w1944:errorcluster)  [unwired: 1 out]
                    }
                    frame #4 {
                      n976 = control-ref of="结果"() -> (w1952:refnum<vi>)
                      n977 = Build Array("电流源关闭") -> (w1953:string[])
                      n978 = call "表格编辑.vi"("新元素/子数组"=w1953, "活动单元格:单元格背景色"=u32 6618880, "MCListbox引用句柄"=w1952) -> ()  [unwired: 9 out]
                    }
                  }
                  n979 = local write "VISA资源名称输出"(w1927) -> ()
                }
                frame 13 {
                  # "打开电压源"
                  n980 = local read "VISA resource name 4"() -> (w1965:refnum<visa-resource-name>)
                  n981 = VISA Open(error in (no error)=w1964, VISA resource name=w1965) -> (VISA resource name=w1969:refnum<visa-resource-name>, error out=w1968:errorcluster)  [unwired: 1 in, 2 out]
                  n982 = property class="Instr"(reference=w1969, error in=w1968, "Timeout"=u32 100 ("General Settings:Timeout Value")) -> (reference out=w1966:refnum<visa-resource-name>, error out=w1967:errorcluster)
                  n983 = call-poly "VISA Configure Serial Port"("VISA resource name"=w1966, "error in (no error)"=w1967) -> ("VISA resource name out"=w1971:refnum<visa-resource-name>, "error out"=w1963:errorcluster)  [unwired: 4 in, 8 out]
                  n984 = Unbundle(w1963) -> ("status"=w1962:bool)  [unwired: 2 out]
                  n985 = case shown="真" w1962 {
                    tunnel: w1971 -> [w1977 w1982]
                    tunnel: ["电压源打开成功" "电压源打开成功"] -> w1957
                    tunnel: [u32 6618880 u32 16711680] -> w1956
                    frame False {
                      w1975 = u8 0 ("禁用")
                      n986 = local write "VISA资源名称输出 10"(w1977) -> ()
                      n987 = local write "连接状态 10"(TRUE ("连接状态")) -> ()
                      n988 = property on="输出150V" class="Bool"("Disabled"=w1975) -> ()  [unwired: 2 in, 2 out]
                      n989 = property on="输出300V" class="Bool"("Disabled"=w1975) -> ()  [unwired: 2 in, 2 out]
                      n990 = property on="输出自定义值2" class="Bool"("Disabled"=w1975) -> ()  [unwired: 2 in, 2 out]
                      n991 = property on="输出自定义值1" class="Bool"("Disabled"=w1975) -> ()  [unwired: 2 in, 2 out]
                      n992 = property on="连接状态 10" class="Bool (严格)"("Colors [4]"=cluster{u32, u32}[] [{6618880, 6618880}] ("颜色[4]")) -> ()  [unwired: 2 in, 2 out]
                    }
                    frame True {
                      w1981 = u8 2 ("禁用")
                      n993 = local write "VISA资源名称输出 10"(w1982) -> ()
                      n994 = local write "连接状态 10"(FALSE ("连接状态")) -> ()
                      n995 = property on="输出自定义值2" class="Bool"("Disabled"=w1981) -> ()  [unwired: 2 in, 2 out]
                      n996 = property on="输出150V" class="Bool"("Disabled"=w1981) -> ()  [unwired: 2 in, 2 out]
                      n997 = property on="输出自定义值1" class="Bool"("Disabled"=w1981) -> ()  [unwired: 2 in, 2 out]
                      n998 = property on="输出300V" class="Bool"("Disabled"=w1981) -> ()  [unwired: 2 in, 2 out]
                      n999 = property on="连接状态 10" class="Bool (严格)"("Colors [4]"=cluster{u32, u32}[] [{15663131, 6618880}] ("颜色[4]")) -> ()  [unwired: 2 in, 2 out]
                    }
                  }
                  n1000 = control-ref of="结果"() -> (w1959:refnum<vi>)
                  n1001 = Build Array(w1957) -> (w1958:string[])
                  n1002 = call "表格编辑.vi"("新元素/子数组"=w1958, "活动单元格:单元格背景色"=w1956, "MCListbox引用句柄"=w1959) -> ()  [unwired: 9 out]
                  n1003 = Not(x=w1962) -> (.not. x?=w1961:bool)
                }
                frame 14 {
                  w1997 = "," ("字符串")
                  # "150V"
                  n1004 = local read "Volt1"() -> (w1985:dbl)
                  n1005 = local write "REAL1"(w1985) -> ()
                  n1006 = local write "REAL1"(w1985) -> ()
                  n1007 = local write "Set"(w1985) -> ()
                  n1008 = local write "控制读取  5"(FALSE ("控制读取")) -> ()
                  n1009 = Number To Fractional String(number=w1985, precision (6)=i16 2 ("精度(6)")) -> (F-format string=w2001:string)  [unwired: 2 out]
                  n1010 = Number To Fractional String(number=0.2 ("数字"), precision (6)=i16 2 ("精度(6)")) -> (F-format string=w2000:string)  [unwired: 2 out]
                  n1011 = Number To Fractional String(number=1.0 ("数字"), precision (6)=i16 2 ("精度(6)")) -> (F-format string=w1998:string)  [unwired: 2 out]
                  n1012 = Number To Fractional String(number=320.0 ("数字"), precision (6)=i16 2 ("精度(6)")) -> (F-format string=w1999:string)  [unwired: 2 out]
                  n1013 = Concatenate Strings(w2001, w1997, w2000, w1997, w1999, w1997, w1998, w1997, w1997, w1997) -> (w1996:string)
                  n1014 = flat-sequence {
                    tunnel: [w2020] -> w2012
                    tunnel: [w2019] -> w2011
                    tunnel: [w2018] -> w2010
                    tunnel: w1996 -> [w2015]
                    tunnel: w1988 -> [w2014]
                    tunnel: w2012 -> [w2025]
                    tunnel: [w2025] -> w2009
                    tunnel: w2011 -> [w2024]
                    tunnel: [w2024] -> w2008
                    tunnel: w2010 -> [w2023]
                    tunnel: [w2023] -> w2007
                    tunnel: w2009 -> [w2029]
                    tunnel: w2008 -> [w2028]
                    tunnel: w2007 -> [_]
                    tunnel: [w2027] -> w2006
                    tunnel: [w2026] -> w2005
                    tunnel: w2006 -> [w2035]
                    tunnel: [w2035] -> w2004
                    tunnel: w2005 -> [w2034]
                    tunnel: [w2034] -> w2003
                    tunnel: w2004 -> [w2038]
                    tunnel: w2003 -> [w2037]
                    tunnel: [w2036] -> w1986
                    tunnel: [w2046] -> w1984
                    frame #0 {
                      n1015 = Wait (ms)(milliseconds to wait=u32 50 ("等待时间（毫秒）")) -> ()  [unwired: 1 out]
                    }
                    frame #1 {
                      n1016 = local read "VISA资源名称输出 10"() -> (w2017:refnum<visa-resource-name>)
                      n1017 = Concatenate Strings("SET:GRO 12," ("写入缓冲区"), w2015, "\n") -> (w2018:string)
                      n1018 = VISA Write(VISA resource name=w2017, write buffer=w2018, error in (no error)=w2014) -> (VISA resource name out=w2020:refnum<visa-resource-name>, error out=w2019:errorcluster)  [unwired: 1 out]
                    }
                    frame #2 {
                      n1019 = Wait (ms)(milliseconds to wait=u32 50 ("等待时间（毫秒）")) -> ()  [unwired: 1 out]
                    }
                    frame #3 {
                      n1020 = Concatenate Strings("SET:STE 12" ("写入缓冲区"), "\n") -> (w2030:string)
                      n1021 = VISA Write(VISA resource name=w2029, write buffer=w2030, error in (no error)=w2028) -> (VISA resource name out=w2027:refnum<visa-resource-name>, error out=w2026:errorcluster)  [unwired: 1 out]
                    }
                    frame #4 {
                      n1022 = Wait (ms)(milliseconds to wait=u32 200 ("等待时间（毫秒）")) -> ()  [unwired: 1 out]
                    }
                    frame #5 {
                      n1023 = Concatenate Strings("OUT:ON" ("写入缓冲区"), "\n") -> (w2043:string)
                      n1024 = Wait (ms)(milliseconds to wait=u32 50 ("等待时间（毫秒）")) -> ()  [unwired: 1 out]
                      n1025 = VISA Write(VISA resource name=w2038, write buffer=w2043, error in (no error)=w2037) -> (VISA resource name out=w2040:refnum<visa-resource-name>, error out=w2036:errorcluster)  [unwired: 1 out]
                      n1026 = local write "VISA资源名称输出 10"(w2040) -> ()
                    }
                    frame #6 {
                      n1027 = while {
                        tunnel: [w2051] -> w2046
                        i -> [w2052]
                        stop <- w2050 stop-if-true
                        n1028 = local read "Actual"() -> (w2057:dbl)
                        n1029 = local read "Volt1"() -> (w2056:dbl)
                        n1030 = Greater Or Equal?(x=w2052, y=20) -> (x >= y?=w2054:bool)
                        n1031 = Multiply(x=w2056, y=0.02) -> (x*y=w2058:dbl)
                        n1032 = Add(x=w2056, y=w2058) -> (x+y=w2060:dbl)
                        n1033 = Subtract(x=w2056, y=w2058) -> (x-y=w2059:dbl)
                        n1034 = Wait Until Next ms Multiple(millisecond multiple=u32 200 ("毫秒倍数")) -> ()  [unwired: 1 out]
                        n1035 = In Range and Coerce(upper limit=w2060, x=w2057, lower limit=w2059) -> (In Range?=w2051:bool)  [unwired: 1 out]
                        n1036 = Or(x=w2051, y=w2054) -> (x .or. y?=w2050:bool)
                      }
                      n1037 = case shown="假" w2046 {
                        tunnel: ["150V电压开启NG" "150V电压开启成功"] -> w2045
                        tunnel: [u32 16711680 u32 6618880] -> w2044
                        frame False {
                        }
                        frame True {
                        }
                      }
                      n1038 = control-ref of="结果"() -> (w2048:refnum<vi>)
                      n1039 = Build Array(w2045) -> (w2047:string[])
                      n1040 = local write "控制读取  5"(TRUE ("控制读取")) -> ()
                      n1041 = call "表格编辑.vi"("新元素/子数组"=w2047, "活动单元格:单元格背景色"=w2044, "MCListbox引用句柄"=w2048) -> ()  [unwired: 9 out]
                    }
                  }
                }
                frame 15 {
                  # "150V内总压AD1"
                  n1042 = flat-sequence {
                    tunnel: w2073 -> [w2079]
                    tunnel: w2074 -> [w2080]
                    tunnel: [w2080] -> w2067
                    tunnel: [w2079] -> w2066
                    tunnel: [w2087] -> w2076
                    tunnel: [w2086] -> w2075
                    tunnel: w2067 -> [w2087]
                    tunnel: w2066 -> [w2086]
                    tunnel: w2076 -> [w2092]
                    tunnel: w2075 -> [w2091]
                    tunnel: [w2090] -> w2070
                    tunnel: [w2089] -> w2069
                    tunnel: [w2098] -> w2072
                    tunnel: [w2099] -> w2071
                    tunnel: w2070 -> [w2099]
                    tunnel: w2069 -> [w2098]
                    tunnel: [w2097] -> w2068
                    frame #0 {
                      n1043 = One Button Dialog(message="请把继电器调到\n内总压状态" ("消息"), button name ("OK")="确定" ("按钮名称（“确定”）")) -> ()  [unwired: 1 out]
                    }
                    frame #1 {
                      n1044 = global write "EV05全局变量1.vi" "CAN接收"(FALSE ("CAN接收")) -> ()
                      n1045 = global write "EV05全局变量1.vi" "高压校正接收"(FALSE ("高压校正接收")) -> ()
                      n1046 = local write "AD1"(0.0 ("AD1 2")) -> ()
                      n1047 = property on="Read1_in结果" class="Bool (严格)"("Colors [4]"=cluster{u32, u32}[] [{0, 0}] ("颜色[4]"), "BoolText.Text"="" ("布尔文本.文本")) -> ()  [unwired: 2 in, 2 out]
                    }
                    frame #2 {
                      n1048 = Enqueue Element(queue=w2092, element="Read1_in" ("元素"), error in (no error)=w2091) -> (queue out=w2089:refnum<queue>, error out=w2090:errorcluster)  [unwired: 2 out]
                    }
                    frame #3 {
                      n1049 = while {
                        tunnel: [w2105] -> w2097
                        i -> [w2110]
                        stop <- w2106 stop-if-true
                        n1050 = property on="Read1_in结果" class="Bool (严格)"() -> ("BoolText.Text"=w2104:string)  [unwired: 2 in, 2 out]
                        n1051 = Greater Or Equal?(x=w2110, y=30) -> (x >= y?=w2107:bool)
                        n1052 = Not Equal?(x=w2104, y="NG" ("布尔文本.文本")) -> (x != y?=w2105:bool)
                        n1053 = Wait Until Next ms Multiple(millisecond multiple=u32 110 ("毫秒倍数")) -> ()  [unwired: 1 out]
                        n1054 = Or(x=w2105, y=w2107) -> (x .or. y?=w2106:bool)
                      }
                      n1055 = case shown="假" w2097 {
                        tunnel: ["内总压AD1值读取NG" "内总压AD1值读取成功"] -> w2094
                        tunnel: [u32 16711680 u32 6618880] -> w2093
                        frame False {
                        }
                        frame True {
                        }
                      }
                      n1056 = control-ref of="结果"() -> (w2095:refnum<vi>)
                      n1057 = Build Array(w2094) -> (w2096:string[])
                      n1058 = call "表格编辑.vi"("新元素/子数组"=w2096, "活动单元格:单元格背景色"=w2093, "MCListbox引用句柄"=w2095) -> ()  [unwired: 9 out]
                    }
                  }
                }
                frame 16 {
                  # "150V外总压AD1"
                  n1059 = flat-sequence {
                    tunnel: w2119 -> [w2125]
                    tunnel: w2120 -> [w2126]
                    tunnel: [w2126] -> w2113
                    tunnel: [w2125] -> w2112
                    tunnel: [w2133] -> w2122
                    tunnel: [w2132] -> w2121
                    tunnel: w2113 -> [w2133]
                    tunnel: w2112 -> [w2132]
                    tunnel: w2122 -> [w2138]
                    tunnel: w2121 -> [w2137]
                    tunnel: [w2136] -> w2116
                    tunnel: [w2135] -> w2115
                    tunnel: [w2144] -> w2118
                    tunnel: [w2145] -> w2117
                    tunnel: w2116 -> [w2145]
                    tunnel: w2115 -> [w2144]
                    tunnel: [w2143] -> w2114
                    frame #0 {
                      n1060 = One Button Dialog(message="请把继电器调到\n外总压状态" ("消息"), button name ("OK")="确定" ("按钮名称（“确定”）")) -> ()  [unwired: 1 out]
                    }
                    frame #1 {
                      n1061 = global write "EV05全局变量1.vi" "CAN接收"(FALSE ("CAN接收")) -> ()
                      n1062 = local write "AD1"(0.0 ("AD1 3")) -> ()
                      n1063 = global write "EV05全局变量1.vi" "高压校正接收"(FALSE ("高压校正接收")) -> ()
                      n1064 = property on="Read1_Out结果" class="Bool (严格)"("Colors [4]"=cluster{u32, u32}[] [{0, 0}] ("颜色[4]"), "BoolText.Text"="" ("布尔文本.文本")) -> ()  [unwired: 2 in, 2 out]
                    }
                    frame #2 {
                      n1065 = Enqueue Element(queue=w2138, element="Read1_out" ("元素"), error in (no error)=w2137) -> (queue out=w2135:refnum<queue>, error out=w2136:errorcluster)  [unwired: 2 out]
                    }
                    frame #3 {
                      n1066 = while {
                        tunnel: [w2151] -> w2143
                        i -> [w2156]
                        stop <- w2152 stop-if-true
                        n1067 = property on="Read1_Out结果" class="Bool (严格)"() -> ("BoolText.Text"=w2150:string)  [unwired: 2 in, 2 out]
                        n1068 = Greater Or Equal?(x=w2156, y=30) -> (x >= y?=w2153:bool)
                        n1069 = Not Equal?(x=w2150, y="NG" ("布尔文本.文本")) -> (x != y?=w2151:bool)
                        n1070 = Or(x=w2151, y=w2153) -> (x .or. y?=w2152:bool)
                        n1071 = Wait Until Next ms Multiple(millisecond multiple=u32 110 ("毫秒倍数")) -> ()  [unwired: 1 out]
                      }
                      n1072 = case shown="真" w2143 {
                        tunnel: ["外总压AD1值读取NG" "外总压AD1值读取成功"] -> w2140
                        tunnel: [u32 16711680 u32 6618880] -> w2139
                        frame False {
                        }
                        frame True {
                        }
                      }
                      n1073 = control-ref of="结果"() -> (w2141:refnum<vi>)
                      n1074 = Build Array(w2140) -> (w2142:string[])
                      n1075 = call "表格编辑.vi"("新元素/子数组"=w2142, "活动单元格:单元格背景色"=w2139, "MCListbox引用句柄"=w2141) -> ()  [unwired: 9 out]
                    }
                  }
                }
                frame 17 {
                  w2171 = "," ("字符串")
                  # "300V"
                  n1076 = local read "Volt2"() -> (w2158:dbl)
                  n1077 = local write "REAL2"(w2158) -> ()
                  n1078 = local write "REAL2"(w2158) -> ()
                  n1079 = local write "Set"(w2158) -> ()
                  n1080 = local write "控制读取  5"(FALSE ("控制读取")) -> ()
                  n1081 = Number To Fractional String(number=w2158, precision (6)=i16 2 ("精度(6)")) -> (F-format string=w2175:string)  [unwired: 2 out]
                  n1082 = Number To Fractional String(number=0.2 ("数字"), precision (6)=i16 2 ("精度(6)")) -> (F-format string=w2174:string)  [unwired: 2 out]
                  n1083 = Number To Fractional String(number=1.0 ("数字"), precision (6)=i16 2 ("精度(6)")) -> (F-format string=w2172:string)  [unwired: 2 out]
                  n1084 = Number To Fractional String(number=320.0 ("数字"), precision (6)=i16 2 ("精度(6)")) -> (F-format string=w2173:string)  [unwired: 2 out]
                  n1085 = Concatenate Strings(w2175, w2171, w2174, w2171, w2173, w2171, w2172, w2171, w2171, w2171) -> (w2170:string)
                  n1086 = flat-sequence {
                    tunnel: [w2194] -> w2186
                    tunnel: [w2193] -> w2185
                    tunnel: [w2192] -> w2184
                    tunnel: w2170 -> [w2189]
                    tunnel: w2162 -> [w2188]
                    tunnel: w2186 -> [w2199]
                    tunnel: [w2199] -> w2183
                    tunnel: w2185 -> [w2198]
                    tunnel: [w2198] -> w2182
                    tunnel: w2184 -> [w2197]
                    tunnel: [w2197] -> w2181
                    tunnel: w2183 -> [w2203]
                    tunnel: w2182 -> [w2202]
                    tunnel: w2181 -> [_]
                    tunnel: [w2201] -> w2180
                    tunnel: [w2200] -> w2179
                    tunnel: w2180 -> [w2209]
                    tunnel: [w2209] -> w2178
                    tunnel: w2179 -> [w2208]
                    tunnel: [w2208] -> w2177
                    tunnel: w2178 -> [w2212]
                    tunnel: w2177 -> [w2211]
                    tunnel: [w2210] -> w2160
                    tunnel: [w2220] -> w2159
                    frame #0 {
                      n1087 = Wait (ms)(milliseconds to wait=u32 50 ("等待时间（毫秒）")) -> ()  [unwired: 1 out]
                    }
                    frame #1 {
                      n1088 = local read "VISA资源名称输出 10"() -> (w2191:refnum<visa-resource-name>)
                      n1089 = Concatenate Strings("SET:GRO 12," ("写入缓冲区"), w2189, "\n") -> (w2192:string)
                      n1090 = VISA Write(VISA resource name=w2191, write buffer=w2192, error in (no error)=w2188) -> (VISA resource name out=w2194:refnum<visa-resource-name>, error out=w2193:errorcluster)  [unwired: 1 out]
                    }
                    frame #2 {
                      n1091 = Wait (ms)(milliseconds to wait=u32 50 ("等待时间（毫秒）")) -> ()  [unwired: 1 out]
                    }
                    frame #3 {
                      n1092 = Concatenate Strings("SET:STE 12" ("写入缓冲区"), "\n") -> (w2204:string)
                      n1093 = VISA Write(VISA resource name=w2203, write buffer=w2204, error in (no error)=w2202) -> (VISA resource name out=w2201:refnum<visa-resource-name>, error out=w2200:errorcluster)  [unwired: 1 out]
                    }
                    frame #4 {
                      n1094 = Wait (ms)(milliseconds to wait=u32 200 ("等待时间（毫秒）")) -> ()  [unwired: 1 out]
                    }
                    frame #5 {
                      n1095 = Concatenate Strings("OUT:ON" ("写入缓冲区"), "\n") -> (w2217:string)
                      n1096 = Wait (ms)(milliseconds to wait=u32 50 ("等待时间（毫秒）")) -> ()  [unwired: 1 out]
                      n1097 = VISA Write(VISA resource name=w2212, write buffer=w2217, error in (no error)=w2211) -> (VISA resource name out=w2214:refnum<visa-resource-name>, error out=w2210:errorcluster)  [unwired: 1 out]
                      n1098 = local write "VISA资源名称输出 10"(w2214) -> ()
                    }
                    frame #6 {
                      n1099 = while {
                        tunnel: [w2225] -> w2220
                        i -> [w2226]
                        stop <- w2224 stop-if-true
                        n1100 = local read "Volt2"() -> (w2230:dbl)
                        n1101 = local read "Actual"() -> (w2231:dbl)
                        n1102 = Greater Or Equal?(x=w2226, y=20) -> (x >= y?=w2228:bool)
                        n1103 = Multiply(x=w2230, y=0.02) -> (x*y=w2232:dbl)
                        n1104 = Add(x=w2230, y=w2232) -> (x+y=w2234:dbl)
                        n1105 = Subtract(x=w2230, y=w2232) -> (x-y=w2233:dbl)
                        n1106 = Wait Until Next ms Multiple(millisecond multiple=u32 200 ("毫秒倍数")) -> ()  [unwired: 1 out]
                        n1107 = In Range and Coerce(upper limit=w2234, x=w2231, lower limit=w2233) -> (In Range?=w2225:bool)  [unwired: 1 out]
                        n1108 = Or(x=w2225, y=w2228) -> (x .or. y?=w2224:bool)
                      }
                      n1109 = case shown="真" w2220 {
                        tunnel: ["300V电压开启NG" "300V电压开启成功"] -> w2219
                        tunnel: [u32 16711680 u32 6618880] -> w2218
                        frame False {
                        }
                        frame True {
                        }
                      }
                      n1110 = control-ref of="结果"() -> (w2222:refnum<vi>)
                      n1111 = Build Array(w2219) -> (w2221:string[])
                      n1112 = local write "控制读取  5"(TRUE ("控制读取")) -> ()
                      n1113 = call "表格编辑.vi"("新元素/子数组"=w2221, "活动单元格:单元格背景色"=w2218, "MCListbox引用句柄"=w2222) -> ()  [unwired: 9 out]
                    }
                  }
                }
                frame 18 {
                  # "300V内总压AD2"
                  n1114 = flat-sequence {
                    tunnel: w2247 -> [w2253]
                    tunnel: w2248 -> [w2254]
                    tunnel: [w2254] -> w2241
                    tunnel: [w2253] -> w2240
                    tunnel: [w2261] -> w2250
                    tunnel: [w2260] -> w2249
                    tunnel: w2241 -> [w2261]
                    tunnel: w2240 -> [w2260]
                    tunnel: w2250 -> [w2266]
                    tunnel: w2249 -> [w2265]
                    tunnel: [w2264] -> w2244
                    tunnel: [w2263] -> w2243
                    tunnel: [w2272] -> w2246
                    tunnel: [w2273] -> w2245
                    tunnel: w2244 -> [w2273]
                    tunnel: w2243 -> [w2272]
                    tunnel: [w2271] -> w2242
                    frame #0 {
                      n1115 = One Button Dialog(message="请把继电器调到\n内总压状态" ("消息"), button name ("OK")="确定" ("按钮名称（“确定”）")) -> ()  [unwired: 1 out]
                    }
                    frame #1 {
                      n1116 = global write "EV05全局变量1.vi" "CAN接收"(FALSE ("CAN接收")) -> ()
                      n1117 = global write "EV05全局变量1.vi" "高压校正接收"(FALSE ("高压校正接收")) -> ()
                      n1118 = local write "AD2"(0.0 ("AD2 2")) -> ()
                      n1119 = property on="Read2_in结果" class="Bool (严格)"("Colors [4]"=cluster{u32, u32}[] [{0, 0}] ("颜色[4]"), "BoolText.Text"="" ("布尔文本.文本")) -> ()  [unwired: 2 in, 2 out]
                    }
                    frame #2 {
                      n1120 = Enqueue Element(queue=w2266, element="Read2_in" ("元素"), error in (no error)=w2265) -> (queue out=w2263:refnum<queue>, error out=w2264:errorcluster)  [unwired: 2 out]
                    }
                    frame #3 {
                      n1121 = while {
                        tunnel: [w2279] -> w2271
                        i -> [w2284]
                        stop <- w2280 stop-if-true
                        n1122 = property on="Read2_in结果" class="Bool (严格)"() -> ("BoolText.Text"=w2278:string)  [unwired: 2 in, 2 out]
                        n1123 = Greater Or Equal?(x=w2284, y=30) -> (x >= y?=w2281:bool)
                        n1124 = Not Equal?(x=w2278, y="NG" ("布尔文本.文本")) -> (x != y?=w2279:bool)
                        n1125 = Or(x=w2279, y=w2281) -> (x .or. y?=w2280:bool)
                        n1126 = Wait Until Next ms Multiple(millisecond multiple=u32 110 ("毫秒倍数")) -> ()  [unwired: 1 out]
                      }
                      n1127 = case shown="真" w2271 {
                        tunnel: ["内总压AD2值读取NG" "内总压AD2值读取成功"] -> w2268
                        tunnel: [u32 16711680 u32 6618880] -> w2267
                        frame False {
                        }
                        frame True {
                        }
                      }
                      n1128 = control-ref of="结果"() -> (w2269:refnum<vi>)
                      n1129 = Build Array(w2268) -> (w2270:string[])
                      n1130 = call "表格编辑.vi"("新元素/子数组"=w2270, "活动单元格:单元格背景色"=w2267, "MCListbox引用句柄"=w2269) -> ()  [unwired: 9 out]
                    }
                  }
                }
                frame 19 {
                  # "300V外总压AD2"
                  n1131 = flat-sequence {
                    tunnel: w2293 -> [w2299]
                    tunnel: w2294 -> [w2300]
                    tunnel: [w2300] -> w2287
                    tunnel: [w2299] -> w2286
                    tunnel: [w2307] -> w2296
                    tunnel: [w2306] -> w2295
                    tunnel: w2287 -> [w2307]
                    tunnel: w2286 -> [w2306]
                    tunnel: w2296 -> [w2312]
                    tunnel: w2295 -> [w2311]
                    tunnel: [w2310] -> w2290
                    tunnel: [w2309] -> w2289
                    tunnel: [w2318] -> w2292
                    tunnel: [w2319] -> w2291
                    tunnel: w2290 -> [w2319]
                    tunnel: w2289 -> [w2318]
                    tunnel: [w2317] -> w2288
                    frame #0 {
                      n1132 = One Button Dialog(message="请把继电器调到\n外总压状态" ("消息"), button name ("OK")="确定" ("按钮名称（“确定”）")) -> ()  [unwired: 1 out]
                    }
                    frame #1 {
                      n1133 = global write "EV05全局变量1.vi" "CAN接收"(FALSE ("CAN接收")) -> ()
                      n1134 = global write "EV05全局变量1.vi" "高压校正接收"(FALSE ("高压校正接收")) -> ()
                      n1135 = local write "AD2"(0.0 ("AD2 3")) -> ()
                      n1136 = property on="Read2_Out结果" class="Bool (严格)"("Colors [4]"=cluster{u32, u32}[] [{0, 0}] ("颜色[4]"), "BoolText.Text"="" ("布尔文本.文本")) -> ()  [unwired: 2 in, 2 out]
                    }
                    frame #2 {
                      n1137 = Enqueue Element(queue=w2312, element="Read1_in" ("元素"), error in (no error)=w2311) -> (queue out=w2309:refnum<queue>, error out=w2310:errorcluster)  [unwired: 2 out]
                    }
                    frame #3 {
                      n1138 = while {
                        tunnel: [w2325] -> w2317
                        i -> [w2330]
                        stop <- w2326 stop-if-true
                        n1139 = property on="Read2_Out结果" class="Bool (严格)"() -> ("BoolText.Text"=w2324:string)  [unwired: 2 in, 2 out]
                        n1140 = Greater Or Equal?(x=w2330, y=30) -> (x >= y?=w2327:bool)
                        n1141 = Not Equal?(x=w2324, y="NG" ("布尔文本.文本")) -> (x != y?=w2325:bool)
                        n1142 = Or(x=w2325, y=w2327) -> (x .or. y?=w2326:bool)
                        n1143 = Wait Until Next ms Multiple(millisecond multiple=u32 110 ("毫秒倍数")) -> ()  [unwired: 1 out]
                      }
                      n1144 = case shown="真" w2317 {
                        tunnel: ["外总压AD2值读取NG" "外总压AD2值读取成功"] -> w2314
                        tunnel: [u32 16711680 u32 6618880] -> w2313
                        frame False {
                        }
                        frame True {
                        }
                      }
                      n1145 = control-ref of="结果"() -> (w2315:refnum<vi>)
                      n1146 = Build Array(w2314) -> (w2316:string[])
                      n1147 = call "表格编辑.vi"("新元素/子数组"=w2316, "活动单元格:单元格背景色"=w2313, "MCListbox引用句柄"=w2315) -> ()  [unwired: 9 out]
                    }
                  }
                }
                frame 20 {
                  # "SET内总压"
                  n1148 = flat-sequence {
                    tunnel: w2337 -> [w2351]
                    tunnel: w2338 -> [w2352]
                    tunnel: [w2352] -> w2340
                    tunnel: [w2351] -> w2339
                    tunnel: w2340 -> [w2357]
                    tunnel: w2339 -> [w2356]
                    tunnel: [w2355] -> w2334
                    tunnel: [w2354] -> w2333
                    tunnel: [w2363] -> w2336
                    tunnel: [w2364] -> w2335
                    tunnel: w2334 -> [w2364]
                    tunnel: w2333 -> [w2363]
                    tunnel: [w2362] -> w2332
                    frame #0 {
                      n1149 = local read "REAL2"() -> (w2349:dbl)
                      n1150 = local read "REAL1"() -> (w2350:dbl)
                      n1151 = local read "AD1"() -> (w2348:dbl)
                      n1152 = local read "AD2"() -> (w2347:dbl)
                      n1153 = global write "EV05全局变量1.vi" "CAN接收"(FALSE ("CAN接收")) -> ()
                      n1154 = global write "EV05全局变量1.vi" "高压校正接收"(FALSE ("高压校正接收")) -> ()
                      n1155 = call "Cal_Gain&offset.vi"("REAL2"=w2349, "REAL1"=w2350, "AD2"=w2347, "AD1"=w2348) -> ("Offset"=w2345:i32, "Gain"=w2346:dbl)  [unwired: 5 out]
                      n1156 = local write "Offset"(w2345) -> ()
                      n1157 = local write "Gain"(w2346) -> ()
                      n1158 = property on="Set_in结果" class="Bool (严格)"("Colors [4]"=cluster{u32, u32}[] [{0, 0}] ("颜色[4]"), "BoolText.Text"="" ("布尔文本.文本")) -> ()  [unwired: 2 in, 2 out]
                    }
                    frame #1 {
                      n1159 = Enqueue Element(queue=w2357, element="Set_in" ("元素"), error in (no error)=w2356) -> (queue out=w2354:refnum<queue>, error out=w2355:errorcluster)  [unwired: 2 out]
                    }
                    frame #2 {
                      n1160 = while {
                        tunnel: [w2370] -> w2362
                        i -> [w2375]
                        stop <- w2371 stop-if-true
                        n1161 = property on="Set_in结果" class="Bool (严格)"() -> ("BoolText.Text"=w2369:string)  [unwired: 2 in, 2 out]
                        n1162 = Greater Or Equal?(x=w2375, y=30) -> (x >= y?=w2372:bool)
                        n1163 = Not Equal?(x=w2369, y="NG" ("布尔文本.文本")) -> (x != y?=w2370:bool)
                        n1164 = Or(x=w2370, y=w2372) -> (x .or. y?=w2371:bool)
                        n1165 = Wait Until Next ms Multiple(millisecond multiple=u32 110 ("毫秒倍数")) -> ()  [unwired: 1 out]
                      }
                      n1166 = case shown="真" w2362 {
                        tunnel: ["内总压参数写入NG" "内总压参数写入成功"] -> w2358
                        tunnel: [u32 16711680 u32 6618880] -> w2359
                        frame False {
                        }
                        frame True {
                        }
                      }
                      n1167 = control-ref of="结果"() -> (w2360:refnum<vi>)
                      n1168 = Build Array(w2358) -> (w2361:string[])
                      n1169 = call "表格编辑.vi"("新元素/子数组"=w2361, "活动单元格:单元格背景色"=w2359, "MCListbox引用句柄"=w2360) -> ()  [unwired: 9 out]
                    }
                  }
                }
                frame 21 {
                  # "SET外总压"
                  n1170 = flat-sequence {
                    tunnel: w2382 -> [w2396]
                    tunnel: w2383 -> [w2397]
                    tunnel: [w2397] -> w2385
                    tunnel: [w2396] -> w2384
                    tunnel: w2385 -> [w2402]
                    tunnel: w2384 -> [w2401]
                    tunnel: [w2400] -> w2379
                    tunnel: [w2399] -> w2378
                    tunnel: [w2408] -> w2381
                    tunnel: [w2409] -> w2380
                    tunnel: w2379 -> [w2409]
                    tunnel: w2378 -> [w2408]
                    tunnel: [w2407] -> w2377
                    frame #0 {
                      n1171 = local read "REAL2"() -> (w2389:dbl)
                      n1172 = local read "REAL1"() -> (w2388:dbl)
                      n1173 = local read "AD1"() -> (w2390:dbl)
                      n1174 = local read "AD2"() -> (w2391:dbl)
                      n1175 = global write "EV05全局变量1.vi" "CAN接收"(FALSE ("CAN接收")) -> ()
                      n1176 = global write "EV05全局变量1.vi" "高压校正接收"(FALSE ("高压校正接收")) -> ()
                      n1177 = call "Cal_Gain&offset.vi"("REAL2"=w2389, "REAL1"=w2388, "AD2"=w2391, "AD1"=w2390) -> ("Offset"=w2392:i32, "Gain"=w2393:dbl)  [unwired: 5 out]
                      n1178 = local write "Gain"(w2393) -> ()
                      n1179 = local write "Offset"(w2392) -> ()
                      n1180 = property on="Set_out结果" class="Bool (严格)"("Colors [4]"=cluster{u32, u32}[] [{0, 0}] ("颜色[4]"), "BoolText.Text"="" ("布尔文本.文本")) -> ()  [unwired: 2 in, 2 out]
                    }
                    frame #1 {
                      n1181 = Enqueue Element(queue=w2402, element="Set_out" ("元素"), error in (no error)=w2401) -> (queue out=w2399:refnum<queue>, error out=w2400:errorcluster)  [unwired: 2 out]
                    }
                    frame #2 {
                      n1182 = while {
                        tunnel: [w2415] -> w2407
                        i -> [w2420]
                        stop <- w2416 stop-if-true
                        n1183 = property on="Set_out结果" class="Bool (严格)"() -> ("BoolText.Text"=w2414:string)  [unwired: 2 in, 2 out]
                        n1184 = Greater Or Equal?(x=w2420, y=30) -> (x >= y?=w2417:bool)
                        n1185 = Not Equal?(x=w2414, y="NG" ("布尔文本.文本")) -> (x != y?=w2415:bool)
                        n1186 = Or(x=w2415, y=w2417) -> (x .or. y?=w2416:bool)
                        n1187 = Wait Until Next ms Multiple(millisecond multiple=u32 110 ("毫秒倍数")) -> ()  [unwired: 1 out]
                      }
                      n1188 = case shown="假" w2407 {
                        tunnel: ["外总压参数写入NG" "外总压参数写入成功"] -> w2403
                        tunnel: [u32 16711680 u32 6618880] -> w2404
                        frame False {
                        }
                        frame True {
                        }
                      }
                      n1189 = control-ref of="结果"() -> (w2405:refnum<vi>)
                      n1190 = Build Array(w2403) -> (w2406:string[])
                      n1191 = call "表格编辑.vi"("新元素/子数组"=w2406, "活动单元格:单元格背景色"=w2404, "MCListbox引用句柄"=w2405) -> ()  [unwired: 9 out]
                    }
                  }
                }
                frame 22 {
                  w2449 = "," ("字符串")
                  # "检验电压校正状态"
                  n1192 = flat-sequence {
                    tunnel: [w2474] -> w2429
                    tunnel: [w2465] -> w2422
                    tunnel: [w2483] -> w2430
                    tunnel: w2429 -> [w2483]
                    tunnel: [w2482] -> w2423
                    tunnel: w2422 -> [w2482]
                    tunnel: [w2493] -> w2464
                    tunnel: [w2492] -> w2463
                    tunnel: [w2491] -> w2462
                    tunnel: w2448 -> [w2488]
                    tunnel: w2440 -> [w2487]
                    tunnel: [w2486] -> w2431
                    tunnel: w2430 -> [w2486]
                    tunnel: [w2485] -> w2424
                    tunnel: w2423 -> [w2485]
                    tunnel: w2464 -> [w2500]
                    tunnel: [w2500] -> w2461
                    tunnel: w2463 -> [w2499]
                    tunnel: [w2499] -> w2460
                    tunnel: w2462 -> [w2498]
                    tunnel: [w2498] -> w2459
                    tunnel: [w2496] -> w2432
                    tunnel: w2431 -> [w2496]
                    tunnel: [w2495] -> w2425
                    tunnel: w2424 -> [w2495]
                    tunnel: w2461 -> [w2506]
                    tunnel: w2460 -> [w2505]
                    tunnel: w2459 -> [_]
                    tunnel: [w2504] -> w2458
                    tunnel: [w2503] -> w2457
                    tunnel: [w2502] -> w2433
                    tunnel: w2432 -> [w2502]
                    tunnel: [w2501] -> w2426
                    tunnel: w2425 -> [w2501]
                    tunnel: w2458 -> [w2514]
                    tunnel: [w2514] -> w2456
                    tunnel: w2457 -> [w2513]
                    tunnel: [w2513] -> w2455
                    tunnel: [w2511] -> w2434
                    tunnel: w2433 -> [w2511]
                    tunnel: [w2510] -> w2427
                    tunnel: w2426 -> [w2510]
                    tunnel: w2456 -> [w2519]
                    tunnel: w2455 -> [w2518]
                    tunnel: [w2517] -> w2438
                    tunnel: [w2516] -> w2435
                    tunnel: w2434 -> [w2516]
                    tunnel: [w2515] -> w2428
                    tunnel: w2427 -> [w2515]
                    tunnel: [w2525] -> w2437
                    tunnel: w2435 -> [w2527]
                    tunnel: w2428 -> [w2526]
                    frame #0 {
                      n1193 = local read "外总压"() -> (w2468:dbl)
                      n1194 = local read "内总压"() -> (w2475:dbl)
                      n1195 = local read "Actual"() -> (w2467:dbl)
                      n1196 = Subtract(x=w2475, y=w2467) -> (x-y=w2480:dbl)
                      n1197 = Subtract(x=w2467, y=w2468) -> (x-y=w2470:dbl)
                      n1198 = Absolute Value(x=w2480) -> (abs(x)=w2481:dbl)
                      n1199 = Absolute Value(x=w2470) -> (abs(x)=w2469:dbl)
                      n1200 = Divide(x=w2481, y=w2467) -> (x/y=w2477:dbl)
                      n1201 = Divide(x=w2469, y=w2467) -> (x/y=w2473:dbl)
                      n1202 = Multiply(x=w2477, y=100.0) -> (x*y=w2478:dbl)
                      n1203 = Multiply(x=w2473, y=100.0) -> (x*y=w2472:dbl)
                      n1204 = Format Into String(format string="%.3f%" ("格式字符串"), w2478) -> (resulting string=w2474:string)  [unwired: 2 in, 1 out]
                      n1205 = Format Into String(format string="%.3f%" ("格式字符串"), w2472) -> (resulting string=w2465:string)  [unwired: 2 in, 1 out]
                    }
                    frame #1 {
                      n1206 = Wait (ms)(milliseconds to wait=u32 50 ("等待时间（毫秒）")) -> ()  [unwired: 1 out]
                    }
                    frame #2 {
                      n1207 = local read "VISA资源名称输出 10"() -> (w2490:refnum<visa-resource-name>)
                      n1208 = Concatenate Strings("SET:GRO 12," ("写入缓冲区"), w2488, "\n") -> (w2491:string)
                      n1209 = VISA Write(VISA resource name=w2490, write buffer=w2491, error in (no error)=w2487) -> (VISA resource name out=w2493:refnum<visa-resource-name>, error out=w2492:errorcluster)  [unwired: 1 out]
                    }
                    frame #3 {
                      n1210 = Wait (ms)(milliseconds to wait=u32 50 ("等待时间（毫秒）")) -> ()  [unwired: 1 out]
                    }
                    frame #4 {
                      n1211 = Concatenate Strings("SET:STE 12" ("写入缓冲区"), "\n") -> (w2507:string)
                      n1212 = VISA Write(VISA resource name=w2506, write buffer=w2507, error in (no error)=w2505) -> (VISA resource name out=w2504:refnum<visa-resource-name>, error out=w2503:errorcluster)  [unwired: 1 out]
                    }
                    frame #5 {
                      n1213 = Wait (ms)(milliseconds to wait=u32 200 ("等待时间（毫秒）")) -> ()  [unwired: 1 out]
                    }
                    frame #6 {
                      n1214 = Concatenate Strings("OUT:ON" ("写入缓冲区"), "\n") -> (w2524:string)
                      n1215 = Wait (ms)(milliseconds to wait=u32 50 ("等待时间（毫秒）")) -> ()  [unwired: 1 out]
                      n1216 = VISA Write(VISA resource name=w2519, write buffer=w2524, error in (no error)=w2518) -> (VISA resource name out=w2521:refnum<visa-resource-name>, error out=w2517:errorcluster)  [unwired: 1 out]
                      n1217 = local write "VISA资源名称输出 10"(w2521) -> ()
                    }
                    frame #7 {
                      n1218 = stacked-sequence {
                        seq-local: [w2528 _ _ _] -> [_ w2541 _ _]
                        tunnel: w2527 -> [_ _ w2552 _]
                        tunnel: w2526 -> [_ _ _ w2568]
                        tunnel: [w2528 _ _ _] -> w2525
                        frame #0 {
                          n1219 = while {
                            tunnel: [w2531] -> w2528
                            i -> [w2532]
                            stop <- w2530 stop-if-true
                            w2529 = 150.0 ("x")
                            n1220 = local read "Actual"() -> (w2536:dbl)
                            n1221 = Greater Or Equal?(x=w2532, y=20) -> (x >= y?=w2534:bool)
                            n1222 = Multiply(x=w2529, y=0.02) -> (x*y=w2537:dbl)
                            n1223 = Add(x=w2529, y=w2537) -> (x+y=w2539:dbl)
                            n1224 = Subtract(x=w2529, y=w2537) -> (x-y=w2538:dbl)
                            n1225 = Wait Until Next ms Multiple(millisecond multiple=u32 200 ("毫秒倍数")) -> ()  [unwired: 1 out]
                            n1226 = In Range and Coerce(upper limit=w2539, x=w2536, lower limit=w2538) -> (In Range?=w2531:bool)  [unwired: 1 out]
                            n1227 = Or(x=w2531, y=w2534) -> (x .or. y?=w2530:bool)
                          }
                        }
                        frame #1 {
                          n1228 = case shown="假" w2541 {
                            tunnel: ["150V电压开启NG" "150V电压开启成功"] -> w2543
                            tunnel: [u32 16711680 u32 6618880] -> w2542
                            frame False {
                            }
                            frame True {
                            }
                          }
                          n1229 = control-ref of="结果"() -> (w2545:refnum<vi>)
                          n1230 = Build Array(w2543) -> (w2544:string[])
                          n1231 = call "表格编辑.vi"("新元素/子数组"=w2544, "活动单元格:单元格背景色"=w2542, "MCListbox引用句柄"=w2545) -> ()  [unwired: 9 out]
                        }
                        frame #2 {
                          n1232 = local read "Actual"() -> (w2554:dbl)
                          n1233 = local read "内总压"() -> (w2553:dbl)
                          n1234 = Subtract(x=w2554, y=w2553) -> (x-y=w2562:dbl)
                          n1235 = Absolute Value(x=w2562) -> (abs(x)=w2563:dbl)
                          n1236 = Divide(x=w2563, y=w2554) -> (x/y=w2558:dbl)
                          n1237 = Multiply(x=w2558, y=100.0) -> (x*y=w2559:dbl)
                          n1238 = Format Into String(format string="%.3f%" ("格式字符串"), w2559) -> (resulting string=w2551:string)  [unwired: 2 in, 1 out]
                          n1239 = Concatenate Strings("内总压150V误差", w2551, "  300V误差", w2552) -> (w2555:string)
                          n1240 = control-ref of="结果"() -> (w2565:refnum<vi>)
                          n1241 = local write "控制读取  5"(TRUE ("控制读取")) -> ()
                          n1242 = Build Array(w2555) -> (w2564:string[])
                          n1243 = call "表格编辑.vi"("新元素/子数组"=w2564, "活动单元格:单元格背景色"=u32 6618880, "MCListbox引用句柄"=w2565) -> ()  [unwired: 9 out]
                        }
                        frame #3 {
                          n1244 = local read "Actual"() -> (w2571:dbl)
                          n1245 = local read "外总压"() -> (w2569:dbl)
                          n1246 = Subtract(x=w2571, y=w2569) -> (x-y=w2579:dbl)
                          n1247 = Absolute Value(x=w2579) -> (abs(x)=w2580:dbl)
                          n1248 = Divide(x=w2580, y=w2571) -> (x/y=w2575:dbl)
                          n1249 = Multiply(x=w2575, y=100.0) -> (x*y=w2576:dbl)
                          n1250 = Format Into String(format string="%.3f%" ("格式字符串"), w2576) -> (resulting string=w2570:string)  [unwired: 2 in, 1 out]
                          n1251 = Concatenate Strings("外总压150V误差", w2570, "  300V误差", w2568) -> (w2572:string)
                          n1252 = control-ref of="结果"() -> (w2582:refnum<vi>)
                          n1253 = Build Array(w2572) -> (w2581:string[])
                          n1254 = call "表格编辑.vi"("新元素/子数组"=w2581, "活动单元格:单元格背景色"=u32 6618880, "MCListbox引用句柄"=w2582) -> ()  [unwired: 9 out]
                        }
                      }
                    }
                  }
                  n1255 = Number To Fractional String(number=150.0 ("数字"), precision (6)=i16 2 ("精度(6)")) -> (F-format string=w2453:string)  [unwired: 2 out]
                  n1256 = Number To Fractional String(number=0.2 ("数字"), precision (6)=i16 2 ("精度(6)")) -> (F-format string=w2452:string)  [unwired: 2 out]
                  n1257 = Number To Fractional String(number=320.0 ("数字"), precision (6)=i16 2 ("精度(6)")) -> (F-format string=w2451:string)  [unwired: 2 out]
                  n1258 = Number To Fractional String(number=1.0 ("数字"), precision (6)=i16 2 ("精度(6)")) -> (F-format string=w2450:string)  [unwired: 2 out]
                  n1259 = Concatenate Strings(w2453, w2449, w2452, w2449, w2451, w2449, w2450, w2449, w2449, w2449) -> (w2448:string)
                  n1260 = local write "控制读取  5"(FALSE ("控制读取")) -> ()
                }
                frame 23 {
                  # "关闭电压源"
                  n1261 = local read "VISA资源名称输出 10"() -> (w2589:refnum<visa-resource-name>)
                  n1262 = local write "控制读取  5"(FALSE ("控制读取")) -> ()
                  n1263 = flat-sequence {
                    tunnel: [w2596] -> w2594
                    tunnel: w2589 -> [w2596]
                    tunnel: w2594 -> [w2600]
                    tunnel: [w2599] -> w2593
                    tunnel: [w2598] -> w2592
                    tunnel: w2587 -> [w2597]
                    tunnel: w2593 -> [w2604]
                    tunnel: w2592 -> [w2603]
                    tunnel: [w2604] -> w2591
                    tunnel: [w2603] -> w2590
                    tunnel: w2591 -> [w2608]
                    tunnel: w2590 -> [w2607]
                    tunnel: [w2605] -> w2584
                    tunnel: [w2615] -> w2586
                    tunnel: w2584 -> [w2615]
                    tunnel: [FALSE ("status")] -> w2583
                    frame #0 {
                      n1264 = Wait (ms)(milliseconds to wait=u32 50 ("等待时间（毫秒）")) -> ()  [unwired: 1 out]
                    }
                    frame #1 {
                      n1265 = VISA Write(VISA resource name=w2600, write buffer="OUT:OFF" ("写入缓冲区"), error in (no error)=w2597) -> (VISA resource name out=w2599:refnum<visa-resource-name>, error out=w2598:errorcluster)  [unwired: 1 out]
                    }
                    frame #2 {
                      n1266 = Wait (ms)(milliseconds to wait=u32 50 ("等待时间（毫秒）")) -> ()  [unwired: 1 out]
                    }
                    frame #3 {
                      n1267 = local write "控制读取  5"(TRUE ("控制读取")) -> ()
                      n1268 = VISA Write(VISA resource name=w2608, write buffer="OUT:OFF" ("写入缓冲区"), error in (no error)=w2607) -> (error out=w2605:errorcluster)  [unwired: 2 out]
                    }
                    frame #4 {
                      n1269 = control-ref of="结果"() -> (w2612:refnum<vi>)
                      n1270 = Build Array("电压源关闭") -> (w2613:string[])
                      n1271 = call "表格编辑.vi"("新元素/子数组"=w2613, "活动单元格:单元格背景色"=u32 6618880, "MCListbox引用句柄"=w2612) -> ()  [unwired: 9 out]
                    }
                  }
                }
                frame 24 {
                  # "分流器型号"
                  n1272 = local read "分流器大小"() -> (w2621:T2)
                  n1273 = case shown="\"100A\", 默认" w2621 {
                    selector: w2621 -> [_ w2628]
                    tunnel: w2620 -> [w2626 w2635]
                    tunnel: w2619 -> [w2625 w2634]
                    tunnel: [w2625 w2633] -> w2617
                    tunnel: [w2626 w2632] -> w2618
                    tunnel: [TRUE ("status") w2629] -> w2616
                    frame "选择分流器型号" {
                      n1274 = One Button Dialog(message="分流器为无效值" ("消息"), button name ("OK")="确定" ("按钮名称（“确定”）")) -> ()  [unwired: 1 out]
                    }
                    frame "100A", Default {
                      n1275 = flat-sequence {
                        tunnel: w2634 -> [w2652]
                        tunnel: w2635 -> [w2653]
                        tunnel: [w2653] -> w2637
                        tunnel: [w2652] -> w2636
                        tunnel: w2637 -> [w2658]
                        tunnel: w2636 -> [w2657]
                        tunnel: [w2656] -> w2631
                        tunnel: [w2655] -> w2630
                        tunnel: [w2666] -> w2632
                        tunnel: [w2667] -> w2633
                        tunnel: w2631 -> [w2667]
                        tunnel: w2630 -> [w2666]
                        tunnel: [TRUE ("status")] -> w2629
                        tunnel: w2627 -> [w2659]
                        frame #0 {
                          n1276 = global write "EV05全局变量1.vi" "CAN接收"(FALSE ("CAN接收")) -> ()
                          n1277 = global write "EV05全局变量1.vi" "高压校正接收"(FALSE ("高压校正接收")) -> ()
                          n1278 = property on="Current Gain结果 4" class="Bool (严格)"("Colors [4]"=cluster{u32, u32}[] [{0, 0}] ("颜色[4]"), "BoolText.Text"="" ("布尔文本.文本")) -> ()  [unwired: 2 in, 2 out]
                        }
                        frame #1 {
                          n1279 = Enqueue Element(queue=w2658, element="Set Current Gain 4" ("元素"), error in (no error)=w2657) -> (queue out=w2655:refnum<queue>, error out=w2656:errorcluster)  [unwired: 2 out]
                        }
                        frame #2 {
                          n1280 = while {
                            tunnel: [w2679] -> w2661
                            i -> [w2684]
                            stop <- w2680 stop-if-true
                            n1281 = property on="Current Gain结果 4" class="Bool (严格)"() -> ("BoolText.Text"=w2678:string)  [unwired: 2 in, 2 out]
                            n1282 = Greater Or Equal?(x=w2684, y=30) -> (x >= y?=w2681:bool)
                            n1283 = Not Equal?(x=w2678, y="NG" ("布尔文本.文本")) -> (x != y?=w2679:bool)
                            n1284 = Or(x=w2679, y=w2681) -> (x .or. y?=w2680:bool)
                            n1285 = Wait Until Next ms Multiple(millisecond multiple=u32 110 ("毫秒倍数")) -> ()  [unwired: 1 out]
                          }
                          n1286 = case shown="假" w2661 {
                            tunnel: [w2668 w2673] -> w2662
                            tunnel: [u32 16711680 u32 6618880] -> w2663
                            tunnel: w2659 -> [w2670 w2675]
                            frame False {
                              n1287 = Concatenate Strings("分流器", w2670, " 写入NG") -> (w2668:string)
                            }
                            frame True {
                              n1288 = Concatenate Strings("分流器", w2675, " 写入成功") -> (w2673:string)
                            }
                          }
                          n1289 = control-ref of="结果"() -> (w2664:refnum<vi>)
                          n1290 = Build Array(w2662) -> (w2665:string[])
                          n1291 = call "表格编辑.vi"("新元素/子数组"=w2665, "活动单元格:单元格背景色"=w2663, "MCListbox引用句柄"=w2664) -> ()  [unwired: 9 out]
                        }
                      }
                      n1292 = case shown="\"100A\", 默认" w2628 {
                        tunnel: ["100A" "200A" "300A" "400A" "500A" "600A" "700A" "800A" "900A" "1000A"] -> w2627
                        frame "100A", Default {
                        }
                        frame "200A" {
                        }
                        frame "300A" {
                        }
                        frame "400A" {
                        }
                        frame "500A" {
                        }
                        frame "600A" {
                        }
                        frame "700A" {
                        }
                        frame "800A" {
                        }
                        frame "900A" {
                        }
                        frame "1000A" {
                        }
                      }
                    }
                  }
                }
              }
              n1293 = call <vilib>:"Set Busy.vi"() -> ()  [unwired: 10 in, 2 out]
              n1294 = case shown="假" w1275 {
                tunnel: ["校正完成" "校正NG"] -> w1272
                tunnel: [u32 6618880 u32 16711680] -> w1271
                frame False {
                  n1295 = call <vilib>:"Unset Busy.vi"() -> ()  [unwired: 11 in, 1 out]
                }
                frame True {
                }
              }
              n1296 = control-ref of="结果"() -> (w1274:refnum<vi>)
              n1297 = Build Array(w1272) -> (w1273:string[])
              n1298 = call "表格编辑.vi"("新元素/子数组"=w1273, "活动单元格:单元格背景色"=w1271, "MCListbox引用句柄"=w1274) -> ()  [unwired: 9 out]
            }
          }
        }
      }
      event "记录": Value Change {
        n1299 = event-data() -> ("NewVal"=w2686:bool)  [unwired: 6 out]
        n1300 = case shown="真" w2686 {
          frame False {
          }
          frame True {
            n1301 = call "当前时间解析-8.6.vi"() -> ("名称格式时间"=w2697:string)  [unwired: 1 in, 18 out]
            n1302 = call <vilib>:"Application Directory.vi"() -> ("Application Directory"=w2687:path)
            n1303 = Concatenate Strings(w2697, ".ini" ("字符串")) -> (w2701:string)
            n1304 = call "路径分析-8.6.vi"("第二个文件夹"="高压校正数据" ("第一个文件夹"), "第一个文件夹"="SaveData", "输入路径"=w2687) -> ("输出路径"=w2699:path)  [unwired: 8 in]
            n1305 = stacked-sequence {
              tunnel: [_ w2738 _] -> w2690
              tunnel: [_ _ w2755] -> w2689
              tunnel: [w2711 _ _] -> w2691
              frame #0 {
                n1306 = local read "REAL2"() -> (w2714:dbl)
                n1307 = local read "REAL1"() -> (w2712:dbl)
                n1308 = local read "Shunt Volt Offset"() -> (w2717:string)
                n1309 = local read "Gain"() -> (w2723:dbl)
                n1310 = local read "分流器大小"() -> (w2724:T2)
                n1311 = local read "AD1"() -> (w2713:u16)
                n1312 = local read "AD2"() -> (w2715:u16)
                n1313 = local read "Shunt Volt Gain"() -> (w2716:string)
                n1314 = local read "电流零点"() -> (w2719:string)
                n1315 = local read "电流增益"() -> (w2718:string)
                n1316 = Build Array(w2712, w2713, w2714, w2715, w2723) -> (w2722:dbl[])
                n1317 = case shown="\"100A\", 默认" w2724 {
                  tunnel: ["100A" "200A" "300A" "400A" "500A" "600A" "700A" "800A" "900A" "1000A"] -> w2720
                  frame "100A", Default {
                  }
                  frame "200A" {
                  }
                  frame "300A" {
                  }
                  frame "400A" {
                  }
                  frame "500A" {
                  }
                  frame "600A" {
                  }
                  frame "700A" {
                  }
                  frame "800A" {
                  }
                  frame "900A" {
                  }
                  frame "1000A" {
                  }
                }
                n1318 = for {
                  tunnel: w2722 -> [w2726] mode=indexing
                  tunnel: [w2725] -> w2721 mode=indexing
                  n1319 = Format Into String(format string="%#f" ("格式字符串"), w2726) -> (resulting string=w2725:string)  [unwired: 2 in, 1 out]
                }
                n1320 = Build Array (concatenate)(w2719, w2718, w2717, w2716, w2720, w2721) -> (w2711:string[])
              }
              frame #1 {
                n1321 = local read "Offset"() -> (w2739:i32)
                n1322 = local read "REAL1"() -> (w2744:dbl)
                n1323 = local read "REAL2"() -> (w2742:dbl)
                n1324 = local read "Gain"() -> (w2740:dbl)
                n1325 = local read "AD1"() -> (w2743:dbl)
                n1326 = local read "AD2"() -> (w2741:dbl)
                n1327 = Build Array(w2744, w2743, w2742, w2741, w2740, w2739) -> (w2745:dbl[])
                n1328 = for {
                  tunnel: w2745 -> [w2747] mode=indexing
                  tunnel: [w2746] -> w2738 mode=indexing
                  n1329 = Format Into String(format string="%#f" ("格式字符串"), w2747) -> (resulting string=w2746:string)  [unwired: 2 in, 1 out]
                }
              }
              frame #2 {
                n1330 = local read "Offset"() -> (w2749:i32)
                n1331 = local read "REAL1"() -> (w2754:dbl)
                n1332 = local read "REAL2"() -> (w2752:dbl)
                n1333 = local read "Gain"() -> (w2750:dbl)
                n1334 = local read "AD1"() -> (w2753:dbl)
                n1335 = local read "AD2"() -> (w2751:dbl)
                n1336 = Build Array(w2754, w2753, w2752, w2751, w2750, w2749) -> (w2756:dbl[])
                n1337 = for {
                  tunnel: w2756 -> [w2758] mode=indexing
                  tunnel: [w2757] -> w2755 mode=indexing
                  n1338 = Format Into String(format string="%#f" ("格式字符串"), w2758) -> (resulting string=w2757:string)  [unwired: 2 in, 1 out]
                }
              }
            }
            n1339 = Build Path(base path=w2699, name or relative path=w2701) -> (appended path=w2696:path)
            n1340 = call <vilib>:"Open Config Data.vi"("configuration file path"=w2696) -> ("refnum"=w2695:T13)  [unwired: 8 in, 2 out]
            n1341 = Build Array(w2691, w2690, w2689) -> (w2688:string[][])
            n1342 = for {
              tunnel: w2695 -> [w2764]
              tunnel: string[] ["Current Gain", "SumV in", "SumV Out"] -> [w2763] mode=indexing
              tunnel: string[][] [["Shunt Current Offset", "Shunt Current Gain", "Shunt Volt Offset", "Shunt Volt Gain", "Shunt Type", "REAL1", "AD1", "REAL2", "AD2", "Gain"], ["REAL1", "AD1", "REAL2", "AD2", "Gain", "Offset", "", "", "", ""], ["REAL1", "AD1", "REAL2", "AD2", "Gain", "Offset", "", "", "", ""]] -> [w2762] mode=indexing
              tunnel: [w2761] -> w2692
              tunnel: w2688 -> [w2760] mode=indexing
              n1343 = for {
                tunnel: w2764 -> [w2769]
                tunnel: w2763 -> [w2768]
                tunnel: w2762 -> [w2767] mode=indexing
                tunnel: [w2766] -> w2761
                tunnel: w2760 -> [w2765] mode=indexing
                n1344 = call-poly <vilib>:"Write Key.vi"("section"=w2768, "value"=w2765, "key"=w2767, "refnum"=w2769) -> ("refnum out"=w2766:T13)  [unwired: 5 in, 2 out]
              }
            }
            n1345 = stacked-sequence {
              tunnel: w2692 -> [w2710]
              frame #0 {
                n1346 = call <vilib>:"Close Config Data.vi"("refnum"=w2710) -> ("file path"=w2706:path)  [unwired: 9 in, 1 out]
                n1347 = Path To String(path=w2706) -> (string=w2705:string)
                n1348 = control-ref of="结果"() -> (w2708:refnum<vi>)
                n1349 = Concatenate Strings("记录完成,路径为:" ("字符串"), w2705) -> (w2703:string)
                n1350 = Build Array(w2703) -> (w2709:string[])
                n1351 = call "表格编辑.vi"("新元素/子数组"=w2709, "活动单元格:单元格背景色"=u32 6618880, "MCListbox引用句柄"=w2708) -> ()  [unwired: 9 out]
              }
            }
          }
        }
      }
      event "输出自定义值1 2": Value Change {
        n1352 = event-data() -> ("NewVal"=w2772:bool)  [unwired: 6 out]
        n1353 = case shown="假" w2772 {
          tunnel: w2771 -> [w2776 w2803]
          tunnel: [w2773 w2801] -> w2770
          frame False {
            w2777 = u8 0 ("禁用")
            n1354 = local read "VISA资源名称输出"() -> (w2782:refnum<visa-resource-name>)
            n1355 = local write "控制读取  2"(FALSE ("控制读取")) -> ()
            n1356 = flat-sequence {
              tunnel: [w2785] -> w2783
              tunnel: w2782 -> [w2785]
              tunnel: w2783 -> [w2789]
              tunnel: [w2788] -> w2780
              tunnel: w2776 -> [w2787]
              tunnel: [w2786] -> w2774
              tunnel: w2780 -> [w2793]
              tunnel: [w2793] -> w2779
              tunnel: [w2791] -> w2775
              tunnel: w2774 -> [w2791]
              tunnel: [w2797] -> w2781
              tunnel: w2779 -> [w2798]
              tunnel: w2775 -> [w2795]
              tunnel: [w2794] -> w2773
              frame #0 {
                n1357 = Wait (ms)(milliseconds to wait=u32 200 ("等待时间（毫秒）")) -> ()  [unwired: 1 out]
              }
              frame #1 {
                n1358 = VISA Write(VISA resource name=w2789, write buffer="outp off" ("写入缓冲区"), error in (no error)=w2787) -> (VISA resource name out=w2788:refnum<visa-resource-name>, error out=w2786:errorcluster)  [unwired: 1 out]
              }
              frame #2 {
                n1359 = Wait (ms)(milliseconds to wait=u32 50 ("等待时间（毫秒）")) -> ()  [unwired: 1 out]
              }
              frame #3 {
                n1360 = local write "控制读取  2"(TRUE ("控制读取")) -> ()
                n1361 = VISA Write(VISA resource name=w2798, write buffer="outp off" ("写入缓冲区"), error in (no error)=w2795) -> (VISA resource name out=w2797:refnum<visa-resource-name>, error out=w2794:errorcluster)  [unwired: 1 out]
              }
            }
            n1362 = local write "VISA资源名称输出"(w2781) -> ()
            n1363 = property on="输出100A" class="Bool"("Disabled"=w2777) -> ()  [unwired: 2 in, 2 out]
            n1364 = property on="输出200A" class="Bool"("Disabled"=w2777) -> ()  [unwired: 2 in, 2 out]
            n1365 = property on="输出自定义值2 2" class="Bool"("Disabled"=w2777) -> ()  [unwired: 2 in, 2 out]
            n1366 = property on="输出自定义值1 2" class="Bool"("Disabled"=w2777) -> ()  [unwired: 2 in, 2 out]
          }
          frame True {
            w2806 = u8 2 ("禁用")
            n1367 = property on="输出200A" class="Bool"("Disabled"=w2806) -> ()  [unwired: 2 in, 2 out]
            n1368 = property on="输出100A" class="Bool"("Disabled"=w2806) -> ()  [unwired: 2 in, 2 out]
            n1369 = property on="输出自定义值2 2" class="Bool"("Disabled"=w2806) -> ()  [unwired: 2 in, 2 out]
            n1370 = local read "Curr1"() -> (w2800:dbl)
            n1371 = flat-sequence {
              tunnel: FALSE ("控制读取") -> [w2816]
              tunnel: [w2826] -> w2811
              tunnel: [w2825] -> w2809
              tunnel: [w2819] -> w2804
              tunnel: w2803 -> [w2818]
              tunnel: w2811 -> [w2830]
              tunnel: [w2830] -> w2810
              tunnel: w2809 -> [w2829]
              tunnel: [w2829] -> w2808
              tunnel: [w2827] -> w2805
              tunnel: w2804 -> [w2827]
              tunnel: w2810 -> [w2835]
              tunnel: w2808 -> [w2834]
              tunnel: [w2833] -> w2815
              tunnel: [w2832] -> w2813
              tunnel: w2805 -> [w2831]
              tunnel: w2815 -> [w2838]
              tunnel: [w2838] -> w2814
              tunnel: w2813 -> [w2837]
              tunnel: [w2837] -> w2812
              tunnel: w2814 -> [w2842]
              tunnel: w2812 -> [w2841]
              tunnel: [w2839] -> w2802
              tunnel: w2802 -> [w2845]
              tunnel: [w2845] -> w2801
              frame #0 {
                n1372 = local write "控制读取  2"(w2816) -> ()
              }
              frame #1 {
                n1373 = Wait (ms)(milliseconds to wait=u32 50 ("等待时间（毫秒）")) -> ()  [unwired: 1 out]
              }
              frame #2 {
                n1374 = local read "VISA资源名称输出"() -> (w2824:refnum<visa-resource-name>)
                n1375 = local read "Curr1"() -> (w2822:dbl)
                n1376 = Number To Fractional String(number=w2822, precision (6)=i16 3 ("精度(6)")) -> (F-format string=w2820:string)  [unwired: 2 out]
                n1377 = Concatenate Strings("volt 1;curr " ("写入缓冲区"), w2820) -> (w2819:string)
                n1378 = VISA Write(VISA resource name=w2824, write buffer=w2819, error in (no error)=w2818) -> (VISA resource name out=w2826:refnum<visa-resource-name>, error out=w2825:errorcluster)  [unwired: 1 out]
              }
              frame #3 {
                n1379 = Wait (ms)(milliseconds to wait=u32 50 ("等待时间（毫秒）")) -> ()  [unwired: 1 out]
              }
              frame #4 {
                n1380 = VISA Write(VISA resource name=w2835, write buffer=w2831, error in (no error)=w2834) -> (VISA resource name out=w2833:refnum<visa-resource-name>, error out=w2832:errorcluster)  [unwired: 1 out]
              }
              frame #5 {
                n1381 = Wait (ms)(milliseconds to wait=u32 200 ("等待时间（毫秒）")) -> ()  [unwired: 1 out]
              }
              frame #6 {
                n1382 = Wait (ms)(milliseconds to wait=u32 50 ("等待时间（毫秒）")) -> ()  [unwired: 1 out]
                n1383 = VISA Write(VISA resource name=w2842, write buffer="outp on" ("写入缓冲区"), error in (no error)=w2841) -> (VISA resource name out=w2844:refnum<visa-resource-name>, error out=w2839:errorcluster)  [unwired: 1 out]
                n1384 = local write "VISA资源名称输出"(w2844) -> ()
              }
              frame #7 {
                n1385 = local write "控制读取  2"(TRUE ("控制读取")) -> ()
              }
            }
            n1386 = local write "REAL1"(w2800) -> ()
            n1387 = local write "Set"(w2800) -> ()
          }
        }
      }
      event "输出自定义值2 2": Value Change {
        n1388 = event-data() -> ("NewVal"=w2849:bool)  [unwired: 6 out]
        n1389 = case shown="真" w2849 {
          tunnel: w2848 -> [_ w2873]
          tunnel: [w2850 w2871] -> w2847
          frame False {
            w2851 = u8 0 ("禁用")
            n1390 = local read "VISA资源名称输出"() -> (w2856:refnum<visa-resource-name>)
            n1391 = local write "控制读取  2"(FALSE ("控制读取")) -> ()
            n1392 = flat-sequence {
              tunnel: [w2859] -> w2857
              tunnel: w2856 -> [w2859]
              tunnel: w2857 -> [w2861]
              tunnel: [w2860] -> w2854
              tunnel: w2854 -> [w2864]
              tunnel: [w2864] -> w2853
              tunnel: [w2867] -> w2855
              tunnel: w2853 -> [w2868]
              tunnel: [w2865] -> w2850
              frame #0 {
                n1393 = Wait (ms)(milliseconds to wait=u32 200 ("等待时间（毫秒）")) -> ()  [unwired: 1 out]
              }
              frame #1 {
                n1394 = VISA Write(VISA resource name=w2861, write buffer="outp off" ("写入缓冲区")) -> (VISA resource name out=w2860:refnum<visa-resource-name>)  [unwired: 1 in, 2 out]
              }
              frame #2 {
                n1395 = Wait (ms)(milliseconds to wait=u32 50 ("等待时间（毫秒）")) -> ()  [unwired: 1 out]
              }
              frame #3 {
                n1396 = local write "控制读取  2"(TRUE ("控制读取")) -> ()
                n1397 = VISA Write(VISA resource name=w2868, write buffer="outp off" ("写入缓冲区")) -> (VISA resource name out=w2867:refnum<visa-resource-name>, error out=w2865:errorcluster)  [unwired: 1 in, 1 out]
              }
            }
            n1398 = local write "VISA资源名称输出"(w2855) -> ()
            n1399 = property on="输出100A" class="Bool"("Disabled"=w2851) -> ()  [unwired: 2 in, 2 out]
            n1400 = property on="输出200A" class="Bool"("Disabled"=w2851) -> ()  [unwired: 2 in, 2 out]
            n1401 = property on="输出自定义值2 2" class="Bool"("Disabled"=w2851) -> ()  [unwired: 2 in, 2 out]
            n1402 = property on="输出自定义值1 2" class="Bool"("Disabled"=w2851) -> ()  [unwired: 2 in, 2 out]
          }
          frame True {
            n1403 = local read "Curr2"() -> (w2870:dbl)
            n1404 = flat-sequence {
              tunnel: FALSE ("控制读取") -> [w2885]
              tunnel: [w2895] -> w2880
              tunnel: [w2894] -> w2878
              tunnel: [w2889] -> w2874
              tunnel: w2873 -> [w2887]
              tunnel: w2880 -> [w2899]
              tunnel: [w2899] -> w2879
              tunnel: w2878 -> [w2898]
              tunnel: [w2898] -> w2877
              tunnel: [w2896] -> w2875
              tunnel: w2874 -> [w2896]
              tunnel: w2879 -> [w2904]
              tunnel: w2877 -> [w2903]
              tunnel: [w2902] -> w2884
              tunnel: [w2901] -> w2882
              tunnel: w2875 -> [w2900]
              tunnel: w2884 -> [w2907]
              tunnel: [w2907] -> w2883
              tunnel: w2882 -> [w2906]
              tunnel: [w2906] -> w2881
              tunnel: w2883 -> [w2911]
              tunnel: w2881 -> [w2910]
              tunnel: [w2908] -> w2872
              tunnel: w2872 -> [w2914]
              tunnel: [w2914] -> w2871
              frame #0 {
                n1405 = local write "控制读取  2"(w2885) -> ()
              }
              frame #1 {
                n1406 = Wait (ms)(milliseconds to wait=u32 50 ("等待时间（毫秒）")) -> ()  [unwired: 1 out]
              }
              frame #2 {
                n1407 = local read "VISA资源名称输出"() -> (w2893:refnum<visa-resource-name>)
                n1408 = local read "Curr2"() -> (w2888:dbl)
                n1409 = Number To Fractional String(number=w2888, precision (6)=i16 3 ("精度(6)")) -> (F-format string=w2890:string)  [unwired: 2 out]
                n1410 = Concatenate Strings("volt 1;curr " ("写入缓冲区"), w2890) -> (w2889:string)
                n1411 = VISA Write(VISA resource name=w2893, write buffer=w2889, error in (no error)=w2887) -> (VISA resource name out=w2895:refnum<visa-resource-name>, error out=w2894:errorcluster)  [unwired: 1 out]
              }
              frame #3 {
                n1412 = Wait (ms)(milliseconds to wait=u32 50 ("等待时间（毫秒）")) -> ()  [unwired: 1 out]
              }
              frame #4 {
                n1413 = VISA Write(VISA resource name=w2904, write buffer=w2900, error in (no error)=w2903) -> (VISA resource name out=w2902:refnum<visa-resource-name>, error out=w2901:errorcluster)  [unwired: 1 out]
              }
              frame #5 {
                n1414 = Wait (ms)(milliseconds to wait=u32 200 ("等待时间（毫秒）")) -> ()  [unwired: 1 out]
              }
              frame #6 {
                n1415 = Wait (ms)(milliseconds to wait=u32 50 ("等待时间（毫秒）")) -> ()  [unwired: 1 out]
                n1416 = VISA Write(VISA resource name=w2911, write buffer="outp on" ("写入缓冲区"), error in (no error)=w2910) -> (VISA resource name out=w2913:refnum<visa-resource-name>, error out=w2908:errorcluster)  [unwired: 1 out]
                n1417 = local write "VISA资源名称输出"(w2913) -> ()
              }
              frame #7 {
                n1418 = local write "控制读取  2"(TRUE ("控制读取")) -> ()
              }
            }
            n1419 = local write "REAL2"(w2870) -> ()
            n1420 = local write "Set"(w2870) -> ()
          }
        }
      }
      event Timeout {
        n1421 = event-data() -> ()  [unwired: 4 out]
      }
      event "监控": Value Change {
        n1422 = event-data() -> ("NewVal"=w2917:bool)  [unwired: 6 out]
        n1423 = case shown="真" w2917 {
          tunnel: [FALSE ("监控 2") TRUE ("监控 2")] -> w2916
          frame False {
          }
          frame True {
          }
        }
        n1424 = local write "监控 2"(w2916) -> ()
      }
      event Menu Selection (User) {
        n1425 = event-data() -> ("ItemTag"=w2920:string)  [unwired: 7 out]
        n1426 = call "getpath.vi"() -> ("stripped path"=w2921:path)  [unwired: 11 out]
        n1427 = case shown="\"自定义\"" w2920 {
          tunnel: w2921 -> [_ w2924 w3007 w3090 w3173]
          frame "假", Default {
          }
          frame "300A以下" {
            n1428 = Build Path(base path=w2924, name or relative path="Settings\\300以下分辨率偏移值.xls" ("名称或相对路径")) -> (appended path=w2930:path)
            n1429 = local read "分辨率偏移值 3"() -> (w2925:T4)
            n1430 = call-poly <vilib>:"Read From Spreadsheet File.vi"("file path (dialog if empty)"=w2930) -> ("all rows"=w2927:string[][])  [unwired: 3 in, 7 out]
            n1431 = Delete From Array(array=w2927, length=1 ("长度"), index (row)=0 ("索引")) -> (array with subset deleted=w2926:string[][])  [unwired: 1 in, 1 out]
            n1432 = for {
              tunnel: w2926 -> [w2939] mode=indexing
              shift-right: [w2931] -> w2922
              shift-left: w2925 -> [w2936]
              n1433 = Index Array(array=w2939, index #1=0 ("索引")) -> (element #1=w2937:string, element #2=w2935:string, element #3=w2933:string)  [unwired: 2 in]
              n1434 = Fract/Exp String To Number(string=w2935) -> (number=w2934:dbl)  [unwired: 4 out]
              n1435 = Fract/Exp String To Number(string=w2933) -> (number=w2932:dbl)  [unwired: 4 out]
              n1436 = case shown="\"高压板功率\"" w2937 {
                tunnel: w2936 -> [w2940 w2944 w2948 w2952 w2956 w2960 w2964 w2968 w2972 w2976 w2980 w2984 w2988 w2992 w2996 w3000 w3004]
                tunnel: [w2940 w2943 w2947 w2951 w2955 w2959 w2963 w2967 w2971 w2975 w2979 w2983 w2987 w2991 w2995 w2999 w3003] -> w2931
                tunnel: w2934 -> [_ w2942 w2946 w2950 w2954 w2958 w2962 w2966 w2970 w2974 w2978 w2982 w2986 w2990 w2994 w2998 w3002]
                tunnel: w2932 -> [_ w2941 w2945 w2949 w2953 w2957 w2961 w2965 w2969 w2973 w2977 w2981 w2985 w2989 w2993 w2997 w3001]
                frame "假", Default {
                }
                frame "主板总电压" {
                  n1437 = Bundle By Name(cluster=w2944, "主板总电压分辨率"=w2942, "主板总电压偏移量"=w2941) -> (w2943:T4)
                }
                frame "高压板总电压" {
                  n1438 = Bundle By Name(cluster=w2948, "高压板总电压分辨率"=w2946, "高压板总电压偏移量"=w2945) -> (w2947:T4)
                }
                frame "高压板总电流" {
                  n1439 = Bundle By Name(cluster=w2952, "高压板总电流分辨率"=w2950, "高压板总电流偏移量"=w2949) -> (w2951:T4)
                }
                frame "高压板安时" {
                  n1440 = Bundle By Name(cluster=w2956, "高压板安时分辨率"=w2954, "高压板安时偏移量"=w2953) -> (w2955:T4)
                }
                frame "高压板SOC" {
                  n1441 = Bundle By Name(cluster=w2960, "高压板SOC分辨率"=w2958, "高压板SOC偏移量"=w2957) -> (w2959:T4)
                }
                frame "高压板功率" {
                  n1442 = Bundle By Name(cluster=w2964, "高压板功率分辨率"=w2962, "高压板功率偏移量"=w2961) -> (w2963:T4)
                }
                frame "主板总电流" {
                  n1443 = Bundle By Name(cluster=w2968, "主板总电流分辨率"=w2966, "主板总电流偏移量"=w2965) -> (w2967:T4)
                }
                frame "主板安时" {
                  n1444 = Bundle By Name(cluster=w2972, "主板安时分辨率"=w2970, "主板安时偏移量"=w2969) -> (w2971:T4)
                }
                frame "主板SOC" {
                  n1445 = Bundle By Name(cluster=w2976, "主板SOC分辨率"=w2974, "主板SOC偏移量"=w2973) -> (w2975:T4)
                }
                frame "从板总电压" {
                  n1446 = Bundle By Name(cluster=w2980, "从板总电压分辨率"=w2978, "从板总电压偏移量"=w2977) -> (w2979:T4)
                }
                frame "从板总电流" {
                  n1447 = Bundle By Name(cluster=w2984, "从板总电流分辨率"=w2982, "从板总电流偏移量"=w2981) -> (w2983:T4)
                }
                frame "从板安时" {
                  n1448 = Bundle By Name(cluster=w2988, "从板安时分辨率"=w2986, "从板安时偏移量"=w2985) -> (w2987:T4)
                }
                frame "从板SOC" {
                  n1449 = Bundle By Name(cluster=w2992, "从板SOC分辨率"=w2990, "从板SOC偏移量"=w2989) -> (w2991:T4)
                }
                frame "温度" {
                  n1450 = Bundle By Name(cluster=w2996, "温度分辨率"=w2994, "温度偏移量"=w2993) -> (w2995:T4)
                }
                frame "功率" {
                  n1451 = Bundle By Name(cluster=w3000, "功率分辨率"=w2998, "功率偏移量"=w2997) -> (w2999:T4)
                }
                frame "单体电压" {
                  n1452 = Bundle By Name(cluster=w3004, "单体电压分辨率"=w3002, "单体电压偏移量"=w3001) -> (w3003:T4)
                }
              }
            }
            n1453 = local write "分辨率偏移值 3"(w2922) -> ()
          }
          frame "400A以上" {
            n1454 = Build Path(base path=w3007, name or relative path="Settings\\400以上分辨率偏移值.xls" ("名称或相对路径")) -> (appended path=w3013:path)
            n1455 = local read "分辨率偏移值 3"() -> (w3008:T4)
            n1456 = call-poly <vilib>:"Read From Spreadsheet File.vi"("file path (dialog if empty)"=w3013) -> ("all rows"=w3010:string[][])  [unwired: 3 in, 7 out]
            n1457 = Delete From Array(array=w3010, length=1 ("长度"), index (row)=0 ("索引")) -> (array with subset deleted=w3009:string[][])  [unwired: 1 in, 1 out]
            n1458 = for {
              tunnel: w3009 -> [w3022] mode=indexing
              shift-right: [w3014] -> w3005
              shift-left: w3008 -> [w3019]
              n1459 = Index Array(array=w3022, index #1=0 ("索引")) -> (element #1=w3020:string, element #2=w3018:string, element #3=w3016:string)  [unwired: 2 in]
              n1460 = Fract/Exp String To Number(string=w3018) -> (number=w3017:dbl)  [unwired: 4 out]
              n1461 = Fract/Exp String To Number(string=w3016) -> (number=w3015:dbl)  [unwired: 4 out]
              n1462 = case shown="\"高压板功率\"" w3020 {
                tunnel: w3019 -> [w3023 w3027 w3031 w3035 w3039 w3043 w3047 w3051 w3055 w3059 w3063 w3067 w3071 w3075 w3079 w3083 w3087]
                tunnel: [w3023 w3026 w3030 w3034 w3038 w3042 w3046 w3050 w3054 w3058 w3062 w3066 w3070 w3074 w3078 w3082 w3086] -> w3014
                tunnel: w3017 -> [_ w3025 w3029 w3033 w3037 w3041 w3045 w3049 w3053 w3057 w3061 w3065 w3069 w3073 w3077 w3081 w3085]
                tunnel: w3015 -> [_ w3024 w3028 w3032 w3036 w3040 w3044 w3048 w3052 w3056 w3060 w3064 w3068 w3072 w3076 w3080 w3084]
                frame "假", Default {
                }
                frame "主板总电压" {
                  n1463 = Bundle By Name(cluster=w3027, "主板总电压分辨率"=w3025, "主板总电压偏移量"=w3024) -> (w3026:T4)
                }
                frame "高压板总电压" {
                  n1464 = Bundle By Name(cluster=w3031, "高压板总电压分辨率"=w3029, "高压板总电压偏移量"=w3028) -> (w3030:T4)
                }
                frame "高压板总电流" {
                  n1465 = Bundle By Name(cluster=w3035, "高压板总电流分辨率"=w3033, "高压板总电流偏移量"=w3032) -> (w3034:T4)
                }
                frame "高压板安时" {
                  n1466 = Bundle By Name(cluster=w3039, "高压板安时分辨率"=w3037, "高压板安时偏移量"=w3036) -> (w3038:T4)
                }
                frame "高压板SOC" {
                  n1467 = Bundle By Name(cluster=w3043, "高压板SOC分辨率"=w3041, "高压板SOC偏移量"=w3040) -> (w3042:T4)
                }
                frame "高压板功率" {
                  n1468 = Bundle By Name(cluster=w3047, "高压板功率分辨率"=w3045, "高压板功率偏移量"=w3044) -> (w3046:T4)
                }
                frame "主板总电流" {
                  n1469 = Bundle By Name(cluster=w3051, "主板总电流分辨率"=w3049, "主板总电流偏移量"=w3048) -> (w3050:T4)
                }
                frame "主板安时" {
                  n1470 = Bundle By Name(cluster=w3055, "主板安时分辨率"=w3053, "主板安时偏移量"=w3052) -> (w3054:T4)
                }
                frame "主板SOC" {
                  n1471 = Bundle By Name(cluster=w3059, "主板SOC分辨率"=w3057, "主板SOC偏移量"=w3056) -> (w3058:T4)
                }
                frame "从板总电压" {
                  n1472 = Bundle By Name(cluster=w3063, "从板总电压分辨率"=w3061, "从板总电压偏移量"=w3060) -> (w3062:T4)
                }
                frame "从板总电流" {
                  n1473 = Bundle By Name(cluster=w3067, "从板总电流分辨率"=w3065, "从板总电流偏移量"=w3064) -> (w3066:T4)
                }
                frame "从板安时" {
                  n1474 = Bundle By Name(cluster=w3071, "从板安时分辨率"=w3069, "从板安时偏移量"=w3068) -> (w3070:T4)
                }
                frame "从板SOC" {
                  n1475 = Bundle By Name(cluster=w3075, "从板SOC分辨率"=w3073, "从板SOC偏移量"=w3072) -> (w3074:T4)
                }
                frame "温度" {
                  n1476 = Bundle By Name(cluster=w3079, "温度分辨率"=w3077, "温度偏移量"=w3076) -> (w3078:T4)
                }
                frame "功率" {
                  n1477 = Bundle By Name(cluster=w3083, "功率分辨率"=w3081, "功率偏移量"=w3080) -> (w3082:T4)
                }
                frame "单体电压" {
                  n1478 = Bundle By Name(cluster=w3087, "单体电压分辨率"=w3085, "单体电压偏移量"=w3084) -> (w3086:T4)
                }
              }
            }
            n1479 = local write "分辨率偏移值 3"(w3005) -> ()
          }
          frame "自定义" {
            n1480 = Build Path(base path=w3090, name or relative path="Settings\\分辨率偏移值.xls" ("名称或相对路径")) -> (appended path=w3096:path)
            n1481 = local read "分辨率偏移值 3"() -> (w3091:T4)
            n1482 = call-poly <vilib>:"Read From Spreadsheet File.vi"("file path (dialog if empty)"=w3096) -> ("all rows"=w3093:string[][])  [unwired: 3 in, 7 out]
            n1483 = Delete From Array(array=w3093, length=1 ("长度"), index (row)=0 ("索引")) -> (array with subset deleted=w3092:string[][])  [unwired: 1 in, 1 out]
            n1484 = for {
              tunnel: w3092 -> [w3105] mode=indexing
              shift-right: [w3097] -> w3088
              shift-left: w3091 -> [w3102]
              n1485 = Index Array(array=w3105, index #1=0 ("索引")) -> (element #1=w3103:string, element #2=w3101:string, element #3=w3099:string)  [unwired: 2 in]
              n1486 = Fract/Exp String To Number(string=w3101) -> (number=w3100:dbl)  [unwired: 4 out]
              n1487 = Fract/Exp String To Number(string=w3099) -> (number=w3098:dbl)  [unwired: 4 out]
              n1488 = case shown="\"高压板功率\"" w3103 {
                tunnel: w3102 -> [w3106 w3110 w3114 w3118 w3122 w3126 w3130 w3134 w3138 w3142 w3146 w3150 w3154 w3158 w3162 w3166 w3170]
                tunnel: [w3106 w3109 w3113 w3117 w3121 w3125 w3129 w3133 w3137 w3141 w3145 w3149 w3153 w3157 w3161 w3165 w3169] -> w3097
                tunnel: w3100 -> [_ w3108 w3112 w3116 w3120 w3124 w3128 w3132 w3136 w3140 w3144 w3148 w3152 w3156 w3160 w3164 w3168]
                tunnel: w3098 -> [_ w3107 w3111 w3115 w3119 w3123 w3127 w3131 w3135 w3139 w3143 w3147 w3151 w3155 w3159 w3163 w3167]
                frame "假", Default {
                }
                frame "主板总电压" {
                  n1489 = Bundle By Name(cluster=w3110, "主板总电压分辨率"=w3108, "主板总电压偏移量"=w3107) -> (w3109:T4)
                }
                frame "高压板总电压" {
                  n1490 = Bundle By Name(cluster=w3114, "高压板总电压分辨率"=w3112, "高压板总电压偏移量"=w3111) -> (w3113:T4)
                }
                frame "高压板总电流" {
                  n1491 = Bundle By Name(cluster=w3118, "高压板总电流分辨率"=w3116, "高压板总电流偏移量"=w3115) -> (w3117:T4)
                }
                frame "高压板安时" {
                  n1492 = Bundle By Name(cluster=w3122, "高压板安时分辨率"=w3120, "高压板安时偏移量"=w3119) -> (w3121:T4)
                }
                frame "高压板SOC" {
                  n1493 = Bundle By Name(cluster=w3126, "高压板SOC分辨率"=w3124, "高压板SOC偏移量"=w3123) -> (w3125:T4)
                }
                frame "高压板功率" {
                  n1494 = Bundle By Name(cluster=w3130, "高压板功率分辨率"=w3128, "高压板功率偏移量"=w3127) -> (w3129:T4)
                }
                frame "主板总电流" {
                  n1495 = Bundle By Name(cluster=w3134, "主板总电流分辨率"=w3132, "主板总电流偏移量"=w3131) -> (w3133:T4)
                }
                frame "主板安时" {
                  n1496 = Bundle By Name(cluster=w3138, "主板安时分辨率"=w3136, "主板安时偏移量"=w3135) -> (w3137:T4)
                }
                frame "主板SOC" {
                  n1497 = Bundle By Name(cluster=w3142, "主板SOC分辨率"=w3140, "主板SOC偏移量"=w3139) -> (w3141:T4)
                }
                frame "从板总电压" {
                  n1498 = Bundle By Name(cluster=w3146, "从板总电压分辨率"=w3144, "从板总电压偏移量"=w3143) -> (w3145:T4)
                }
                frame "从板总电流" {
                  n1499 = Bundle By Name(cluster=w3150, "从板总电流分辨率"=w3148, "从板总电流偏移量"=w3147) -> (w3149:T4)
                }
                frame "从板安时" {
                  n1500 = Bundle By Name(cluster=w3154, "从板安时分辨率"=w3152, "从板安时偏移量"=w3151) -> (w3153:T4)
                }
                frame "从板SOC" {
                  n1501 = Bundle By Name(cluster=w3158, "从板SOC分辨率"=w3156, "从板SOC偏移量"=w3155) -> (w3157:T4)
                }
                frame "温度" {
                  n1502 = Bundle By Name(cluster=w3162, "温度分辨率"=w3160, "温度偏移量"=w3159) -> (w3161:T4)
                }
                frame "功率" {
                  n1503 = Bundle By Name(cluster=w3166, "功率分辨率"=w3164, "功率偏移量"=w3163) -> (w3165:T4)
                }
                frame "单体电压" {
                  n1504 = Bundle By Name(cluster=w3170, "单体电压分辨率"=w3168, "单体电压偏移量"=w3167) -> (w3169:T4)
                }
              }
            }
            n1505 = local write "分辨率偏移值 3"(w3088) -> ()
          }
          frame "自定义分辨率" {
            n1506 = Build Path(base path=w3173, name or relative path="SubVi\\分辨率自定义.vi" ("名称或相对路径")) -> (appended path=w3171:path)
            n1507 = Open VI Reference(vi path=w3171) -> (vi reference=w3180:refnum<vi>)  [unwired: 1 in, 5 out]
            n1508 = invoke class="VI" method="FP.Open"(reference=w3180, "Activate"=TRUE ("激活？"), "State"=T12."Standard" ("状态")) -> (reference out=w3177:refnum<vi>, error out=w3176:errorcluster)  [unwired: 2 in, 3 out]
            n1509 = invoke class="VI" method="Run VI"(reference=w3177, error in=w3176, "Wait until done"=FALSE ("结束前等待"), "Auto Dispose Ref"=TRUE ("自动销毁引用")) -> ()  [unwired: 1 in, 5 out]
          }
        }
      }
      event "Read1": Value Change {
        n1510 = event-data() -> ("NewVal"=w3185:bool)  [unwired: 6 out]
        n1511 = case shown="真" w3185 {
          tunnel: w3184 -> [w3187 w3204]
          tunnel: w3183 -> [w3186 w3203]
          tunnel: [w3186 w3202] -> w3182
          tunnel: [w3187 w3201] -> w3181
          frame False {
          }
          frame True {
            n1512 = flat-sequence {
              tunnel: w3203 -> [w3205]
              tunnel: w3204 -> [w3206]
              tunnel: [w3206] -> w3194
              tunnel: [w3205] -> w3192
              tunnel: w3194 -> [w3208]
              tunnel: [w3208] -> w3193
              tunnel: w3192 -> [w3207]
              tunnel: [w3207] -> w3191
              tunnel: w3193 -> [w3210]
              tunnel: [w3210] -> w3198
              tunnel: w3191 -> [w3209]
              tunnel: [w3209] -> w3196
              tunnel: w3198 -> [w3212]
              tunnel: [w3212] -> w3197
              tunnel: w3196 -> [w3211]
              tunnel: [w3211] -> w3195
              tunnel: [w3217] -> w3202
              tunnel: [w3216] -> w3201
              tunnel: w3197 -> [w3219]
              tunnel: w3195 -> [w3218]
              frame #0 {
              }
              frame #1 {
              }
              frame #2 {
              }
              frame #3 {
                n1513 = disable-structure shown="禁用" {
                  frame Disabled {
                    n1514 = local read "自动控制仪器"() -> (w3213:bool)
                    n1515 = case shown="真" w3213 {
                      frame False {
                      }
                      frame True {
                        n1516 = Wait (ms)(milliseconds to wait=u32 2000 ("等待时间（毫秒）")) -> ()  [unwired: 1 out]
                      }
                    }
                  }
                  frame Enabled {
                  }
                }
              }
              frame #4 {
                n1517 = Enqueue Element(queue=w3219, element="Read1" ("元素"), error in (no error)=w3218) -> (queue out=w3216:refnum<queue>, error out=w3217:errorcluster)  [unwired: 2 out]
              }
            }
            n1518 = global write "EV05全局变量1.vi" "CAN接收"(FALSE ("CAN接收")) -> ()
            n1519 = global write "EV05全局变量1.vi" "高压校正接收"(FALSE ("高压校正接收")) -> ()
            n1520 = call <vilib>:"Set Busy.vi"() -> ()  [unwired: 4 in, 8 out]
            n1521 = local write "AD1"(u16 0 ("AD1")) -> ()
            n1522 = property on="Read1结果" class="Bool (严格)"("Colors [4]"=cluster{u32, u32}[] [{0, 0}] ("颜色[4]"), "BoolText.Text"="" ("布尔文本.文本")) -> ()  [unwired: 2 in, 2 out]
          }
        }
      }
      event "Read1_Out": Value Change {
        n1523 = event-data() -> ("NewVal"=w3224:bool)  [unwired: 6 out]
        n1524 = case shown="真" w3224 {
          tunnel: w3223 -> [w3226 w3243]
          tunnel: w3222 -> [w3225 w3242]
          tunnel: [w3225 w3241] -> w3221
          tunnel: [w3226 w3240] -> w3220
          frame False {
          }
          frame True {
            n1525 = flat-sequence {
              tunnel: w3242 -> [w3244]
              tunnel: w3243 -> [w3245]
              tunnel: [w3245] -> w3233
              tunnel: [w3244] -> w3231
              tunnel: w3233 -> [w3247]
              tunnel: [w3247] -> w3232
              tunnel: w3231 -> [w3246]
              tunnel: [w3246] -> w3230
              tunnel: w3232 -> [w3249]
              tunnel: [w3249] -> w3237
              tunnel: w3230 -> [w3248]
              tunnel: [w3248] -> w3235
              tunnel: w3237 -> [w3251]
              tunnel: [w3251] -> w3236
              tunnel: w3235 -> [w3250]
              tunnel: [w3250] -> w3234
              tunnel: [w3254] -> w3241
              tunnel: [w3253] -> w3240
              tunnel: w3236 -> [w3256]
              tunnel: w3234 -> [w3255]
              frame #0 {
              }
              frame #1 {
              }
              frame #2 {
              }
              frame #3 {
              }
              frame #4 {
                n1526 = Enqueue Element(queue=w3256, element="Read1_out" ("元素"), error in (no error)=w3255) -> (queue out=w3253:refnum<queue>, error out=w3254:errorcluster)  [unwired: 2 out]
              }
            }
            n1527 = global write "EV05全局变量1.vi" "CAN接收"(FALSE ("CAN接收")) -> ()
            n1528 = global write "EV05全局变量1.vi" "高压校正接收"(FALSE ("高压校正接收")) -> ()
            n1529 = call <vilib>:"Set Busy.vi"() -> ()  [unwired: 4 in, 8 out]
            n1530 = property on="Read1_Out结果" class="Bool (严格)"("Colors [4]"=cluster{u32, u32}[] [{0, 0}] ("颜色[4]"), "BoolText.Text"="" ("布尔文本.文本")) -> ()  [unwired: 2 in, 2 out]
            n1531 = local write "AD1"(0.0 ("AD1 3")) -> ()
          }
        }
      }
      event "Read2_Out": Value Change {
        n1532 = event-data() -> ("NewVal"=w3261:bool)  [unwired: 6 out]
        n1533 = case shown="真" w3261 {
          tunnel: w3260 -> [w3263 w3279]
          tunnel: w3259 -> [w3262 w3278]
          tunnel: [w3262 w3277] -> w3258
          tunnel: [w3263 w3276] -> w3257
          frame False {
          }
          frame True {
            n1534 = flat-sequence {
              tunnel: w3278 -> [w3280]
              tunnel: w3279 -> [w3281]
              tunnel: [w3281] -> w3269
              tunnel: [w3280] -> w3267
              tunnel: w3269 -> [w3283]
              tunnel: [w3283] -> w3268
              tunnel: w3267 -> [w3282]
              tunnel: [w3282] -> w3266
              tunnel: w3268 -> [w3285]
              tunnel: [w3285] -> w3273
              tunnel: w3266 -> [w3284]
              tunnel: [w3284] -> w3271
              tunnel: w3273 -> [w3287]
              tunnel: [w3287] -> w3272
              tunnel: w3271 -> [w3286]
              tunnel: [w3286] -> w3270
              tunnel: [w3290] -> w3277
              tunnel: [w3289] -> w3276
              tunnel: w3272 -> [w3292]
              tunnel: w3270 -> [w3291]
              frame #0 {
              }
              frame #1 {
              }
              frame #2 {
              }
              frame #3 {
              }
              frame #4 {
                n1535 = Enqueue Element(queue=w3292, element="Read2_out" ("元素"), error in (no error)=w3291) -> (queue out=w3289:refnum<queue>, error out=w3290:errorcluster)  [unwired: 2 out]
              }
            }
            n1536 = global write "EV05全局变量1.vi" "高压校正接收"(FALSE ("高压校正接收")) -> ()
            n1537 = global write "EV05全局变量1.vi" "CAN接收"(FALSE ("CAN接收")) -> ()
            n1538 = call <vilib>:"Set Busy.vi"() -> ()  [unwired: 4 in, 8 out]
            n1539 = property on="Read2_Out结果" class="Bool (严格)"("Colors [4]"=cluster{u32, u32}[] [{0, 0}] ("颜色[4]"), "BoolText.Text"="" ("布尔文本.文本")) -> ()  [unwired: 2 in, 2 out]
          }
        }
      }
      event "Clear": Value Change {
        n1540 = event-data() -> ("NewVal"=w3297:bool)  [unwired: 6 out]
        n1541 = case shown="真" w3297 {
          tunnel: w3296 -> [w3299 w3307]
          tunnel: w3295 -> [w3298 w3306]
          tunnel: [w3298 w3305] -> w3294
          tunnel: [w3299 w3304] -> w3293
          frame False {
          }
          frame True {
            n1542 = flat-sequence {
              tunnel: w3306 -> [w3308]
              tunnel: w3307 -> [w3309]
              tunnel: [w3309] -> w3303
              tunnel: [w3308] -> w3302
              tunnel: [w3312] -> w3305
              tunnel: [w3311] -> w3304
              tunnel: w3303 -> [w3314]
              tunnel: w3302 -> [w3313]
              frame #0 {
              }
              frame #1 {
                n1543 = Enqueue Element(queue=w3314, element="Clear" ("元素"), error in (no error)=w3313) -> (queue out=w3311:refnum<queue>, error out=w3312:errorcluster)  [unwired: 2 out]
              }
            }
            n1544 = property on="Clear结果" class="Bool (严格)"("Colors [4]"=cluster{u32, u32}[] [{0, 0}] ("颜色[4]"), "BoolText.Text"="" ("布尔文本.文本")) -> ()  [unwired: 2 in, 2 out]
          }
        }
      }
      event "写配置文件版本": Value Change {
        n1545 = event-data() -> ("NewVal"=w3319:bool)  [unwired: 6 out]
        n1546 = case shown="真" w3319 {
          tunnel: w3318 -> [w3321 w3329]
          tunnel: w3317 -> [w3320 w3328]
          tunnel: [w3320 w3327] -> w3316
          tunnel: [w3321 w3326] -> w3315
          frame False {
          }
          frame True {
            n1547 = flat-sequence {
              tunnel: w3328 -> [w3330]
              tunnel: w3329 -> [w3331]
              tunnel: [w3331] -> w3325
              tunnel: [w3330] -> w3324
              tunnel: [w3334] -> w3327
              tunnel: [w3333] -> w3326
              tunnel: w3325 -> [w3336]
              tunnel: w3324 -> [w3335]
              frame #0 {
              }
              frame #1 {
                n1548 = Enqueue Element(queue=w3336, element="写配置文件版本" ("元素"), error in (no error)=w3335) -> (queue out=w3333:refnum<queue>, error out=w3334:errorcluster)  [unwired: 2 out]
              }
            }
            n1549 = property on="写版本结果" class="Bool (严格)"("Colors [4]"=cluster{u32, u32}[] [{0, 0}] ("颜色[4]"), "BoolText.Text"="" ("布尔文本.文本")) -> ()  [unwired: 2 in, 2 out]
          }
        }
      }
      event "读配置文件版本": Value Change {
        n1550 = event-data() -> ("NewVal"=w3341:bool)  [unwired: 6 out]
        n1551 = case shown="真" w3341 {
          tunnel: w3340 -> [w3343 w3352]
          tunnel: w3339 -> [w3342 w3351]
          tunnel: [w3342 w3350] -> w3338
          tunnel: [w3343 w3349] -> w3337
          frame False {
          }
          frame True {
            n1552 = flat-sequence {
              tunnel: w3351 -> [w3353]
              tunnel: w3352 -> [w3354]
              tunnel: [w3354] -> w3348
              tunnel: [w3353] -> w3347
              tunnel: [w3357] -> w3350
              tunnel: [w3356] -> w3349
              tunnel: w3348 -> [w3359]
              tunnel: w3347 -> [w3358]
              frame #0 {
              }
              frame #1 {
                n1553 = Enqueue Element(queue=w3359, element="读配置文件版本" ("元素"), error in (no error)=w3358) -> (queue out=w3356:refnum<queue>, error out=w3357:errorcluster)  [unwired: 2 out]
              }
            }
            n1554 = local write "版本号-读"("\u0000\u0000\u0000\u0000\u0000\u0000\u0000\u0000" ("版本号-读")) -> ()
            n1555 = property on="读版本结果" class="Bool (严格)"("Colors [4]"=cluster{u32, u32}[] [{0, 0}] ("颜色[4]"), "BoolText.Text"="" ("布尔文本.文本")) -> ()  [unwired: 2 in, 2 out]
          }
        }
      }
      event "设置参数": Value Change {
        n1556 = event-data() -> ("NewVal"=w3364:bool)  [unwired: 6 out]
        n1557 = case shown="真" w3364 {
          tunnel: w3363 -> [w3366 w3446]
          tunnel: w3362 -> [w3365 w3445]
          tunnel: [w3365 w3444] -> w3361
          tunnel: [w3366 w3443] -> w3360
          frame False {
          }
          frame True {
            w3438 = u16 1 ("y")
            n1558 = flat-sequence {
              tunnel: w3445 -> [w3447]
              tunnel: w3446 -> [w3448]
              tunnel: [w3448] -> w3442
              tunnel: [w3447] -> w3441
              tunnel: [w3451] -> w3444
              tunnel: [w3450] -> w3443
              tunnel: w3442 -> [w3453]
              tunnel: w3441 -> [w3452]
              frame #0 {
              }
              frame #1 {
                n1559 = Enqueue Element(queue=w3453, element="设置参数" ("元素"), error in (no error)=w3452) -> (queue out=w3450:refnum<queue>, error out=w3451:errorcluster)  [unwired: 2 out]
              }
            }
            n1560 = Add(x="传感器类型", y=u16 1) -> (x+y=w3424:u16)
            n1561 = Add(x="分流器大小/A", y=u16 1) -> (x+y=w3425:u16)
            n1562 = Add(x=w3438, y="电压分辨率/V") -> (x+y=w3435:u16)
            n1563 = Add(x=w3438, y="安时分辨率/AH") -> (x+y=w3434:u16)
            n1564 = Add(x="电流分辨率/A", y=w3438) -> (x+y=w3374:u16)
            n1565 = Multiply(x=u16 16, y=w3425) -> (x*y=w3423:u16)
            n1566 = Add(x=w3424, y=w3423) -> (x+y=w3421:u16)
            n1567 = Multiply(x=u16 16, y=w3434) -> (x*y=w3432:u16)
            n1568 = Multiply(x=u16 4, y=w3435) -> (x*y=w3433:u16)
            n1569 = Number To Hexadecimal String(1:i16 2 ("宽度(-)"), 2:w3421) -> (0:w3394:string)
            n1570 = property on="连接状态 10" class="Bool (严格)"("Colors [4]"=cluster{u32, u32}[] [{0, 0}] ("颜色[4]"), "BoolText.Text"="" ("布尔文本.文本")) -> ()  [unwired: 2 in, 2 out]
            n1571 = Compound Arithmetic op=ADD(w3374, w3433, w3432) -> (w3430:u16)
            n1572 = Number To Hexadecimal String(1:i16 2 ("宽度(-)"), 2:w3430) -> (0:w3395:string)
            n1573 = Equal?(x="分流器大小/A", y=u16 0) -> (x = y?=w3412:bool)
            n1574 = Multiply(x=u16 100, y="分流器大小/A") -> (x*y=w3408:u16)
            n1575 = Equal?(x="安时分辨率/AH", y=u16 0) -> (x = y?=w3379:bool)
            n1576 = Equal?(x="是否有外部高压", y=u16 0) -> (x = y?=w3418:bool)
            n1577 = Select(t=u16 50 ("y"), s=w3412, f=w3408) -> (s? t:f=w3402:u16)
            n1578 = Select(t=u16 5 ("y"), s=w3418, f=u16 0 ("y")) -> (s? t:f=w3416:u16)
            n1579 = Select(t=u16 375 ("y"), s=w3379, f=u32 75006 ("y")) -> (s? t:f=w3401:u32)
            n1580 = Number To Hexadecimal String(1:i16 2 ("宽度(-)"), 2:w3416) -> (0:w3393:string)
            n1581 = Multiply(x=u16 300 ("y"), y=w3401) -> (x*y=w3399:u32)
            n1582 = Divide(x=w3399, y=w3402) -> (x/y=w3398:dbl)
            n1583 = Round To Nearest(number=w3398) -> (nearest integer value=w3397:dbl)
            "充放电阈值" <- w3397
            n1584 = Number To Hexadecimal String(1:i16 8 ("宽度(-)"), 2:w3397) -> (0:w3396:string)
            n1585 = Number To Hexadecimal String(1:i16 2 ("宽度(-)"), 2:0 ("数字")) -> (0:w3389:string)
            n1586 = Concatenate Strings(w3396, w3389, w3395, w3394, w3393) -> (→"config_data":string)
            n1587 = Equal?(x="电流分辨率/A", y=u16 0) -> (x = y?=w3369:bool)
            n1588 = Equal?(x="电压分辨率/V", y=u16 0) -> (x = y?=w3386:bool)
            n1589 = Select(t=sgl 0.01 ("y"), s=w3386, f=sgl 0.1 ("y")) -> (s? t:f=w3383:sgl)
            n1590 = Select(t=sgl 0.01 ("y"), s=w3369, f=sgl 0.1 ("y")) -> (s? t:f=w3373:sgl)
            n1591 = Select(t=sgl -300.0 ("y"), s=w3369, f=sgl -3000.0 ("y")) -> (s? t:f=w3368:sgl)
            n1592 = Select(t=sgl 0.001 ("y"), s=w3379, f=sgl 0.2 ("y")) -> (s? t:f=w3378:sgl)
            n1593 = local read "分辨率偏移值 3"() -> (w3388:T4)
            n1594 = Bundle By Name(cluster=w3388, "高压板总电压分辨率"=w3383, "高压板总电流分辨率"=w3373, "高压板总电流偏移量"=w3368, "高压板安时分辨率"=w3378) -> (w3372:T4)
            n1595 = local write "分辨率偏移值 3"(w3372) -> ()
          }
        }
      }
      event "生成配置": Value Change {
        n1596 = event-data() -> ("NewVal"=w3455:bool)  [unwired: 6 out]
        n1597 = case shown="真" w3455 {
          tunnel: w3454 -> [_ w3457]
          frame False {
          }
          frame True {
            n1598 = call "文件对话框"("error in"=w3457, "pattern (all files)"=".txt") -> ("selected path"=w3458:path, "cancelled"=w3459:bool, "error out"=w3456:errorcluster)  [unwired: 5 in, 6 out]
            n1599 = case shown="假" w3459 {
              tunnel: w3458 -> [w3464 _]
              tunnel: w3456 -> [_ _]
              frame False {
                n1600 = local read "安时分辨率/AH"() -> (w3499:u16)
                n1601 = local read "是否有外部高压"() -> (w3481:u16)
                n1602 = local read "电流分辨率/A"() -> (w3512:u16)
                n1603 = local read "电压分辨率/V"() -> (w3504:u16)
                n1604 = local read "传感器类型"() -> (w3494:u16)
                n1605 = local read "分流器大小/A"() -> (w3492:u16)
                n1606 = Equal To 0?(x=w3512) -> (x = 0?=w3511:bool)
                n1607 = Equal To 0?(x=w3504) -> (x = 0?=w3505:bool)
                n1608 = Equal To 0?(x=w3499) -> (x = 0?=w3502:bool)
                n1609 = local read "充放电阈值"() -> (w3479:dbl)
                n1610 = Equal To 0?(x=w3494) -> (x = 0?=w3495:bool)
                n1611 = Equal?(x=w3492, y=u16 0) -> (x = y?=w3490:bool)
                n1612 = Select(t="0.01", s=w3511, f="0.1") -> (s? t:f=w3508:string)
                n1613 = Select(t="0.01", s=w3505, f="0.1") -> (s? t:f=w3503:string)
                n1614 = Multiply(x=u16 100, y=w3492) -> (x*y=w3487:u16)
                n1615 = Select(t="0.001", s=w3502, f="0.2") -> (s? t:f=w3498:string)
                n1616 = Select(t="霍尔传感器", s=w3495, f="分流器") -> (s? t:f=w3493:string)
                n1617 = Equal To 0?(x=w3481) -> (x = 0?=w3484:bool)
                n1618 = Select(t=u16 50 ("y"), s=w3490, f=w3487) -> (s? t:f=w3486:u16)
                n1619 = Select(t="有", s=w3484, f="无") -> (s? t:f=w3480:string)
                n1620 = Number To Decimal String(number=w3486) -> (decimal integer string=w3485:string)  [unwired: 1 out]
                n1621 = Number To Decimal String(number=w3479) -> (decimal integer string=w3478:string)  [unwired: 1 out]
                n1622 = local read "版本号"() -> (w3473:string)
                n1623 = Build Array("参数值" ("元素"), w3508, w3503, w3498, w3493, w3485, w3480, w3478, w3473) -> (w3476:string[])
                n1624 = Build Array(string[] ["参数名称", "电流分辨率", "电压分辨率", "安时分辨率", "传感器类型", "分流器大小", "是否有外部高压", "充放电阈值", "配置文件版本号"], w3476) -> (w3474:string[][])
                n1625 = Transpose 2D Array(2D array=w3474) -> (transposed array=w3465:string[][])
                n1626 = call-poly <vilib>:"Write To Spreadsheet File.vi"("2D data"=w3465, "file path (dialog if empty)"=w3464) -> ("new file path (Not A Path if cancelled)"=w3461:path)  [unwired: 4 in, 2 out]
                n1627 = call <vilib>:"MD5Checksum File.vi"("Path"=w3461) -> ("MD5 message-digest"=w3471:string)  [unwired: 1 in, 9 out]
                n1628 = Strip Path(path=w3461) -> (stripped path=w3462:path)  [unwired: 1 out]
                n1629 = call <vilib>:"Get File Extension.vi"("file"=w3461) -> ("filename without extension"=w3469:string)  [unwired: 1 in, 9 out]
                n1630 = Concatenate Strings(w3469, "_(MD5=" ("字符串"), w3471, ")" ("字符串"), ".txt" ("字符串")) -> (w3467:string)
                n1631 = Build Path(base path=w3462, name or relative path=w3467) -> (appended path=w3466:path)
                n1632 = call-poly <vilib>:"Write To Spreadsheet File.vi"("2D data"=w3465, "file path (dialog if empty)"=w3466) -> ("new file path (Not A Path if cancelled)"=w3463:path)  [unwired: 4 in, 2 out]
                n1633 = flat-sequence {
                  tunnel: w3463 -> [_]
                  tunnel: w3461 -> [w3513]
                  frame #0 {
                    n1634 = Delete(path (use dialog)=w3513) -> ()  [unwired: 1 in, 6 out]
                  }
                }
              }
              frame True {
              }
            }
          }
        }
      }
      event "导入配置": Value Change {
        n1635 = event-data() -> ("NewVal"=w3515:bool)  [unwired: 6 out]
        n1636 = case shown="真" w3515 {
          tunnel: w3514 -> [_ w3517]
          frame False {
          }
          frame True {
            n1637 = property on="导入配置结果" class="Bool (严格)"("Colors [4]"=cluster{u32, u32}[] [{0, 0}] ("颜色[4]"), "BoolText.Text"="" ("布尔文本.文本")) -> ()  [unwired: 2 in, 2 out]
            n1638 = call "文件对话框2"("default name"=".txt", "error in"=w3517) -> ("selected path"=w3520:path, "cancelled"=w3521:bool, "error out"=w3516:errorcluster)  [unwired: 5 in, 6 out]
            n1639 = case shown="假" w3521 {
              tunnel: w3520 -> [w3537 _]
              tunnel: w3516 -> [_ _]
              frame False {
                n1640 = call-poly <vilib>:"Read From Spreadsheet File.vi"("file path (dialog if empty)"=w3537) -> ("all rows"=w3540:string[][])  [unwired: 3 in, 7 out]
                n1641 = call <vilib>:"Get File Extension.vi"("file"=w3537) -> ("filename without extension"=w3534:string)  [unwired: 1 in, 9 out]
                n1642 = call <vilib>:"MD5Checksum File.vi"("Path"=w3537) -> ("MD5 message-digest"=w3528:string)  [unwired: 1 in, 9 out]
                n1643 = Index Array(array=w3540, index (col)=0 ("禁用的索引 (列)")) -> (element=w3543:string[])  [unwired: 1 in]
                n1644 = Index Array(array=w3540, index (col)=1 ("禁用的索引 (列)")) -> (element=w3539:string[])  [unwired: 1 in]
                n1645 = Match Pattern(string=w3534, regular expression="(MD5=" ("正则表达式")) -> (offset past match=w3532:i32)  [unwired: 4 out]
                n1646 = Match Pattern(string=w3534, regular expression=")" ("正则表达式")) -> (offset past match=w3533:i32)  [unwired: 4 out]
                n1647 = Subtract(x=w3533, y=w3532) -> (x-y=w3531:i32)
                n1648 = Decrement(x=w3531) -> (x-1=w3530:i32)
                n1649 = String Subset(string=w3534, offset (0)=w3532, length (rest)=w3530) -> (substring=w3529:string)
                n1650 = for {
                  N: 9 -> [_]
                  tunnel: w3543 -> [w3549] mode=indexing
                  tunnel: w3539 -> [w3548] mode=indexing
                  n1651 = case shown="\"配置文件版本号\"" w3549 {
                    tunnel: w3548 -> [_ w3555 w3557 w3563 w3569 w3575 w3581 w3582 w3584]
                    frame "假", Default {
                    }
                    frame "电流分辨率" {
                      n1652 = Equal?(x=w3555, y="0.01") -> (x = y?=w3553:bool)
                      n1653 = Select(t=0.0, s=w3553, f=1.0) -> (s? t:f=w3552:dbl)
                      n1654 = local write "电流分辨率/A"(w3552) -> ()
                    }
                    frame "电压分辨率" {
                      n1655 = Equal?(x=w3557, y="0.01") -> (x = y?=w3560:bool)
                      n1656 = Select(t=0.0, s=w3560, f=1.0) -> (s? t:f=w3556:dbl)
                      n1657 = local write "电压分辨率/V"(w3556) -> ()
                    }
                    frame "安时分辨率" {
                      n1658 = Equal?(x=w3563, y="0.001") -> (x = y?=w3566:bool)
                      n1659 = Select(t=0.0, s=w3566, f=1.0) -> (s? t:f=w3562:dbl)
                      n1660 = local write "安时分辨率/AH"(w3562) -> ()
                    }
                    frame "传感器类型" {
                      n1661 = Equal?(x=w3569, y="霍尔传感器") -> (x = y?=w3572:bool)
                      n1662 = Select(t=0.0, s=w3572, f=1.0) -> (s? t:f=w3568:dbl)
                      n1663 = local write "传感器类型"(w3568) -> ()
                    }
                    frame "是否有外部高压" {
                      n1664 = Equal?(x=w3575, y="有") -> (x = y?=w3578:bool)
                      n1665 = Select(t=0.0, s=w3578, f=1.0) -> (s? t:f=w3574:dbl)
                      n1666 = local write "是否有外部高压"(w3574) -> ()
                    }
                    frame "充放电阈值" {
                      n1667 = Decimal String To Number(string=w3581) -> (number=w3580:i32)  [unwired: 3 out]
                      n1668 = local write "充放电阈值"(w3580) -> ()
                    }
                    frame "配置文件版本号" {
                      n1669 = local write "版本号"(w3582) -> ()
                    }
                    frame "分流器大小" {
                      n1670 = Search 1D Array(1D array=string[] ["50", "100", "200", "300", "400", "500", "600", "700", "800", "900", "1000"], element=w3584) -> (index of element=w3583:i32)  [unwired: 1 out]
                      n1671 = local write "分流器大小/A"(w3583) -> ()
                    }
                  }
                }
                n1672 = Equal?(x=w3528, y=w3529) -> (x = y?=w3525:bool)
                n1673 = case shown="假" w3525 {
                  tunnel: cluster{u32, u32}[] [{6618880, 6618880}] ("颜色[4]") -> [w3544 _]
                  tunnel: cluster{u32, u32}[] [{15663131, 6618880}] ("颜色[4]") -> [_ w3547]
                  tunnel: [w3544 w3547] -> w3524
                  tunnel: ["通过" ("布尔文本.文本") "失败" ("布尔文本.文本")] -> w3523
                  frame True {
                  }
                  frame False {
                  }
                }
                n1674 = property on="导入配置结果" class="Bool (严格)"("Colors [4]"=w3524, "BoolText.Text"=w3523) -> ()  [unwired: 2 in, 2 out]
              }
              frame True {
              }
            }
          }
        }
      }
      event "分流器大小/A": Value Change {
        n1675 = event-data() -> ("NewVal"=w3586:u16)  [unwired: 6 out]
        n1676 = local read "安时分辨率/AH"() -> (w3601:u16)
        n1677 = Equal?(x=w3586, y=u16 0) -> (x = y?=w3599:bool)
        n1678 = Multiply(x=u16 100, y=w3586) -> (x*y=w3596:u16)
        n1679 = Select(t=u16 50 ("y"), s=w3599, f=w3596) -> (s? t:f=w3591:u16)
        n1680 = Equal?(x=w3601, y=u16 0) -> (x = y?=w3594:bool)
        n1681 = Select(t=u16 375 ("y"), s=w3594, f=u32 75006 ("y")) -> (s? t:f=w3590:u32)
        n1682 = Multiply(x=u16 300 ("y"), y=w3590) -> (x*y=w3588:u32)
        n1683 = Divide(x=w3588, y=w3591) -> (x/y=w3587:dbl)
        n1684 = Round To Nearest(number=w3587) -> (nearest integer value=w3602:dbl)
        n1685 = local write "充放电阈值"(w3602) -> ()
      }
      event "安时分辨率/AH": Value Change {
        n1686 = event-data() -> ("NewVal"=w3603:u16)  [unwired: 6 out]
        n1687 = local read "分流器大小/A"() -> (w3619:u16)
        n1688 = Equal?(x=w3619, y=u16 0) -> (x = y?=w3616:bool)
        n1689 = Multiply(x=u16 100, y=w3619) -> (x*y=w3613:u16)
        n1690 = Select(t=u16 50 ("y"), s=w3616, f=w3613) -> (s? t:f=w3608:u16)
        n1691 = Equal?(x=w3603, y=u16 0) -> (x = y?=w3611:bool)
        n1692 = Select(t=u16 375 ("y"), s=w3611, f=u32 75006 ("y")) -> (s? t:f=w3607:u32)
        n1693 = Multiply(x=u16 300 ("y"), y=w3607) -> (x*y=w3605:u32)
        n1694 = Divide(x=w3605, y=w3608) -> (x/y=w3604:dbl)
        n1695 = Round To Nearest(number=w3604) -> (nearest integer value=w3618:dbl)
        n1696 = local write "充放电阈值"(w3618) -> ()
      }
      event "Set Current Offset": Value Change {
        n1697 = event-data() -> ("NewVal"=w3624:bool)  [unwired: 6 out]
        n1698 = case shown="真" w3624 {
          tunnel: w3623 -> [w3626 w3636]
          tunnel: w3622 -> [w3625 w3635]
          tunnel: [w3625 w3634] -> w3621
          tunnel: [w3626 w3633] -> w3620
          frame False {
          }
          frame True {
            n1699 = Enqueue Element(queue=w3636, element="Set Current Offset" ("元素"), error in (no error)=w3635) -> (queue out=w3633:refnum<queue>, error out=w3634:errorcluster)  [unwired: 2 out]
            n1700 = global write "EV05全局变量1.vi" "高压校正接收"(FALSE ("高压校正接收")) -> ()
            n1701 = global write "EV05全局变量1.vi" "CAN接收"(FALSE ("CAN接收")) -> ()
            n1702 = call <vilib>:"Set Busy.vi"() -> ()  [unwired: 4 in, 8 out]
            n1703 = property on="Current Offset结果" class="Bool (严格)"("Colors [4]"=cluster{u32, u32}[] [{0, 0}] ("颜色[4]"), "BoolText.Text"="" ("布尔文本.文本")) -> ()  [unwired: 2 in, 2 out]
            n1704 = local write "电流零点"("" ("5460Current Offset")) -> ()
          }
        }
      }
      event "Set Current Offset 3": Value Change {
        n1705 = event-data() -> ("NewVal"=w3641:bool)  [unwired: 6 out]
        n1706 = case shown="真" w3641 {
          tunnel: w3640 -> [w3643 w3653]
          tunnel: w3639 -> [w3642 w3652]
          tunnel: [w3642 w3651] -> w3638
          tunnel: [w3643 w3650] -> w3637
          frame False {
          }
          frame True {
            n1707 = flat-sequence {
              tunnel: w3652 -> [w3654]
              tunnel: w3653 -> [w3655]
              tunnel: [w3655] -> w3649
              tunnel: [w3654] -> w3648
              tunnel: [w3658] -> w3651
              tunnel: [w3657] -> w3650
              tunnel: w3649 -> [w3660]
              tunnel: w3648 -> [w3659]
              frame #0 {
              }
              frame #1 {
                n1708 = Enqueue Element(queue=w3660, element="Set Current Offset 3" ("元素"), error in (no error)=w3659) -> (queue out=w3657:refnum<queue>, error out=w3658:errorcluster)  [unwired: 2 out]
              }
            }
            n1709 = global write "EV05全局变量1.vi" "CAN接收"(FALSE ("CAN接收")) -> ()
            n1710 = global write "EV05全局变量1.vi" "高压校正接收"(FALSE ("高压校正接收")) -> ()
            n1711 = call <vilib>:"Set Busy.vi"() -> ()  [unwired: 4 in, 8 out]
            n1712 = property on="Current Offset结果 3" class="Bool (严格)"("Colors [4]"=cluster{u32, u32}[] [{0, 0}] ("颜色[4]"), "BoolText.Text"="" ("布尔文本.文本")) -> ()  [unwired: 2 in, 2 out]
          }
        }
      }
      event "充电能量阀值": Value Change {
        n1713 = event-data() -> ("NewVal"=w3665:bool)  [unwired: 6 out]
        n1714 = case shown="真" w3665 {
          tunnel: w3664 -> [w3667 w3677]
          tunnel: w3663 -> [w3666 w3676]
          tunnel: [w3666 w3675] -> w3662
          tunnel: [w3667 w3674] -> w3661
          frame False {
          }
          frame True {
            n1715 = flat-sequence {
              tunnel: w3676 -> [w3678]
              tunnel: w3677 -> [w3679]
              tunnel: [w3679] -> w3673
              tunnel: [w3678] -> w3672
              tunnel: [w3682] -> w3675
              tunnel: [w3681] -> w3674
              tunnel: w3673 -> [w3684]
              tunnel: w3672 -> [w3683]
              frame #0 {
              }
              frame #1 {
                n1716 = Enqueue Element(queue=w3684, element="Set Current Offset 4" ("元素"), error in (no error)=w3683) -> (queue out=w3681:refnum<queue>, error out=w3682:errorcluster)  [unwired: 2 out]
              }
            }
            n1717 = call <vilib>:"Set Busy.vi"() -> ()  [unwired: 4 in, 8 out]
            n1718 = global write "EV05全局变量1.vi" "CAN接收"(FALSE ("CAN接收")) -> ()
            n1719 = global write "EV05全局变量1.vi" "高压校正接收"(FALSE ("高压校正接收")) -> ()
            n1720 = property on="Current Offset结果 4" class="Bool (严格)"("Colors [4]"=cluster{u32, u32}[] [{0, 0}] ("颜色[4]"), "BoolText.Text"="" ("布尔文本.文本")) -> ()  [unwired: 2 in, 2 out]
          }
        }
      }
      event "分流器型号": Value Change {
        n1721 = event-data() -> ("NewVal"=w3689:bool)  [unwired: 6 out]
        n1722 = case shown="真" w3689 {
          tunnel: w3688 -> [w3691 w3700]
          tunnel: w3687 -> [w3690 w3699]
          tunnel: [w3690 w3698] -> w3686
          tunnel: [w3691 w3697] -> w3685
          frame False {
          }
          frame True {
            n1723 = local read "分流器大小"() -> (w3692:T2)
            n1724 = case shown="\"100A\", 默认" w3692 {
              tunnel: w3700 -> [w3704 w3708]
              tunnel: w3699 -> [w3703 w3707]
              tunnel: [w3703 w3706] -> w3698
              tunnel: [w3704 w3705] -> w3697
              frame "选择分流器型号" {
                n1725 = One Button Dialog(message="分流器为无效值" ("消息"), button name ("OK")="确定" ("按钮名称（“确定”）")) -> ()  [unwired: 1 out]
              }
              frame "100A", Default {
                n1726 = flat-sequence {
                  tunnel: w3707 -> [w3711]
                  tunnel: w3708 -> [w3712]
                  tunnel: [w3712] -> w3710
                  tunnel: [w3711] -> w3709
                  tunnel: [w3715] -> w3706
                  tunnel: [w3714] -> w3705
                  tunnel: w3710 -> [w3717]
                  tunnel: w3709 -> [w3716]
                  frame #0 {
                  }
                  frame #1 {
                    n1727 = Enqueue Element(queue=w3717, element="Set Current Gain 4" ("元素"), error in (no error)=w3716) -> (queue out=w3714:refnum<queue>, error out=w3715:errorcluster)  [unwired: 2 out]
                  }
                }
              }
            }
            n1728 = call <vilib>:"Set Busy.vi"() -> ()  [unwired: 4 in, 8 out]
            n1729 = global write "EV05全局变量1.vi" "CAN接收"(FALSE ("CAN接收")) -> ()
            n1730 = global write "EV05全局变量1.vi" "高压校正接收"(FALSE ("高压校正接收")) -> ()
            n1731 = property on="Current Gain结果 4" class="Bool (严格)"("Colors [4]"=cluster{u32, u32}[] [{0, 0}] ("颜色[4]"), "BoolText.Text"="" ("布尔文本.文本")) -> ()  [unwired: 2 in, 2 out]
          }
        }
      }
      event "Set Current Gain 3": Value Change {
        n1732 = event-data() -> ("NewVal"=w3722:bool)  [unwired: 6 out]
        n1733 = case shown="真" w3722 {
          tunnel: w3721 -> [w3724 w3734]
          tunnel: w3720 -> [w3723 w3733]
          tunnel: [w3723 w3732] -> w3719
          tunnel: [w3724 w3731] -> w3718
          frame False {
          }
          frame True {
            n1734 = flat-sequence {
              tunnel: w3733 -> [w3735]
              tunnel: w3734 -> [w3736]
              tunnel: [w3736] -> w3730
              tunnel: [w3735] -> w3729
              tunnel: [w3739] -> w3732
              tunnel: [w3738] -> w3731
              tunnel: w3730 -> [w3741]
              tunnel: w3729 -> [w3740]
              frame #0 {
              }
              frame #1 {
                n1735 = Enqueue Element(queue=w3741, element="Set Current Gain 3" ("元素"), error in (no error)=w3740) -> (queue out=w3738:refnum<queue>, error out=w3739:errorcluster)  [unwired: 2 out]
              }
            }
            n1736 = global write "EV05全局变量1.vi" "CAN接收"(FALSE ("CAN接收")) -> ()
            n1737 = call <vilib>:"Set Busy.vi"() -> ()  [unwired: 4 in, 8 out]
            n1738 = global write "EV05全局变量1.vi" "高压校正接收"(FALSE ("高压校正接收")) -> ()
            n1739 = property on="Current Gain结果 3" class="Bool (严格)"("Colors [4]"=cluster{u32, u32}[] [{0, 0}] ("颜色[4]"), "BoolText.Text"="" ("布尔文本.文本")) -> ()  [unwired: 2 in, 2 out]
          }
        }
      }
      event "Set Current Gain": Value Change {
        n1740 = event-data() -> ("NewVal"=w3746:bool)  [unwired: 6 out]
        n1741 = case shown="真" w3746 {
          tunnel: w3745 -> [w3748 w3759]
          tunnel: w3744 -> [w3747 w3758]
          tunnel: [w3747 w3757] -> w3743
          tunnel: [w3748 w3756] -> w3742
          frame False {
          }
          frame True {
            n1742 = flat-sequence {
              tunnel: w3758 -> [w3760]
              tunnel: w3759 -> [w3761]
              tunnel: [w3761] -> w3755
              tunnel: [w3760] -> w3754
              tunnel: [w3764] -> w3757
              tunnel: [w3763] -> w3756
              tunnel: w3755 -> [w3766]
              tunnel: w3754 -> [w3765]
              frame #0 {
              }
              frame #1 {
                n1743 = Enqueue Element(queue=w3766, element="Set Current Gain" ("元素"), error in (no error)=w3765) -> (queue out=w3763:refnum<queue>, error out=w3764:errorcluster)  [unwired: 2 out]
              }
            }
            n1744 = global write "EV05全局变量1.vi" "CAN接收"(FALSE ("CAN接收")) -> ()
            n1745 = global write "EV05全局变量1.vi" "高压校正接收"(FALSE ("高压校正接收")) -> ()
            n1746 = call <vilib>:"Set Busy.vi"() -> ()  [unwired: 4 in, 8 out]
            n1747 = local write "电流增益"("" ("5460Current Gain")) -> ()
            n1748 = property on="Current Gain结果" class="Bool (严格)"("Colors [4]"=cluster{u32, u32}[] [{0, 0}] ("颜色[4]"), "BoolText.Text"="" ("布尔文本.文本")) -> ()  [unwired: 2 in, 2 out]
          }
        }
      }
      event "Set Current Gain 2": Value Change {
        n1749 = event-data() -> ("NewVal"=w3771:bool)  [unwired: 6 out]
        n1750 = case shown="真" w3771 {
          tunnel: w3770 -> [w3773 w3784]
          tunnel: w3769 -> [w3772 w3783]
          tunnel: [w3772 w3782] -> w3768
          tunnel: [w3773 w3781] -> w3767
          frame False {
          }
          frame True {
            n1751 = flat-sequence {
              tunnel: w3783 -> [w3785]
              tunnel: w3784 -> [w3786]
              tunnel: [w3786] -> w3780
              tunnel: [w3785] -> w3779
              tunnel: [w3789] -> w3782
              tunnel: [w3788] -> w3781
              tunnel: w3780 -> [w3791]
              tunnel: w3779 -> [w3790]
              frame #0 {
              }
              frame #1 {
                n1752 = Enqueue Element(queue=w3791, element="Set Volt Gain" ("元素"), error in (no error)=w3790) -> (queue out=w3788:refnum<queue>, error out=w3789:errorcluster)  [unwired: 2 out]
              }
            }
            n1753 = global write "EV05全局变量1.vi" "CAN接收"(FALSE ("CAN接收")) -> ()
            n1754 = global write "EV05全局变量1.vi" "高压校正接收"(FALSE ("高压校正接收")) -> ()
            n1755 = call <vilib>:"Set Busy.vi"() -> ()  [unwired: 4 in, 8 out]
            n1756 = local write "Shunt Volt Gain"(" " ("5460Volt Gain")) -> ()
            n1757 = property on="Current Gain结果 2" class="Bool (严格)"("Colors [4]"=cluster{u32, u32}[] [{0, 0}] ("颜色[4]"), "BoolText.Text"="" ("布尔文本.文本")) -> ()  [unwired: 2 in, 2 out]
          }
        }
      }
      event "Volt Offset": Value Change {
        n1758 = event-data() -> ("NewVal"=w3796:bool)  [unwired: 6 out]
        n1759 = case shown="真" w3796 {
          tunnel: w3795 -> [w3798 w3809]
          tunnel: w3794 -> [w3797 w3808]
          tunnel: [w3797 w3807] -> w3793
          tunnel: [w3798 w3806] -> w3792
          frame False {
          }
          frame True {
            n1760 = flat-sequence {
              tunnel: w3808 -> [w3810]
              tunnel: w3809 -> [w3811]
              tunnel: [w3811] -> w3805
              tunnel: [w3810] -> w3804
              tunnel: [w3814] -> w3807
              tunnel: [w3813] -> w3806
              tunnel: w3805 -> [w3816]
              tunnel: w3804 -> [w3815]
              frame #0 {
              }
              frame #1 {
                n1761 = Enqueue Element(queue=w3816, element="Set Volt offset" ("元素"), error in (no error)=w3815) -> (queue out=w3813:refnum<queue>, error out=w3814:errorcluster)  [unwired: 2 out]
              }
            }
            n1762 = global write "EV05全局变量1.vi" "CAN接收"(FALSE ("CAN接收")) -> ()
            n1763 = global write "EV05全局变量1.vi" "高压校正接收"(FALSE ("高压校正接收")) -> ()
            n1764 = call <vilib>:"Set Busy.vi"() -> ()  [unwired: 4 in, 8 out]
            n1765 = local write "Shunt Volt Offset"(" " ("5460Volt Offset")) -> ()
            n1766 = property on="Current Offset结果 2" class="Bool (严格)"("Colors [4]"=cluster{u32, u32}[] [{0, 0}] ("颜色[4]"), "BoolText.Text"="" ("布尔文本.文本")) -> ()  [unwired: 2 in, 2 out]
          }
        }
      }
      event "Clear_in": Value Change {
        n1767 = event-data() -> ("NewVal"=w3821:bool)  [unwired: 6 out]
        n1768 = case shown="真" w3821 {
          tunnel: w3820 -> [w3823 w3831]
          tunnel: w3819 -> [w3822 w3830]
          tunnel: [w3822 w3829] -> w3818
          tunnel: [w3823 w3828] -> w3817
          frame False {
          }
          frame True {
            n1769 = flat-sequence {
              tunnel: w3830 -> [w3832]
              tunnel: w3831 -> [w3833]
              tunnel: [w3833] -> w3827
              tunnel: [w3832] -> w3826
              tunnel: [w3836] -> w3829
              tunnel: [w3835] -> w3828
              tunnel: w3827 -> [w3838]
              tunnel: w3826 -> [w3837]
              frame #0 {
              }
              frame #1 {
                n1770 = Enqueue Element(queue=w3838, element="Clear_in" ("元素"), error in (no error)=w3837) -> (queue out=w3835:refnum<queue>, error out=w3836:errorcluster)  [unwired: 2 out]
              }
            }
            n1771 = property on="Clear_in结果" class="Bool (严格)"("Colors [4]"=cluster{u32, u32}[] [{0, 0}] ("颜色[4]"), "BoolText.Text"="" ("布尔文本.文本")) -> ()  [unwired: 2 in, 2 out]
          }
        }
      }
      event "Clear_out": Value Change {
        n1772 = event-data() -> ("NewVal"=w3843:bool)  [unwired: 6 out]
        n1773 = case shown="真" w3843 {
          tunnel: w3842 -> [w3845 w3853]
          tunnel: w3841 -> [w3844 w3852]
          tunnel: [w3844 w3851] -> w3840
          tunnel: [w3845 w3850] -> w3839
          frame False {
          }
          frame True {
            n1774 = flat-sequence {
              tunnel: w3852 -> [w3854]
              tunnel: w3853 -> [w3855]
              tunnel: [w3855] -> w3849
              tunnel: [w3854] -> w3848
              tunnel: [w3858] -> w3851
              tunnel: [w3857] -> w3850
              tunnel: w3849 -> [w3860]
              tunnel: w3848 -> [w3859]
              frame #0 {
              }
              frame #1 {
                n1775 = Enqueue Element(queue=w3860, element="Clear_out" ("元素"), error in (no error)=w3859) -> (queue out=w3857:refnum<queue>, error out=w3858:errorcluster)  [unwired: 2 out]
              }
            }
            n1776 = property on="Clear_out结果" class="Bool (严格)"("Colors [4]"=cluster{u32, u32}[] [{0, 0}] ("颜色[4]"), "BoolText.Text"="" ("布尔文本.文本")) -> ()  [unwired: 2 in, 2 out]
          }
        }
      }
      event "Read1_in": Value Change {
        n1777 = event-data() -> ("NewVal"=w3865:bool)  [unwired: 6 out]
        n1778 = case shown="真" w3865 {
          tunnel: w3864 -> [w3867 w3884]
          tunnel: w3863 -> [w3866 w3883]
          tunnel: [w3866 w3882] -> w3862
          tunnel: [w3867 w3881] -> w3861
          frame False {
          }
          frame True {
            n1779 = flat-sequence {
              tunnel: w3883 -> [w3885]
              tunnel: w3884 -> [w3886]
              tunnel: [w3886] -> w3874
              tunnel: [w3885] -> w3872
              tunnel: w3874 -> [w3888]
              tunnel: [w3888] -> w3873
              tunnel: w3872 -> [w3887]
              tunnel: [w3887] -> w3871
              tunnel: w3873 -> [w3890]
              tunnel: [w3890] -> w3878
              tunnel: w3871 -> [w3889]
              tunnel: [w3889] -> w3876
              tunnel: w3878 -> [w3892]
              tunnel: [w3892] -> w3877
              tunnel: w3876 -> [w3891]
              tunnel: [w3891] -> w3875
              tunnel: [w3895] -> w3882
              tunnel: [w3894] -> w3881
              tunnel: w3877 -> [w3897]
              tunnel: w3875 -> [w3896]
              frame #0 {
              }
              frame #1 {
              }
              frame #2 {
              }
              frame #3 {
              }
              frame #4 {
                n1780 = Enqueue Element(queue=w3897, element="Read1_in" ("元素"), error in (no error)=w3896) -> (queue out=w3894:refnum<queue>, error out=w3895:errorcluster)  [unwired: 2 out]
              }
            }
            n1781 = global write "EV05全局变量1.vi" "高压校正接收"(FALSE ("高压校正接收")) -> ()
            n1782 = local write "AD1"(0.0 ("AD1 2")) -> ()
            n1783 = global write "EV05全局变量1.vi" "CAN接收"(FALSE ("CAN接收")) -> ()
            n1784 = call <vilib>:"Set Busy.vi"() -> ()  [unwired: 4 in, 8 out]
            n1785 = property on="Read1_in结果" class="Bool (严格)"("Colors [4]"=cluster{u32, u32}[] [{0, 0}] ("颜色[4]"), "BoolText.Text"="" ("布尔文本.文本")) -> ()  [unwired: 2 in, 2 out]
          }
        }
      }
      event "Read2_in": Value Change {
        n1786 = event-data() -> ("NewVal"=w3902:bool)  [unwired: 6 out]
        n1787 = case shown="真" w3902 {
          tunnel: w3901 -> [w3904 w3921]
          tunnel: w3900 -> [w3903 w3920]
          tunnel: [w3903 w3919] -> w3899
          tunnel: [w3904 w3918] -> w3898
          frame False {
          }
          frame True {
            n1788 = flat-sequence {
              tunnel: w3920 -> [w3922]
              tunnel: w3921 -> [w3923]
              tunnel: [w3923] -> w3911
              tunnel: [w3922] -> w3909
              tunnel: w3911 -> [w3925]
              tunnel: [w3925] -> w3910
              tunnel: w3909 -> [w3924]
              tunnel: [w3924] -> w3908
              tunnel: w3910 -> [w3927]
              tunnel: [w3927] -> w3915
              tunnel: w3908 -> [w3926]
              tunnel: [w3926] -> w3913
              tunnel: w3915 -> [w3929]
              tunnel: [w3929] -> w3914
              tunnel: w3913 -> [w3928]
              tunnel: [w3928] -> w3912
              tunnel: [w3932] -> w3919
              tunnel: [w3931] -> w3918
              tunnel: w3914 -> [w3934]
              tunnel: w3912 -> [w3933]
              frame #0 {
              }
              frame #1 {
              }
              frame #2 {
              }
              frame #3 {
              }
              frame #4 {
                n1789 = Enqueue Element(queue=w3934, element="Read2_in" ("元素"), error in (no error)=w3933) -> (queue out=w3931:refnum<queue>, error out=w3932:errorcluster)  [unwired: 2 out]
              }
            }
            n1790 = global write "EV05全局变量1.vi" "高压校正接收"(FALSE ("高压校正接收")) -> ()
            n1791 = global write "EV05全局变量1.vi" "CAN接收"(FALSE ("CAN接收")) -> ()
            n1792 = local write "AD2"(0.0 ("AD2 2")) -> ()
            n1793 = call <vilib>:"Set Busy.vi"() -> ()  [unwired: 4 in, 8 out]
            n1794 = property on="Read2_in结果" class="Bool (严格)"("Colors [4]"=cluster{u32, u32}[] [{0, 0}] ("颜色[4]"), "BoolText.Text"="" ("布尔文本.文本")) -> ()  [unwired: 2 in, 2 out]
          }
        }
      }
      event "Read2": Value Change {
        n1795 = event-data() -> ("NewVal"=w3939:bool)  [unwired: 6 out]
        n1796 = case shown="真" w3939 {
          tunnel: w3938 -> [w3941 w3958]
          tunnel: w3937 -> [w3940 w3957]
          tunnel: [w3940 w3956] -> w3936
          tunnel: [w3941 w3955] -> w3935
          frame False {
          }
          frame True {
            n1797 = flat-sequence {
              tunnel: w3957 -> [w3959]
              tunnel: w3958 -> [w3960]
              tunnel: [w3960] -> w3952
              tunnel: [w3959] -> w3950
              tunnel: w3952 -> [w3962]
              tunnel: [w3962] -> w3951
              tunnel: w3950 -> [w3961]
              tunnel: [w3961] -> w3949
              tunnel: w3951 -> [w3964]
              tunnel: [w3964] -> w3948
              tunnel: w3949 -> [w3963]
              tunnel: [w3963] -> w3946
              tunnel: w3948 -> [w3966]
              tunnel: [w3966] -> w3947
              tunnel: w3946 -> [w3965]
              tunnel: [w3965] -> w3945
              tunnel: [w3971] -> w3956
              tunnel: [w3970] -> w3955
              tunnel: w3947 -> [w3973]
              tunnel: w3945 -> [w3972]
              frame #0 {
              }
              frame #1 {
              }
              frame #2 {
              }
              frame #3 {
                n1798 = disable-structure shown="禁用" {
                  frame Disabled {
                    n1799 = local read "自动控制仪器"() -> (w3967:bool)
                    n1800 = case shown="真" w3967 {
                      frame False {
                      }
                      frame True {
                        n1801 = Wait (ms)(milliseconds to wait=u32 2000 ("等待时间（毫秒）")) -> ()  [unwired: 1 out]
                      }
                    }
                  }
                  frame Enabled {
                  }
                }
              }
              frame #4 {
                n1802 = Enqueue Element(queue=w3973, element="Read2" ("元素"), error in (no error)=w3972) -> (queue out=w3970:refnum<queue>, error out=w3971:errorcluster)  [unwired: 2 out]
              }
            }
            n1803 = global write "EV05全局变量1.vi" "高压校正接收"(FALSE ("高压校正接收")) -> ()
            n1804 = global write "EV05全局变量1.vi" "CAN接收"(FALSE ("CAN接收")) -> ()
            n1805 = local write "AD2"(u16 0 ("AD2")) -> ()
            n1806 = call <vilib>:"Set Busy.vi"() -> ()  [unwired: 4 in, 8 out]
            n1807 = property on="Read2结果" class="Bool (严格)"("Colors [4]"=cluster{u32, u32}[] [{0, 0}] ("颜色[4]"), "BoolText.Text"="" ("布尔文本.文本")) -> ()  [unwired: 2 in, 2 out]
          }
        }
      }
      event "Set": Value Change {
        n1808 = event-data() -> ("NewVal"=w3978:bool)  [unwired: 6 out]
        n1809 = case shown="真" w3978 {
          tunnel: w3977 -> [w3980 w3990]
          tunnel: w3976 -> [w3979 w3989]
          tunnel: [w3979 w3988] -> w3975
          tunnel: [w3980 w3987] -> w3974
          frame False {
          }
          frame True {
            n1810 = flat-sequence {
              tunnel: w3989 -> [w4001]
              tunnel: w3990 -> [w4002]
              tunnel: [w4002] -> w3986
              tunnel: [w4001] -> w3985
              tunnel: [w4005] -> w3988
              tunnel: [w4004] -> w3987
              tunnel: w3986 -> [w4007]
              tunnel: w3985 -> [w4006]
              frame #0 {
                n1811 = local read "REAL2"() -> (w3999:dbl)
                n1812 = local read "REAL1"() -> (w3998:dbl)
                n1813 = local read "AD1"() -> (w3994:u16)
                n1814 = local read "AD2"() -> (w3995:u16)
                n1815 = Subtract(x=w3999, y=w3998) -> (x-y=w3997:dbl)
                n1816 = Subtract(x=w3995, y=w3994) -> (x-y=w3993:u16)
                n1817 = Multiply(x=w3997, y=1000000.0) -> (x*y=w3996:dbl)
                n1818 = Divide(x=w3996, y=w3993) -> (x/y=w3992:dbl)
                n1819 = Round Toward -Infinity(1:w3992) -> (0:w3991:dbl)
                n1820 = local write "Gain"(w3991) -> ()
              }
              frame #1 {
                n1821 = Enqueue Element(queue=w4007, element="Set" ("元素"), error in (no error)=w4006) -> (queue out=w4004:refnum<queue>, error out=w4005:errorcluster)  [unwired: 2 out]
              }
            }
            n1822 = global write "EV05全局变量1.vi" "CAN接收"(FALSE ("CAN接收")) -> ()
            n1823 = global write "EV05全局变量1.vi" "高压校正接收"(FALSE ("高压校正接收")) -> ()
            n1824 = call <vilib>:"Set Busy.vi"() -> ()  [unwired: 4 in, 8 out]
            n1825 = property on="Set结果" class="Bool (严格)"("Colors [4]"=cluster{u32, u32}[] [{0, 0}] ("颜色[4]"), "BoolText.Text"="" ("布尔文本.文本")) -> ()  [unwired: 2 in, 2 out]
          }
        }
      }
      event "Set_in": Value Change {
        n1826 = event-data() -> ("NewVal"=w4012:bool)  [unwired: 6 out]
        n1827 = case shown="真" w4012 {
          tunnel: w4011 -> [w4014 w4024]
          tunnel: w4010 -> [w4013 w4023]
          tunnel: [w4013 w4022] -> w4009
          tunnel: [w4014 w4021] -> w4008
          frame False {
          }
          frame True {
            n1828 = flat-sequence {
              tunnel: w4023 -> [w4031]
              tunnel: w4024 -> [w4032]
              tunnel: [w4032] -> w4020
              tunnel: [w4031] -> w4019
              tunnel: [w4035] -> w4022
              tunnel: [w4034] -> w4021
              tunnel: w4020 -> [w4037]
              tunnel: w4019 -> [w4036]
              frame #0 {
                n1829 = local read "REAL2"() -> (w4029:dbl)
                n1830 = local read "REAL1"() -> (w4030:dbl)
                n1831 = local read "AD1"() -> (w4028:dbl)
                n1832 = local read "AD2"() -> (w4027:dbl)
                n1833 = call "Cal_Gain&offset.vi"("REAL2"=w4029, "REAL1"=w4030, "AD2"=w4027, "AD1"=w4028) -> ("Offset"=w4025:i32, "Gain"=w4026:dbl)  [unwired: 5 out]
                n1834 = local write "Gain"(w4026) -> ()
                n1835 = local write "Offset"(w4025) -> ()
              }
              frame #1 {
                n1836 = Enqueue Element(queue=w4037, element="Set_in" ("元素"), error in (no error)=w4036) -> (queue out=w4034:refnum<queue>, error out=w4035:errorcluster)  [unwired: 2 out]
              }
            }
            n1837 = global write "EV05全局变量1.vi" "CAN接收"(FALSE ("CAN接收")) -> ()
            n1838 = global write "EV05全局变量1.vi" "高压校正接收"(FALSE ("高压校正接收")) -> ()
            n1839 = call <vilib>:"Set Busy.vi"() -> ()  [unwired: 4 in, 8 out]
            n1840 = property on="Set_in结果" class="Bool (严格)"("Colors [4]"=cluster{u32, u32}[] [{0, 0}] ("颜色[4]"), "BoolText.Text"="" ("布尔文本.文本")) -> ()  [unwired: 2 in, 2 out]
          }
        }
      }
      event "连接GPIB": Value Change {
        n1841 = event-data() -> ("NewVal"=w4040:bool)  [unwired: 6 out]
        n1842 = case shown="真" w4040 {
          tunnel: w4039 -> [w4042 w4072]
          tunnel: [w4041 w4073] -> w4038
          frame False {
            w4044 = u8 2 ("禁用")
            n1843 = property on="输出100A" class="Bool"("Disabled"=w4044) -> ()  [unwired: 2 in, 2 out]
            n1844 = property on="输出200A" class="Bool"("Disabled"=w4044) -> ()  [unwired: 2 in, 2 out]
            n1845 = property on="输出自定义值2 2" class="Bool"("Disabled"=w4044) -> ()  [unwired: 2 in, 2 out]
            n1846 = property on="输出自定义值1 2" class="Bool"("Disabled"=w4044) -> ()  [unwired: 2 in, 2 out]
            n1847 = invoke on="输出200A" class="Bool" method="Reinit To Default"() -> ()  [unwired: 3 in, 3 out]
            n1848 = invoke on="输出100A" class="Bool" method="Reinit To Default"() -> ()  [unwired: 3 in, 3 out]
            n1849 = invoke on="输出自定义值2 2" class="Bool" method="Reinit To Default"() -> ()  [unwired: 3 in, 3 out]
            n1850 = invoke on="输出自定义值1 2" class="Bool" method="Reinit To Default"() -> ()  [unwired: 3 in, 3 out]
            n1851 = local read "VISA资源名称输出"() -> (w4049:refnum<visa-resource-name>)
            n1852 = flat-sequence {
              tunnel: w4049 -> [w4053]
              tunnel: [w4053] -> w4051
              tunnel: w4051 -> [w4055]
              tunnel: [w4055] -> w4050
              tunnel: w4050 -> [w4060]
              tunnel: [w4059] -> w4046
              tunnel: [w4058] -> w4045
              tunnel: [w4057] -> w4043
              tunnel: w4042 -> [w4056]
              tunnel: [w4065] -> w4047
              tunnel: [w4064] -> w4048
              tunnel: w4046 -> [w4067]
              tunnel: w4045 -> [w4066]
              tunnel: w4043 -> [w4063]
              frame #0 {
                n1853 = local write "连接状态 10"(FALSE ("连接状态")) -> ()
              }
              frame #1 {
                n1854 = Wait (ms)(milliseconds to wait=u32 50 ("等待时间（毫秒）")) -> ()  [unwired: 1 out]
              }
              frame #2 {
                w4057 = "outp off" ("写入缓冲区")
                n1855 = VISA Write(VISA resource name=w4060, write buffer=w4057, error in (no error)=w4056) -> (VISA resource name out=w4059:refnum<visa-resource-name>, error out=w4058:errorcluster)  [unwired: 1 out]
              }
              frame #3 {
                n1856 = VISA Write(VISA resource name=w4067, write buffer=w4063, error in (no error)=w4066) -> (VISA resource name out=w4064:refnum<visa-resource-name>, error out=w4065:errorcluster)  [unwired: 1 out]
                n1857 = local write "Actual"(0.0 ("实际值")) -> ()
                n1858 = Wait (ms)(milliseconds to wait=u32 50 ("等待时间（毫秒）")) -> ()  [unwired: 1 out]
                n1859 = local write "Set"(0.0 ("设定值")) -> ()
              }
            }
            n1860 = VISA Close(VISA resource name=w4048, error in (no error)=w4047) -> (error out=w4041:errorcluster)
          }
          frame True {
            n1861 = VISA Open(error in (no error)=w4072, VISA resource name="VISA resource name 2") -> (VISA resource name=w4070:refnum<visa-resource-name>, error out=w4076:errorcluster)  [unwired: 3 out]
            n1862 = property class="Instr"(reference=w4070, "Timeout"=u32 100 ("General Settings:Timeout Value")) -> (reference out=w4069:refnum<visa-resource-name>)  [unwired: 1 in, 1 out]
            n1863 = VISA Write(VISA resource name=w4069, write buffer="*rst" ("写入缓冲区"), error in (no error)=w4076) -> (VISA resource name out=w4075:refnum<visa-resource-name>, error out=w4073:errorcluster)  [unwired: 1 out]
            n1864 = Unbundle(w4073) -> ("status"=w4078:bool)  [unwired: 2 out]
            n1865 = case shown="假" w4078 {
              tunnel: w4075 -> [w4082 w4085]
              frame False {
                w4080 = u8 0 ("禁用")
                n1866 = local write "VISA资源名称输出"(w4082) -> ()
                n1867 = local write "连接状态 10"(TRUE ("连接状态")) -> ()
                n1868 = property on="连接状态 10" class="Bool (严格)"("Colors [4]"=cluster{u32, u32}[] [{6618880, 6618880}] ("颜色[4]")) -> ()  [unwired: 2 in, 2 out]
                n1869 = property on="输出100A" class="Bool"("Disabled"=w4080) -> ()  [unwired: 2 in, 2 out]
                n1870 = property on="输出200A" class="Bool"("Disabled"=w4080) -> ()  [unwired: 2 in, 2 out]
                n1871 = property on="输出自定义值2 2" class="Bool"("Disabled"=w4080) -> ()  [unwired: 2 in, 2 out]
                n1872 = property on="输出自定义值1 2" class="Bool"("Disabled"=w4080) -> ()  [unwired: 2 in, 2 out]
              }
              frame True {
                w4084 = u8 2 ("禁用")
                n1873 = local write "VISA资源名称输出"(w4085) -> ()
                n1874 = local write "连接状态 10"(FALSE ("连接状态")) -> ()
                n1875 = property on="连接状态 10" class="Bool (严格)"("Colors [4]"=cluster{u32, u32}[] [{15663131, 6618880}] ("颜色[4]")) -> ()  [unwired: 2 in, 2 out]
                n1876 = property on="输出100A" class="Bool"("Disabled"=w4084) -> ()  [unwired: 2 in, 2 out]
                n1877 = property on="输出200A" class="Bool"("Disabled"=w4084) -> ()  [unwired: 2 in, 2 out]
                n1878 = property on="输出自定义值2 2" class="Bool"("Disabled"=w4084) -> ()  [unwired: 2 in, 2 out]
                n1879 = property on="输出自定义值1 2" class="Bool"("Disabled"=w4084) -> ()  [unwired: 2 in, 2 out]
              }
            }
          }
        }
      }
      event "输出自定义值1": Value Change {
        n1880 = event-data() -> ("NewVal"=w4089:bool)  [unwired: 6 out]
        n1881 = case shown="真" w4089 {
          tunnel: w4088 -> [w4091 w4115]
          tunnel: [w4090 w4116] -> w4087
          frame False {
            w4092 = u8 0 ("禁用")
            n1882 = local read "VISA资源名称输出 10"() -> (w4098:refnum<visa-resource-name>)
            n1883 = local write "控制读取  5"(FALSE ("控制读取")) -> ()
            n1884 = flat-sequence {
              tunnel: [w4101] -> w4099
              tunnel: w4098 -> [w4101]
              tunnel: w4099 -> [w4105]
              tunnel: [w4104] -> w4097
              tunnel: [w4103] -> w4096
              tunnel: w4091 -> [w4102]
              tunnel: w4097 -> [w4109]
              tunnel: w4096 -> [w4108]
              tunnel: [w4109] -> w4095
              tunnel: [w4108] -> w4094
              tunnel: w4095 -> [w4113]
              tunnel: w4094 -> [w4112]
              tunnel: [w4110] -> w4090
              frame #0 {
                n1885 = Wait (ms)(milliseconds to wait=u32 200 ("等待时间（毫秒）")) -> ()  [unwired: 1 out]
              }
              frame #1 {
                n1886 = VISA Write(VISA resource name=w4105, write buffer="OUT:OFF" ("写入缓冲区"), error in (no error)=w4102) -> (VISA resource name out=w4104:refnum<visa-resource-name>, error out=w4103:errorcluster)  [unwired: 1 out]
              }
              frame #2 {
                n1887 = Wait (ms)(milliseconds to wait=u32 50 ("等待时间（毫秒）")) -> ()  [unwired: 1 out]
              }
              frame #3 {
                n1888 = local write "控制读取  5"(TRUE ("控制读取")) -> ()
                n1889 = VISA Write(VISA resource name=w4113, write buffer="OUT:OFF" ("写入缓冲区"), error in (no error)=w4112) -> (error out=w4110:errorcluster)  [unwired: 2 out]
              }
            }
            n1890 = property on="输出150V" class="Bool"("Disabled"=w4092) -> ()  [unwired: 2 in, 2 out]
            n1891 = property on="输出300V" class="Bool"("Disabled"=w4092) -> ()  [unwired: 2 in, 2 out]
            n1892 = property on="输出自定义值2" class="Bool"("Disabled"=w4092) -> ()  [unwired: 2 in, 2 out]
            n1893 = property on="输出自定义值1" class="Bool"("Disabled"=w4092) -> ()  [unwired: 2 in, 2 out]
          }
          frame True {
            w4125 = u8 2 ("禁用")
            w4127 = "," ("字符串")
            n1894 = local read "Volt1"() -> (w4118:dbl)
            n1895 = local write "Set"(w4118) -> ()
            n1896 = local write "控制读取  5"(FALSE ("控制读取")) -> ()
            n1897 = property on="输出150V" class="Bool"("Disabled"=w4125) -> ()  [unwired: 2 in, 2 out]
            n1898 = property on="输出300V" class="Bool"("Disabled"=w4125) -> ()  [unwired: 2 in, 2 out]
            n1899 = property on="输出自定义值2" class="Bool"("Disabled"=w4125) -> ()  [unwired: 2 in, 2 out]
            n1900 = Number To Fractional String(number=w4118, precision (6)=i16 2 ("精度(6)")) -> (F-format string=w4131:string)  [unwired: 2 out]
            n1901 = Number To Fractional String(number=0.2 ("数字"), precision (6)=i16 2 ("精度(6)")) -> (F-format string=w4130:string)  [unwired: 2 out]
            n1902 = Number To Fractional String(number=1.0 ("数字"), precision (6)=i16 2 ("精度(6)")) -> (F-format string=w4128:string)  [unwired: 2 out]
            n1903 = Number To Fractional String(number=320.0 ("数字"), precision (6)=i16 2 ("精度(6)")) -> (F-format string=w4129:string)  [unwired: 2 out]
            n1904 = Concatenate Strings(w4131, w4127, w4130, w4127, w4129, w4127, w4128, w4127, w4127, w4127) -> (w4126:string)
            n1905 = flat-sequence {
              tunnel: [w4150] -> w4138
              tunnel: [w4149] -> w4136
              tunnel: [w4148] -> w4134
              tunnel: w4126 -> [w4145]
              tunnel: w4115 -> [w4144]
              tunnel: w4138 -> [w4155]
              tunnel: [w4155] -> w4137
              tunnel: w4136 -> [w4154]
              tunnel: [w4154] -> w4135
              tunnel: w4134 -> [w4153]
              tunnel: [w4153] -> w4133
              tunnel: w4137 -> [w4159]
              tunnel: w4135 -> [w4158]
              tunnel: w4133 -> [_]
              tunnel: [w4157] -> w4142
              tunnel: [w4156] -> w4140
              tunnel: w4142 -> [w4165]
              tunnel: [w4165] -> w4141
              tunnel: w4140 -> [w4164]
              tunnel: [w4164] -> w4139
              tunnel: w4141 -> [w4168]
              tunnel: w4139 -> [w4167]
              tunnel: [w4166] -> w4116
              frame #0 {
                n1906 = Wait (ms)(milliseconds to wait=u32 200 ("等待时间（毫秒）")) -> ()  [unwired: 1 out]
              }
              frame #1 {
                n1907 = local read "VISA资源名称输出 10"() -> (w4147:refnum<visa-resource-name>)
                n1908 = Concatenate Strings("SET:GRO 12," ("写入缓冲区"), w4145, "\n") -> (w4148:string)
                n1909 = VISA Write(VISA resource name=w4147, write buffer=w4148, error in (no error)=w4144) -> (VISA resource name out=w4150:refnum<visa-resource-name>, error out=w4149:errorcluster)  [unwired: 1 out]
              }
              frame #2 {
                n1910 = Wait (ms)(milliseconds to wait=u32 50 ("等待时间（毫秒）")) -> ()  [unwired: 1 out]
              }
              frame #3 {
                n1911 = Concatenate Strings("SET:STE 12" ("写入缓冲区"), "\n") -> (w4160:string)
                n1912 = VISA Write(VISA resource name=w4159, write buffer=w4160, error in (no error)=w4158) -> (VISA resource name out=w4157:refnum<visa-resource-name>, error out=w4156:errorcluster)  [unwired: 1 out]
              }
              frame #4 {
                n1913 = Wait (ms)(milliseconds to wait=u32 200 ("等待时间（毫秒）")) -> ()  [unwired: 1 out]
              }
              frame #5 {
                n1914 = Concatenate Strings("OUT:ON" ("写入缓冲区"), "\n") -> (w4173:string)
                n1915 = Wait (ms)(milliseconds to wait=u32 50 ("等待时间（毫秒）")) -> ()  [unwired: 1 out]
                n1916 = VISA Write(VISA resource name=w4168, write buffer=w4173, error in (no error)=w4167) -> (VISA resource name out=w4170:refnum<visa-resource-name>, error out=w4166:errorcluster)  [unwired: 1 out]
                n1917 = local write "VISA资源名称输出 10"(w4170) -> ()
              }
              frame #6 {
                n1918 = local write "控制读取  5"(TRUE ("控制读取")) -> ()
              }
            }
          }
        }
      }
      event "输出自定义值2": Value Change {
        n1919 = event-data() -> ("NewVal"=w4177:bool)  [unwired: 6 out]
        n1920 = case shown="真" w4177 {
          tunnel: w4176 -> [w4178 w4207]
          tunnel: [w4180 w4205] -> w4175
          frame False {
            w4181 = u8 0 ("禁用")
            n1921 = local read "VISA资源名称输出 10"() -> (w4187:refnum<visa-resource-name>)
            n1922 = local write "控制读取  5"(FALSE ("控制读取")) -> ()
            n1923 = flat-sequence {
              tunnel: [w4191] -> w4188
              tunnel: w4187 -> [w4191]
              tunnel: [w4189] -> w4179
              tunnel: w4178 -> [w4189]
              tunnel: w4188 -> [w4195]
              tunnel: [w4194] -> w4186
              tunnel: [w4193] -> w4185
              tunnel: w4179 -> [w4192]
              tunnel: w4186 -> [w4199]
              tunnel: w4185 -> [w4198]
              tunnel: [w4199] -> w4184
              tunnel: [w4198] -> w4183
              tunnel: w4184 -> [w4203]
              tunnel: w4183 -> [w4202]
              tunnel: [w4200] -> w4180
              frame #0 {
                n1924 = Wait (ms)(milliseconds to wait=u32 200 ("等待时间（毫秒）")) -> ()  [unwired: 1 out]
              }
              frame #1 {
                n1925 = VISA Write(VISA resource name=w4195, write buffer="OUT:OFF" ("写入缓冲区"), error in (no error)=w4192) -> (VISA resource name out=w4194:refnum<visa-resource-name>, error out=w4193:errorcluster)  [unwired: 1 out]
              }
              frame #2 {
                n1926 = Wait (ms)(milliseconds to wait=u32 50 ("等待时间（毫秒）")) -> ()  [unwired: 1 out]
              }
              frame #3 {
                n1927 = local write "控制读取  5"(TRUE ("控制读取")) -> ()
                n1928 = VISA Write(VISA resource name=w4203, write buffer="OUT:OFF" ("写入缓冲区"), error in (no error)=w4202) -> (error out=w4200:errorcluster)  [unwired: 2 out]
              }
            }
            n1929 = property on="输出150V" class="Bool"("Disabled"=w4181) -> ()  [unwired: 2 in, 2 out]
            n1930 = property on="输出300V" class="Bool"("Disabled"=w4181) -> ()  [unwired: 2 in, 2 out]
            n1931 = property on="输出自定义值2" class="Bool"("Disabled"=w4181) -> ()  [unwired: 2 in, 2 out]
            n1932 = property on="输出自定义值1" class="Bool"("Disabled"=w4181) -> ()  [unwired: 2 in, 2 out]
          }
          frame True {
            w4212 = i16 2 ("精度(6)")
            w4213 = u8 2 ("禁用")
            w4215 = "," ("字符串")
            n1933 = local read "Volt2"() -> (w4209:dbl)
            n1934 = local write "控制读取  5"(FALSE ("控制读取")) -> ()
            n1935 = property on="输出150V" class="Bool"("Disabled"=w4213) -> ()  [unwired: 2 in, 2 out]
            n1936 = property on="输出300V" class="Bool"("Disabled"=w4213) -> ()  [unwired: 2 in, 2 out]
            n1937 = property on="输出自定义值1" class="Bool"("Disabled"=w4213) -> ()  [unwired: 2 in, 2 out]
            n1938 = Number To Fractional String(number=w4209, precision (6)=w4212) -> (F-format string=w4219:string)  [unwired: 2 out]
            n1939 = Number To Fractional String(number=0.2 ("数字"), precision (6)=w4212) -> (F-format string=w4218:string)  [unwired: 2 out]
            n1940 = Number To Fractional String(number=1.0 ("数字"), precision (6)=w4212) -> (F-format string=w4216:string)  [unwired: 2 out]
            n1941 = Number To Fractional String(number=320.0 ("数字"), precision (6)=w4212) -> (F-format string=w4217:string)  [unwired: 2 out]
            n1942 = local write "Set"(w4209) -> ()
            n1943 = Concatenate Strings(w4219, w4215, w4218, w4215, w4217, w4215, w4216, w4215, w4215, w4215) -> (w4214:string)
            n1944 = flat-sequence {
              tunnel: [w4238] -> w4226
              tunnel: [w4237] -> w4224
              tunnel: [w4236] -> w4222
              tunnel: w4214 -> [w4233]
              tunnel: w4207 -> [w4232]
              tunnel: w4226 -> [w4243]
              tunnel: [w4243] -> w4225
              tunnel: w4224 -> [w4242]
              tunnel: [w4242] -> w4223
              tunnel: w4222 -> [w4241]
              tunnel: [w4241] -> w4221
              tunnel: w4225 -> [w4247]
              tunnel: w4223 -> [w4246]
              tunnel: w4221 -> [_]
              tunnel: [w4245] -> w4230
              tunnel: [w4244] -> w4228
              tunnel: w4230 -> [w4253]
              tunnel: [w4253] -> w4229
              tunnel: w4228 -> [w4252]
              tunnel: [w4252] -> w4227
              tunnel: w4229 -> [w4256]
              tunnel: w4227 -> [w4255]
              tunnel: [w4254] -> w4206
              tunnel: w4206 -> [w4262]
              tunnel: [w4262] -> w4205
              frame #0 {
                n1945 = Wait (ms)(milliseconds to wait=u32 200 ("等待时间（毫秒）")) -> ()  [unwired: 1 out]
              }
              frame #1 {
                n1946 = local read "VISA资源名称输出 10"() -> (w4235:refnum<visa-resource-name>)
                n1947 = Concatenate Strings("SET:GRO 12," ("写入缓冲区"), w4233, "\n") -> (w4236:string)
                n1948 = VISA Write(VISA resource name=w4235, write buffer=w4236, error in (no error)=w4232) -> (VISA resource name out=w4238:refnum<visa-resource-name>, error out=w4237:errorcluster)  [unwired: 1 out]
              }
              frame #2 {
                n1949 = Wait (ms)(milliseconds to wait=u32 50 ("等待时间（毫秒）")) -> ()  [unwired: 1 out]
              }
              frame #3 {
                n1950 = Concatenate Strings("SET:STE 12" ("写入缓冲区"), "\n") -> (w4248:string)
                n1951 = VISA Write(VISA resource name=w4247, write buffer=w4248, error in (no error)=w4246) -> (VISA resource name out=w4245:refnum<visa-resource-name>, error out=w4244:errorcluster)  [unwired: 1 out]
              }
              frame #4 {
                n1952 = Wait (ms)(milliseconds to wait=u32 200 ("等待时间（毫秒）")) -> ()  [unwired: 1 out]
              }
              frame #5 {
                n1953 = Concatenate Strings("OUT:ON" ("写入缓冲区"), "\n") -> (w4261:string)
                n1954 = Wait (ms)(milliseconds to wait=u32 50 ("等待时间（毫秒）")) -> ()  [unwired: 1 out]
                n1955 = VISA Write(VISA resource name=w4256, write buffer=w4261, error in (no error)=w4255) -> (VISA resource name out=w4258:refnum<visa-resource-name>, error out=w4254:errorcluster)  [unwired: 1 out]
                n1956 = local write "VISA资源名称输出 10"(w4258) -> ()
              }
              frame #6 {
                n1957 = local write "控制读取  5"(TRUE ("控制读取")) -> ()
              }
            }
          }
        }
      }
      event "连接电压源": Value Change {
        n1958 = event-data() -> ("NewVal"=w4266:bool)  [unwired: 6 out]
        n1959 = case shown="真" w4266 {
          tunnel: [w4270 w4300] -> w4265
          tunnel: w4264 -> [w4269 w4299]
          frame False {
            w4271 = u8 2 ("禁用")
            n1960 = property on="输出150V" class="Bool"("Disabled"=w4271) -> ()  [unwired: 2 in, 2 out]
            n1961 = property on="输出300V" class="Bool"("Disabled"=w4271) -> ()  [unwired: 2 in, 2 out]
            n1962 = property on="输出自定义值2" class="Bool"("Disabled"=w4271) -> ()  [unwired: 2 in, 2 out]
            n1963 = property on="输出自定义值1" class="Bool"("Disabled"=w4271) -> ()  [unwired: 2 in, 2 out]
            n1964 = invoke on="输出300V" class="Bool" method="Reinit To Default"() -> ()  [unwired: 3 in, 3 out]
            n1965 = invoke on="输出150V" class="Bool" method="Reinit To Default"() -> ()  [unwired: 3 in, 3 out]
            n1966 = invoke on="输出自定义值2" class="Bool" method="Reinit To Default"() -> ()  [unwired: 3 in, 3 out]
            n1967 = invoke on="输出自定义值1" class="Bool" method="Reinit To Default"() -> ()  [unwired: 3 in, 3 out]
            n1968 = local read "VISA资源名称输出 10"() -> (w4276:refnum<visa-resource-name>)
            n1969 = flat-sequence {
              tunnel: w4276 -> [w4281]
              tunnel: [w4281] -> w4278
              tunnel: w4269 -> [w4279]
              tunnel: [w4279] -> w4267
              tunnel: w4278 -> [w4284]
              tunnel: [w4284] -> w4277
              tunnel: [w4282] -> w4268
              tunnel: w4267 -> [w4282]
              tunnel: w4277 -> [w4288]
              tunnel: [w4287] -> w4273
              tunnel: [w4286] -> w4272
              tunnel: w4268 -> [w4285]
              tunnel: [w4292] -> w4274
              tunnel: [w4293] -> w4275
              tunnel: w4273 -> [w4293]
              tunnel: w4272 -> [w4292]
              frame #0 {
                n1970 = local write "连接状态 10"(FALSE ("连接状态")) -> ()
              }
              frame #1 {
                n1971 = Wait (ms)(milliseconds to wait=u32 50 ("等待时间（毫秒）")) -> ()  [unwired: 1 out]
              }
              frame #2 {
                n1972 = VISA Write(VISA resource name=w4288, write buffer="OUT:OFF" ("写入缓冲区"), error in (no error)=w4285) -> (VISA resource name out=w4287:refnum<visa-resource-name>, error out=w4286:errorcluster)  [unwired: 1 out]
              }
              frame #3 {
                w4290 = 0.0 ("电压/V")
                n1973 = local write "电流/A 4"(w4290) -> ()
                n1974 = local write "Actual"(w4290) -> ()
                n1975 = Wait (ms)(milliseconds to wait=u32 50 ("等待时间（毫秒）")) -> ()  [unwired: 1 out]
              }
            }
            n1976 = VISA Close(VISA resource name=w4275, error in (no error)=w4274) -> (error out=w4270:errorcluster)
          }
          frame True {
            n1977 = VISA Open(error in (no error)=w4299, VISA resource name="VISA resource name 4") -> (VISA resource name=w4297:refnum<visa-resource-name>, error out=w4296:errorcluster)  [unwired: 1 in, 2 out]
            n1978 = property class="Instr"(reference=w4297, error in=w4296, "Timeout"=u32 100 ("General Settings:Timeout Value")) -> (reference out=w4294:refnum<visa-resource-name>, error out=w4295:errorcluster)
            n1979 = call-poly "VISA Configure Serial Port"("VISA resource name"=w4294, "error in (no error)"=w4295) -> ("VISA resource name out"=w4303:refnum<visa-resource-name>, "error out"=w4300:errorcluster)  [unwired: 4 in, 8 out]
            n1980 = Unbundle(w4300) -> ("status"=w4302:bool)  [unwired: 2 out]
            n1981 = case shown="假" w4302 {
              tunnel: w4303 -> [w4307 w4310]
              frame False {
                w4305 = u8 0 ("禁用")
                n1982 = local write "VISA资源名称输出 10"(w4307) -> ()
                n1983 = local write "连接状态 10"(TRUE ("连接状态")) -> ()
                n1984 = property on="输出150V" class="Bool"("Disabled"=w4305) -> ()  [unwired: 2 in, 2 out]
                n1985 = property on="输出300V" class="Bool"("Disabled"=w4305) -> ()  [unwired: 2 in, 2 out]
                n1986 = property on="输出自定义值2" class="Bool"("Disabled"=w4305) -> ()  [unwired: 2 in, 2 out]
                n1987 = property on="输出自定义值1" class="Bool"("Disabled"=w4305) -> ()  [unwired: 2 in, 2 out]
                n1988 = property on="连接状态 10" class="Bool (严格)"("Colors [4]"=cluster{u32, u32}[] [{6618880, 6618880}] ("颜色[4]")) -> ()  [unwired: 2 in, 2 out]
              }
              frame True {
                w4309 = u8 2 ("禁用")
                n1989 = local write "VISA资源名称输出 10"(w4310) -> ()
                n1990 = local write "连接状态 10"(FALSE ("连接状态")) -> ()
                n1991 = property on="输出150V" class="Bool"("Disabled"=w4309) -> ()  [unwired: 2 in, 2 out]
                n1992 = property on="输出300V" class="Bool"("Disabled"=w4309) -> ()  [unwired: 2 in, 2 out]
                n1993 = property on="输出自定义值2" class="Bool"("Disabled"=w4309) -> ()  [unwired: 2 in, 2 out]
                n1994 = property on="输出自定义值1" class="Bool"("Disabled"=w4309) -> ()  [unwired: 2 in, 2 out]
                n1995 = property on="连接状态 10" class="Bool (严格)"("Colors [4]"=cluster{u32, u32}[] [{15663131, 6618880}] ("颜色[4]")) -> ()  [unwired: 2 in, 2 out]
              }
            }
          }
        }
      }
      event "Set_out": Value Change {
        n1996 = event-data() -> ("NewVal"=w4316:bool)  [unwired: 6 out]
        n1997 = case shown="真" w4316 {
          tunnel: w4315 -> [w4318 w4328]
          tunnel: w4314 -> [w4317 w4327]
          tunnel: [w4317 w4326] -> w4313
          tunnel: [w4318 w4325] -> w4312
          frame False {
          }
          frame True {
            n1998 = flat-sequence {
              tunnel: w4327 -> [w4335]
              tunnel: w4328 -> [w4336]
              tunnel: [w4336] -> w4324
              tunnel: [w4335] -> w4323
              tunnel: [w4339] -> w4326
              tunnel: [w4338] -> w4325
              tunnel: w4324 -> [w4341]
              tunnel: w4323 -> [w4340]
              frame #0 {
                n1999 = local read "REAL2"() -> (w4333:dbl)
                n2000 = local read "REAL1"() -> (w4334:dbl)
                n2001 = local read "AD1"() -> (w4332:dbl)
                n2002 = local read "AD2"() -> (w4331:dbl)
                n2003 = call "Cal_Gain&offset.vi"("REAL2"=w4333, "REAL1"=w4334, "AD2"=w4331, "AD1"=w4332) -> ("Offset"=w4330:i32, "Gain"=w4329:dbl)  [unwired: 5 out]
                n2004 = local write "Offset"(w4330) -> ()
                n2005 = local write "Gain"(w4329) -> ()
              }
              frame #1 {
                n2006 = Enqueue Element(queue=w4341, element="Set_out" ("元素"), error in (no error)=w4340) -> (queue out=w4338:refnum<queue>, error out=w4339:errorcluster)  [unwired: 2 out]
              }
            }
            n2007 = global write "EV05全局变量1.vi" "CAN接收"(FALSE ("CAN接收")) -> ()
            n2008 = global write "EV05全局变量1.vi" "高压校正接收"(FALSE ("高压校正接收")) -> ()
            n2009 = call <vilib>:"Set Busy.vi"() -> ()  [unwired: 4 in, 8 out]
            n2010 = property on="Set_out结果" class="Bool (严格)"("Colors [4]"=cluster{u32, u32}[] [{0, 0}] ("颜色[4]"), "BoolText.Text"="" ("布尔文本.文本")) -> ()  [unwired: 2 in, 2 out]
          }
        }
      }
    }
  }
  n2011 = while {
    tunnel: "error in (no error)" -> [w4349]
    tunnel: [w4342] -> _
    stop <- "停止 7" stop-if-true
    n2012 = local read "连接状态 10"() -> (w4350:bool)
    n2013 = local read "控制读取  2"() -> (w4351:bool)
    n2014 = Tick Count (ms)() -> (millisecond timer value=w4347:u32)
    n2015 = And(x=w4350, y=w4351) -> (x .and. y?=w4343:bool)
    n2016 = case shown="真" w4343 {
      tunnel: w4349 -> [_ w4365]
      tunnel: [_ w4357] -> w4348
      tunnel: w4347 -> [w4354 w4359]
      tunnel: [w4354 w4359] -> w4346
      tunnel: [w4355 w4356] -> w4345
      frame False {
        n2017 = Tick Count (ms)() -> (millisecond timer value=w4355:u32)
      }
      frame True {
        n2018 = local read "VISA资源名称输出"() -> (w4369:refnum<visa-resource-name>)
        n2019 = VISA Write(VISA resource name=w4369, write buffer="MEAS:curr?" ("写入缓冲区"), error in (no error)=w4365) -> (VISA resource name out=w4364:refnum<visa-resource-name>, error out=w4363:errorcluster)  [unwired: 1 out]
        n2020 = flat-sequence {
          tunnel: w4364 -> [w4374]
          tunnel: w4363 -> [w4373]
          tunnel: [w4374] -> w4362
          tunnel: [w4373] -> w4361
          frame #0 {
            n2021 = Wait (ms)(milliseconds to wait=u32 50 ("等待时间（毫秒）")) -> ()  [unwired: 1 out]
          }
        }
        n2022 = VISA Read(VISA resource name=w4362, byte count=u32 20 ("字节总数"), error in (no error)=w4361) -> (read buffer=w4367:string, error out=w4358:errorcluster)  [unwired: 2 out]
        n2023 = Fract/Exp String To Number(string=w4367) -> (number=w4366:dbl)  [unwired: 4 out]
        n2024 = local write "Actual"(w4366) -> ()
        n2025 = flat-sequence {
          tunnel: w4358 -> [w4371]
          tunnel: [w4371] -> w4357
          tunnel: [w4370] -> w4356
          frame #0 {
            n2026 = Tick Count (ms)() -> (millisecond timer value=w4370:u32)
          }
        }
      }
    }
    n2027 = Wait (ms)(milliseconds to wait=u32 50 ("等待时间（毫秒）")) -> ()  [unwired: 1 out]
    n2028 = Subtract(x=w4345, y=w4346) -> (x-y=→"x-y":u32)
    n2029 = call <vilib>:"Clear Errors.vi"("error in (no error)"=w4348) -> ("error out"=w4342:errorcluster)  [unwired: 6 out]
  }
  n2030 = while {
    tunnel: w7 -> [w4385]
    tunnel: w41 -> [w4384]
    tunnel: [w4377] -> w3
    tunnel: [w4376] -> w4
    stop <- w4387 stop-if-true
    n2031 = local read "CAN路数"() -> (w4378:u16)
    n2032 = local read "CAN卡类型"() -> (w4380:u32)
    n2033 = local read "设备索引"() -> (w4379:u16)
    n2034 = local read "停止 2"() -> (w4387:bool)
    n2035 = call "receiver-8.6.vi"("CAN端口"=w4378, "设备索引号"=w4379, "CAN卡类型"=w4380) -> ("输出簇"=w4375:T14, "接收成功"=w4386:bool)  [unwired: 1 in, 4 out]
    n2036 = case shown="真" w4386 {
      tunnel: w4385 -> [w4398 w4403]
      tunnel: w4384 -> [w4397 w4402]
      tunnel: w4375 -> [_ w4401]
      tunnel: [w4398 w4400] -> w4382
      tunnel: [w4397 w4399] -> w4381
      frame False {
      }
      frame True {
        n2037 = Enqueue Element(queue=w4403, element=w4401, error in (no error)=w4402) -> (queue out=w4400:refnum<queue>, error out=w4399:errorcluster)  [unwired: 1 in, 1 out]
      }
    }
    n2038 = call "已用时间"() -> ("Elapsed Time (s)"=w4383:dbl)  [unwired: 12 in, 7 out]
    n2039 = case shown="1" w4383 {
      tunnel: w4382 -> [w4388 w4391]
      tunnel: w4381 -> [w4389 w4393]
      tunnel: w4380 -> [_ w4396]
      tunnel: w4379 -> [_ w4395]
      tunnel: w4378 -> [_ w4394]
      tunnel: [w4389 w4392] -> w4377
      tunnel: [w4388 w4390] -> w4376
      frame 0, Default {
      }
      frame 1 {
        n2040 = dll-call lib="PTH1ƒabs FBluewave New EnergySVN_WorkBMS_Monitor_Bnet01trunk\"BMS_Monitor - 91ç‰ˆ - new protocaldata\nkerneldlls\nusbcan.dll" fn="VCI_ClearBuffer"(error in=w4393, "DeviceType"=w4396, "DeviceInd"=w4395, "CANInd"=w4394) -> (error out=w4392:errorcluster)  [unwired: 3 in, 4 out]
        n2041 = Flush Queue(queue=w4391) -> (queue out=w4390:refnum<queue>)  [unwired: 1 in, 2 out]
      }
    }
  }
  n2042 = global read "功能码全局.vi" "13"() -> (w17:bool[])
  n2043 = Index Array(array=w17) -> (element #5=w8:bool, element #6=w9:bool, element #7=w10:bool, element #8=w11:bool)  [unwired: 8 in, 4 out]
  n2044 = Not(x=w8) -> (.not. x?=w16:bool)
  n2045 = Not(x=w9) -> (.not. x?=w13:bool)
  n2046 = Compound Arithmetic op=AND(w11, w10, w9, w8) -> (w12:bool)
  n2047 = property on="电流校正 2" class="TabCtl (严格)"("Visible"=w16) -> ()  [unwired: 2 in, 2 out]
  n2048 = property on="电流校正" class="TabCtl (严格)"("Visible"=w16) -> ()  [unwired: 2 in, 2 out]
  n2049 = Not(x=w10) -> (.not. x?=w14:bool)
  n2050 = Not(x=w11) -> (.not. x?=w15:bool)
  n2051 = property on="一键校正" class="Bool (严格)"("Visible"=w12) -> ()  [unwired: 2 in, 2 out]
  n2052 = property on="外总压" class="TabCtl (严格)"("Visible"=w13) -> ()  [unwired: 2 in, 2 out]
  n2053 = property on="内总压" class="TabCtl (严格)"("Visible"=w14) -> ()  [unwired: 2 in, 2 out]
  n2054 = property on="分流器" class="TabCtl (严格)"("Visible"=w15) -> ()  [unwired: 2 in, 2 out]
  n2055 = Release Queue(queue=w4, force destroy? (F)=TRUE ("强制销毁？(F)"), error in (no error)=w3) -> (error out=w6:errorcluster)  [unwired: 2 out]
  n2056 = call <vilib>:"Clear Errors.vi"("error in (no error)"=w6) -> ()  [unwired: 7 out]
  n2057 = control-ref of="结果"() -> (w21:refnum<vi>)
  n2058 = for {
    N: 40 -> [_]
    tunnel: w21 -> [w4408]
    i -> [w4406]
    n2059 = Bundle(w4406, 0) -> (w4404:cluster{i32, i32})  [unwired: 1 out]
    n2060 = property class="MCListbox (严格)"(reference=w4408, "ActiveCell"=w4404, "CellBG"=u32 16448250) -> ()  [unwired: 1 in, 2 out]
  }
  n2061 = property class="MCListbox (严格)"(reference=w21, "ItemNames"=string[][] [] ("项名")) -> ()  [unwired: 1 in, 2 out]
  n2062 = global write "EV05全局变量1.vi" "CAN接收"(TRUE ("CAN接收")) -> ()
  n2063 = local write "监控状态"(FALSE ("监控状态")) -> ()
  n2064 = property on="外总压" class="DigNum (严格)"("NumText.BGColor"=w18) -> ()  [unwired: 2 in, 2 out]
  n2065 = property on="内总压" class="DigNum (严格)"("NumText.BGColor"=w18) -> ()  [unwired: 2 in, 2 out]
  n2066 = property on="电流" class="DigNum (严格)"("NumText.BGColor"=w18) -> ()  [unwired: 2 in, 2 out]
  n2067 = call "自适应屏幕分辨率.vi"() -> ()  [unwired: 16 in]
  n2068 = Release Queue(queue=w30, force destroy? (F)=TRUE ("强制销毁？(F)"), error in (no error)=w31) -> (error out=w28:errorcluster)  [unwired: 2 out]
  n2069 = property on="连接状态 10" class="Bool (严格)"("Colors [4]"=w24) -> ()  [unwired: 2 in, 2 out]
  n2070 = property on="连接状态 10" class="Bool (严格)"("Colors [4]"=w24) -> ()  [unwired: 2 in, 2 out]
  n2071 = property on="监控状态" class="Bool (严格)"("Colors [4]"=w24) -> ()  [unwired: 2 in, 2 out]
  n2072 = call <vilib>:"Clear Errors.vi"("error in (no error)"=w28) -> ()  [unwired: 7 out]
  n2073 = property on="Set结果" class="Bool (严格)"("Colors [4]"=w24, "BoolText.Text"=w23) -> ()  [unwired: 2 in, 2 out]
  n2074 = property on="Read1结果" class="Bool (严格)"("Colors [4]"=w24, "BoolText.Text"=w23) -> ()  [unwired: 2 in, 2 out]
  n2075 = local write "行号"(0.0 ("行号")) -> ()
  n2076 = property on="Clear_in结果" class="Bool (严格)"("Colors [4]"=w24, "BoolText.Text"=w23) -> ()  [unwired: 2 in, 2 out]
  n2077 = property on="Current Offset结果 2" class="Bool (严格)"("Colors [4]"=w24, "BoolText.Text"=w23) -> ()  [unwired: 2 in, 2 out]
  n2078 = property on="Current Offset结果 4" class="Bool (严格)"("Colors [4]"=w24, "BoolText.Text"=w23) -> ()  [unwired: 2 in, 2 out]
  n2079 = property on="Current Gain结果 4" class="Bool (严格)"("Colors [4]"=w24, "BoolText.Text"=w23) -> ()  [unwired: 2 in, 2 out]
  n2080 = property on="Set_out结果" class="Bool (严格)"("Colors [4]"=w24, "BoolText.Text"=w23) -> ()  [unwired: 2 in, 2 out]
  n2081 = local write "停止"(w35) -> ()
  n2082 = property on="Read2_Out结果" class="Bool (严格)"("Colors [4]"=w24, "BoolText.Text"=w23) -> ()  [unwired: 2 in, 2 out]
  n2083 = property on="Read1_Out结果" class="Bool (严格)"("Colors [4]"=w24, "BoolText.Text"=w23) -> ()  [unwired: 2 in, 2 out]
  n2084 = property on="Current Offset结果" class="Bool (严格)"("Colors [4]"=w24, "BoolText.Text"=w23) -> ()  [unwired: 2 in, 2 out]
  n2085 = property on="Current Offset结果 3" class="Bool (严格)"("Colors [4]"=w24, "BoolText.Text"=w23) -> ()  [unwired: 2 in, 2 out]
  n2086 = property on="Current Gain结果 3" class="Bool (严格)"("Colors [4]"=w24, "BoolText.Text"=w23) -> ()  [unwired: 2 in, 2 out]
  n2087 = local write "停止 3"(w35) -> ()
  n2088 = local write "停止 2"(w35) -> ()
  n2089 = local write "停止 6"(w35) -> ()
  n2090 = local write "停止 7"(w35) -> ()
  n2091 = property on="Read2结果" class="Bool (严格)"("Colors [4]"=w24, "BoolText.Text"=w23) -> ()  [unwired: 2 in, 2 out]
  n2092 = property on="Current Offset结果" class="Bool (严格)"("Colors [4]"=w24, "BoolText.Text"=w23) -> ()  [unwired: 2 in, 2 out]
  n2093 = property on="Current Gain结果" class="Bool (严格)"("Colors [4]"=w24, "BoolText.Text"=w23) -> ()  [unwired: 2 in, 2 out]
  n2094 = property on="Clear结果" class="Bool (严格)"("Colors [4]"=w24, "BoolText.Text"=w23) -> ()  [unwired: 2 in, 2 out]
  n2095 = property on="Read1_in结果" class="Bool (严格)"("Colors [4]"=w24, "BoolText.Text"=w23) -> ()  [unwired: 2 in, 2 out]
  n2096 = property on="Clear_out结果" class="Bool (严格)"("Colors [4]"=w24, "BoolText.Text"=w23) -> ()  [unwired: 2 in, 2 out]
  n2097 = property on="Read2_in结果" class="Bool (严格)"("Colors [4]"=w24, "BoolText.Text"=w23) -> ()  [unwired: 2 in, 2 out]
  n2098 = property on="Set_in结果" class="Bool (严格)"("Colors [4]"=w24, "BoolText.Text"=w23) -> ()  [unwired: 2 in, 2 out]
  n2099 = property on="Current Gain结果 2" class="Bool (严格)"("Colors [4]"=w24, "BoolText.Text"=w23) -> ()  [unwired: 2 in, 2 out]
  "CAN连接状态" <- FALSE ("CAN连接状态")
  "CAN" <- FALSE ("CAN接收")
  "测试结果" <- TRUE ("测试结果")
  "Set" <- 0.0 ("电压/V")
  "Actual" <- 0.0 ("电流/A")
  "电流/A 4" <- 0.0 ("电流/A")
  "设定值 2" <- 0.0 ("电压/V")
  "实际值 2" <- w46
